vi "BRig_RT_start_v1,10__PortC.vi"() -> ()   [LabVIEW 2014]
uses:
  myRIO_BRig_RT__Case_Exp_stateList.ctl
  myRIO_BRig_RT__Case_NonExp_stateList.ctl
  <vilib>/WebDAVClient/Advanced/SessionHandle.ctl
  <vilib>/Platform/TimedLoop/XDataNode/timing_clust.ctl
  <vilib>/Platform/TimedLoop/XDataNode/nitl_modes.ctl
  <vilib>/Platform/TimedLoop/XDataNode/wakeup.ctl
  <vilib>/myRIO/Common/Instrument Driver Framework/myRIO v1.0/UART/vis/myRIO v1.0 Close UART.vi
  <vilib>/FPGAPlugInAG/myRIO-1900/niLvFpga_Open_myRIO-1900.vi
  <vilib>/rvi/interface/common/dynamic/niFpgaDynamicAddResources.vi
  <vilib>/Utility/error.llb/Error Cluster From Error Code.vi
  <vilib>/rvi/errors/niLvFpgaAdjustHostInterfaceError.vi
  <vilib>/Utility/file.llb/Read From Spreadsheet File (I64).vi
  <vilib>/Utility/file.llb/Write To Spreadsheet File (DBL).vi
  <vilib>/FPGAPlugInAG/Dynamic/niLvFpga_Close_Dynamic.vi
  <vilib>/myRIO/Common/Instrument Driver Framework/Utilities/vis/FPGA Ref Manager.vi
  <vilib>/myRIO/Common/Instrument Driver Framework/myRIO v1.0/myRIO v1.0 Reset FPGA.vi
  <vilib>/myRIO/Common/Instrument Driver Framework/myRIO v1.0/IRQ/vis/myRIO v1.0 IRQ Info FGV.vi
  <vilib>/myRIO/Common/Instrument Driver Framework/myRIO v1.0/IRQ/vis/myRIO v1.0 Timer IRQ Info FGV.vi
  <vilib>/myRIO/Common/Instrument Driver Framework/myRIO v1.0/IRQ/vis/myRIO v1.0 ISR Agent.vi
  <vilib>/rvi/interface/nirviOpenFPGA/nirviOpenFPGA.xnode
  BRig_FPGA_v3,93__PortC__build.lvbitx
  BRig_FPGA_v3,93__PortC.vi
  <vilib>/rvi/interface/nirviReadWriteControl/nirviReadWriteControl.xnode
  <vilib>/Platform/TimedLoop/XDataNode/XDataNode.xnode
  <vilib>/rvi/interface/nirviCloseFPGA/nirviCloseFPGA.xnode
  <vilib>/Platform/TimedLoop/XDataNode/XDNodeRunTimeDep.lvlib
  <vilib>/rvi/interface/Simulation/niFpgaSimulationCallBeginRW.vi
  <vilib>/myRIO/Instrument Drivers/Utilities/Utilities.lvlib
  NiFpgaLv.dll
  <vilib>/WebDAVClient/NI_WebDAV.lvlib
panel:
  out "Solenoid R":bool
  out "Solenoid L":bool
  out "Laser2":bool
  out "Laser1":bool
  out "FreeReward_c_R":u16
  out "FreeReward_c_L":u16
  in  "Laser2_LED":bool
  in  "Laser1_LED":bool
  in  "lick_Rising(F)_or_Falling(T)":bool
  out "T_ExpRun_min":dbl
  out "stop_TimedLoop":bool
  out "BTPR_avg_R":dbl
  out "T2R_avg_R":dbl
  out "BTPR_avg_L":dbl
  out "T2R_avg_L":dbl
  out "BTPR_block":u16
  out "T2R_block":u16
  in  "comm_WebDAV_connect":bool
  in  "I_sendData":bool
  in  "comm_TCP_connect":bool
  out "nRewards_total":u16 caption="# Rewards in Current Block"
  out "BUR_target":u16 caption="Target Trials Per Block"
  in  "input_Threshold_reset":bool
  out "nTrial":u16
  out "allReward_R":bool
  out "allReward_L":bool
  out "Threshold":bool
  out "tLoop":dbl format="%#_2g"
  out "L_Power_l2":dbl
  out "comm_TCP":bool
  in  "get_countPerMS":bool
  out "SolenoidReward":bool
  out "L_Power_l1":dbl caption="LaserPower"
  in  "Recording":bool
  out "FPGA_count2ms":dbl=159.0
  out "error out":errorcluster
  out "cSpout":enum16{"Left", "Right"}(ring) caption="Left or Right Spout"
  out "A4":u32 caption="LickCounter_Right"
  out "A2":u32 caption="LickCounter_Left"
  out "nRewards_Right":u16 caption="# Rewards Total (Right)"
  out "nRewards_Left":u16 caption="# Rewards Total (Left)"
  out "nRewards_cur":u16 caption="# Rewards in Current Block"
  out "TpB_target":u16 caption="Target Trials Per Block"
  out "cState_NonExp":T1 caption="WarmUp State"
  out "iBlock":u16 caption="Current Block"
  out "cState":T2 caption="Experimental State"
  out "iTrial":u16 caption="Current Trial"
  in  "Data Set Prefix":string="Exp1_TM2"
  out "comm_WebDAV":bool
  in  "Host Password":string="sabalab"
  in  "Host UserName":string="Test2"
  in  "STOP_abort":bool caption="Stop LabView\n(Stops myRio and FPGA)"
  in  "STOP_endBlock":bool caption="Stop Experiment\n@ End of Block"
  in  "STOP_endTrial":bool caption="Stop Experiment\n@ End of Trial"
  in  "START":bool caption="Start Experiment"
  # "Experimental Run"
  # "Recording Rig"
  # "FPGA Conversion\n[counts per ms]"
  # "RealTime Cycle\nShould be <5ms"
  # "STOP experiment at"
  # "Exp Run Time"
  # "Reset"
  # "min"
  # "Communication with Host"
  # "Lick Counter"
  # "Give Water?\n(Reward)"
  # "Experimental State"
  # "Left/Right"
  # "Left           Right"
  # "Direction\n(NonSpecific Licking)"
  # "Block Target"
  # "# Blocks"
  # "L          R"
  # "# Trials"
  # "# Rewards"
  # "Bad Trials\nPost Reward"
  # "Trials 2 Reward"
  # "Block"
  # "# Trials"
  # "# Rewards"
  # "Current\nBlock"
  # "WarmUp State"
  # "avg L"
  # "Total"
  # "# Rewards"
  # "# Trials"
  # "avg R"
  # "Laser Power [V]"
  # "Left           Right"
  # "FreeRewards"
  # "Laser1"
  # "Laser2"
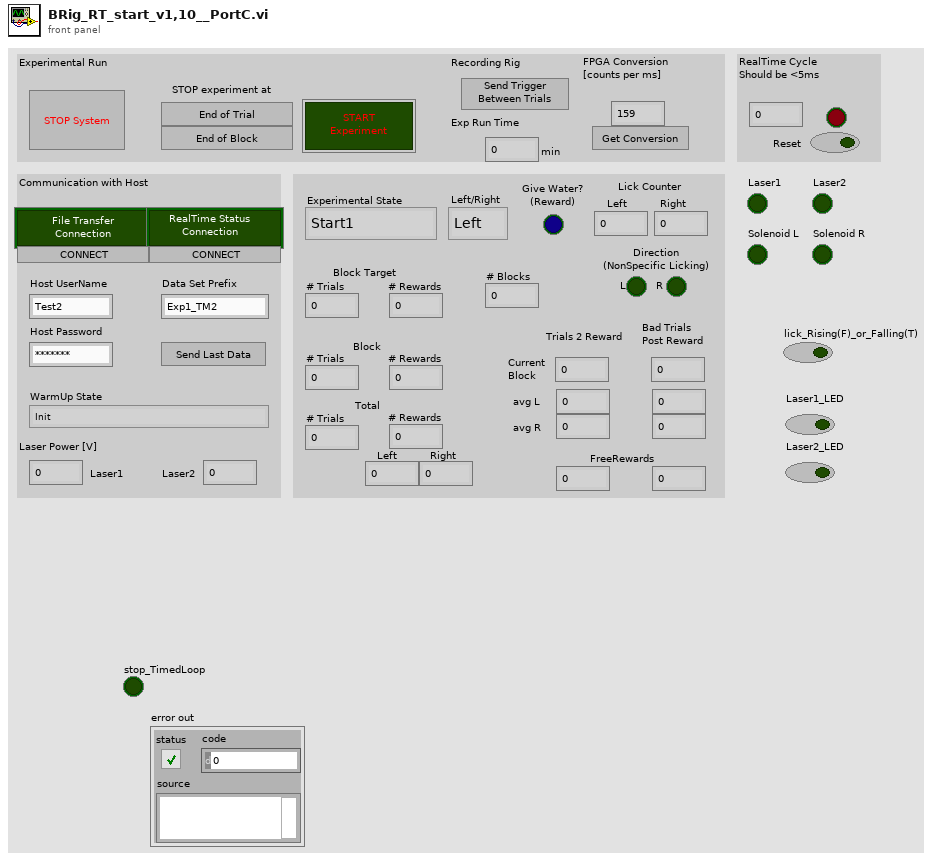
[diagram p1: front panel]
types:
  T1 = typedef "myRIO_BRig_RT__Case_NonExp_stateList.ctl" = enum16{"Init", "UploadSettings_pre", "UploadSettings_Read_dataExp", "UploadSettings_dataExp_1", "UploadSettings_dataExp_2", "UploadSettings_Read_dataLC", "UploadSettings_dataLC_1", "UploadSettings_dataLC_2", "UploadSettings_dataLC_3", "UploadSettings_dataLC_4", "UploadSettings_Read_dataMTrig", "UploadSettings_dataMTrig_1", "UploadSettings_post", "Idle_pre", "IdleEmpty", "IdleEmpty2", "IdleEmpty3", "IdleEmpty4", "Idle", "Idle_2", "Idle_3", "Idle_4", "Idle_5", "Idle_6", "Idle_post", "Cue_pre__pre", "Cue_pre", "Cue", "Cue_LED", "Cue_post", "RewardCalibration_pre", "RewardCalibration", "DispenseWater_pre__pre", "DispenseWater_pre", "DispenseWater", "DispenseWater_post", "TestConnection", "SendData", "Get_FPGA_count_per_ms", "End", "commTCP_connect"}
  T2 = typedef "myRIO_BRig_RT__Case_Exp_stateList.ctl" = enum16{"Start1", "Start2", "Start3", "saveSettings1", "saveSettings2", "saveSettings3", "saveSettings4", "saveSettings_LC_ENL_l1", "saveSettings_LC_ENL_l2", "saveSettings_LC_Cue_l1", "saveSettings_LC_Cue_l2", "saveSettings6_LC_l1_Other", "SaveSettings6_LC_l2_Other", "setSettings_Audio", "setSettings_Laser", "initBlock_pre", "initBlock", "initBlock2", "initBlock_post", "initTrial_pre", "initTrial", "initTrial2", "initTrial3", "initTrial4", "initTrial_LC_ENL1", "initTrial_LC_Cue1", "initTrial_LC_Cue1_2", "initTrial_LC_Sel", "initTrial_post", "ENL1_pre", "ENL1", "ENL1_post", "ENL1Penalty_pre", "ENL1Penalty", "ENL2_pre", "ENL2", "ENL2Penalty_pre", "ENL2Penalty", "Cue1_pre", "Cue1", "Cue1_post", "Cue1Penalty_pre", "Cue1Penalty", "Cue2_pre", "Cue2", "Cue2Penalty_pre", "Cue2Penalty", "Selection_pre", "Selection", "Select_post", "SelectReward_pre", "SelectReward", "SelectRewardPost_pre", "SelectRewardPost", "SelectWrong_pre", "SelectWrong", "SelectWrong_post", "SelectTimeout_pre", "SelectTimeout", "SelectTimeout_post", "endTrial_pre", "endTrial1", "endTrial2", "endTrial3", "endTrial_post", "endBlock_pre", "endBlock", "endBlock_post", "endExp", "commConnect", "commUpload_pre", "commUpload_dataBlock", "commUpload_dataCurrent", "commUpload_dataExp", "commUpload_dataLC", "commUpload_dataTrial", "commUpload_post", "saveData_pre", "saveData_dataBlock", "saveData_dataCurrent", "saveData_dataExp", "saveData_dataLC", "saveData_dataTrial", "saveData_post", "empty_endBlock1", "empty_endBlock2", "empty_endTrial1", "empty_endTrial2", "empty_endTrial3", "empty_endTrial4", "empty_endTrial5", "dummyState", "dummyState_endBlock", "FreeReward_pre", "FreeReward", "FreeRewardPost_pre", "FreeRewardPost"}
  T3 = enum8{"Enabled", "Disabled", "Disabled and Grayed Out"}
  T4 = typedef "NI_WebDAV.lvlib/SessionHandle.ctl" = refnum<k1>
  T5 = typedef "XDNodeRunTimeDep.lvlib/timing_clust.ctl" = cluster{"Expected End [f-1]":u64, "Actual End [f-1]":u64, "Finished Late? [f-1]":bool, "Expected End [i-1]":u64, "Actual End [i-1]":u64, "Finished Late? [i-1]":bool, "Expected Start [i]":u64, "Actual Start [i]":u64, "Expected Start [f]":u64, "Actual Start [f]":u64, "Source Name":string, "Structure Name":string, "Period":i64, "Deadline":i64, "Offset":i64, "Start":i64, "Priority":i32, "Timeout":i32, "Mode":T6, "Wakeup Reason":T7, "Error":errorcluster, "Source Type":string, "Secondary Source Type":string, "Global End Time":u64, "Global Start Time":u64, "Frame Duration":u64, "Iteration Duration":u64, "Assigned CPU":i32, "I/O Scan Engine Mode":u32}
  T6 = typedef "XDNodeRunTimeDep.lvlib/nitl_modes.ctl" = enum32{"No Change", "Process missed periods, maintain original phase", "Discard missed periods, maintain original phase", "Process missed periods, ignore original phase", "Discard missed periods, ignore original phase"}
  T7 = typedef "XDNodeRunTimeDep.lvlib/wakeup.ctl" = enum32{"Normal", "Aborted", "Asynchronous wakeup", "Timing source error", "Timed loop error", "Timeout"}
  T8 = cluster{"read mode":enum16{"polling", "blocking"}, "write mode":enum16{"polling", "blocking"}}
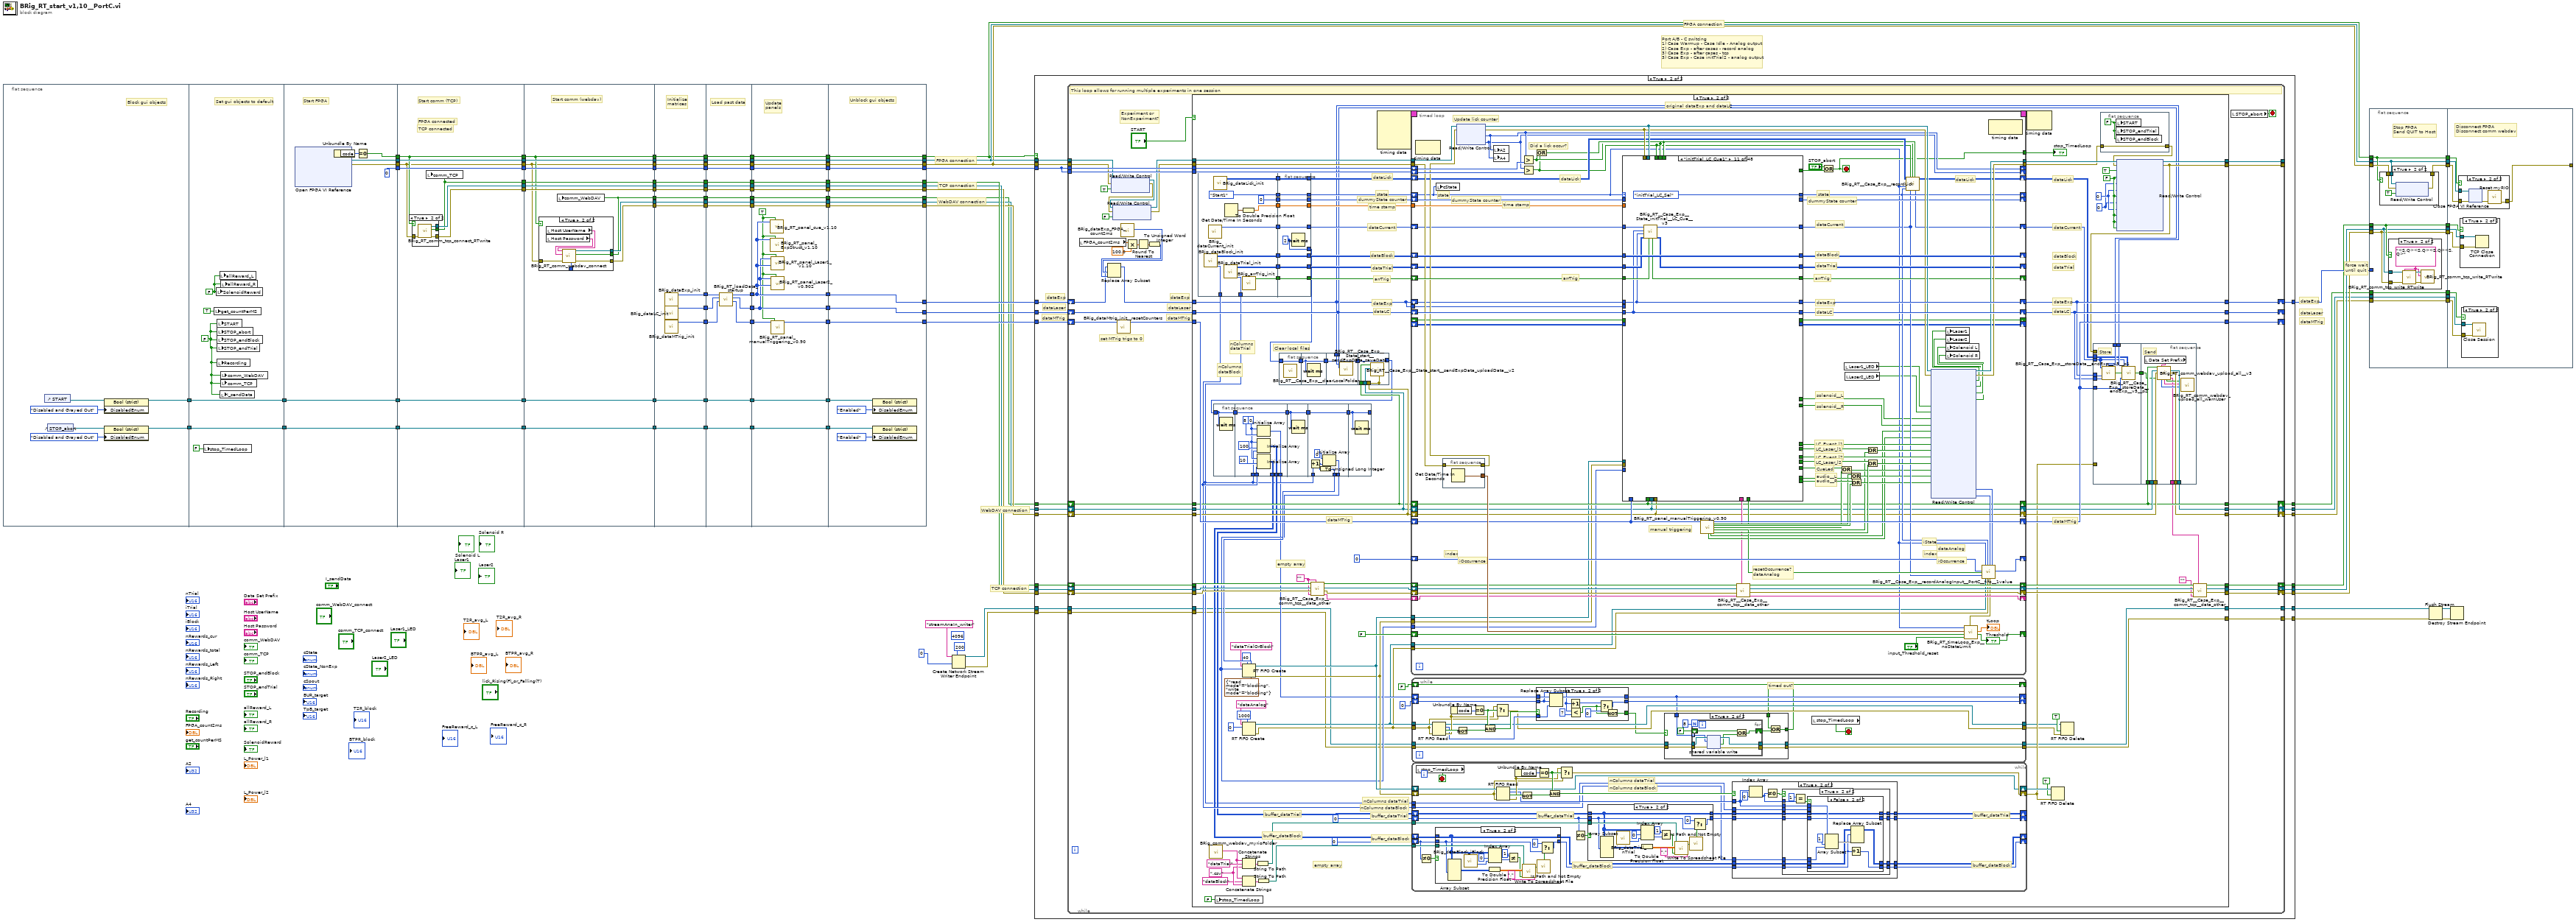
[diagram p0: block diagram]
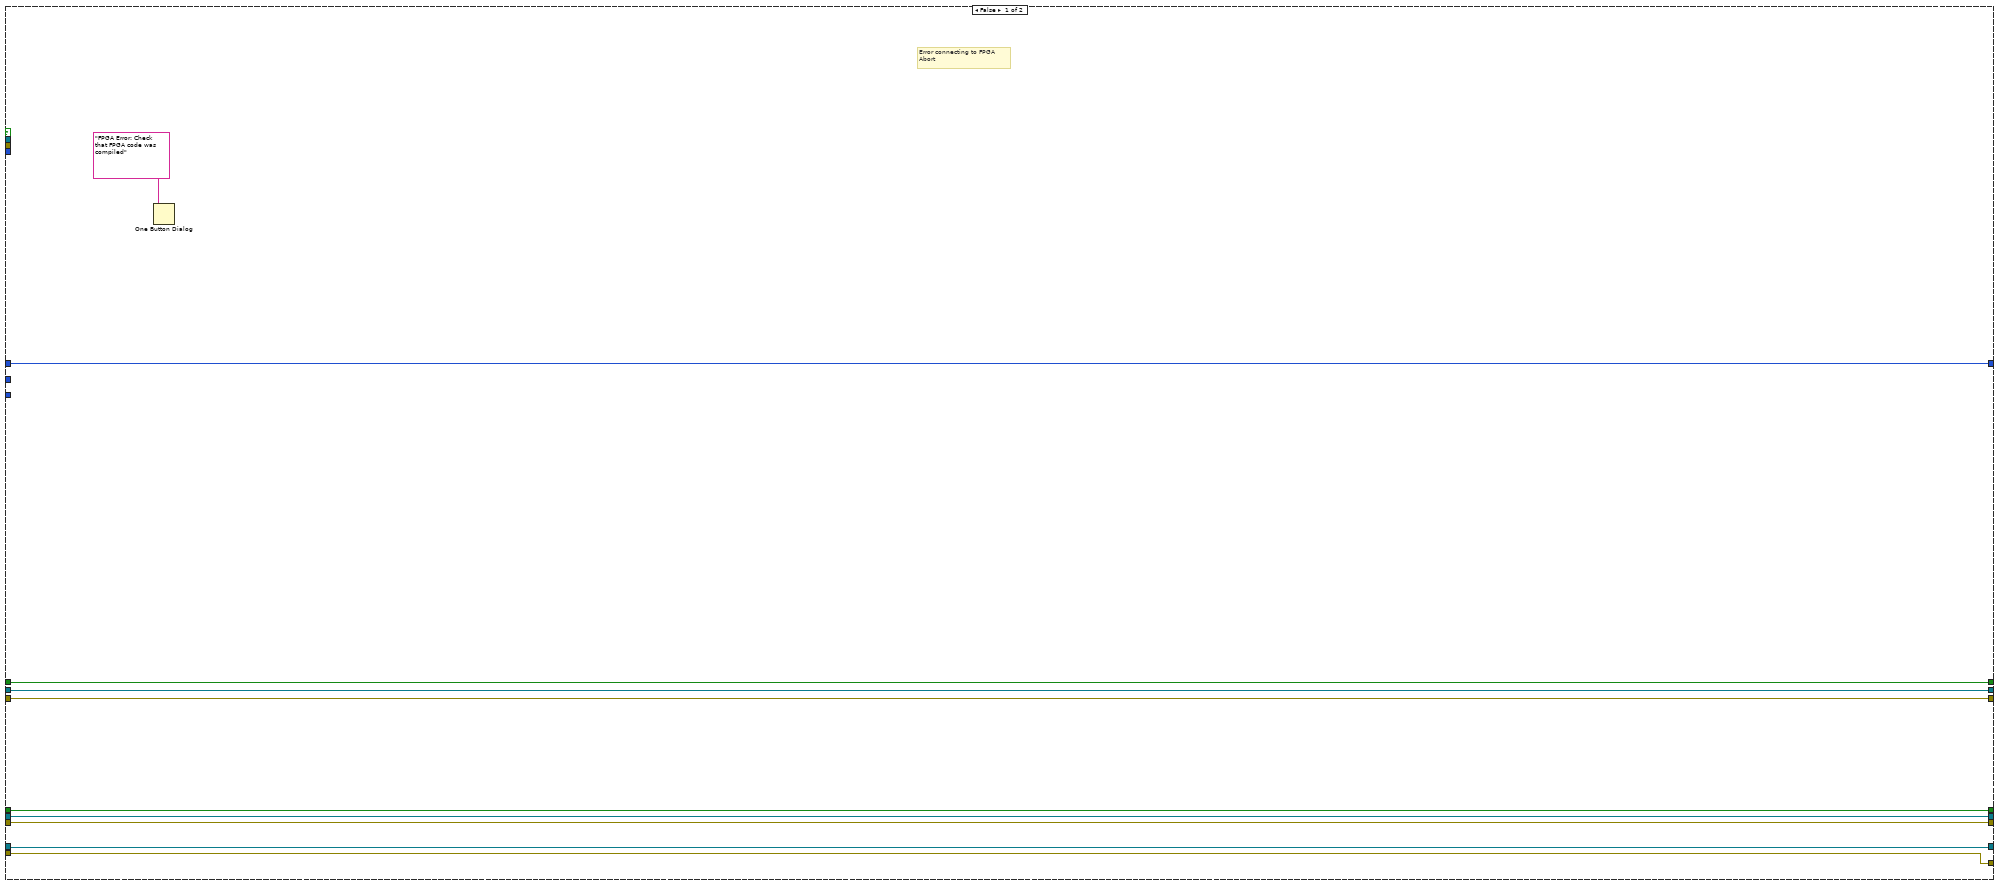
[diagram p2: hidden frame]
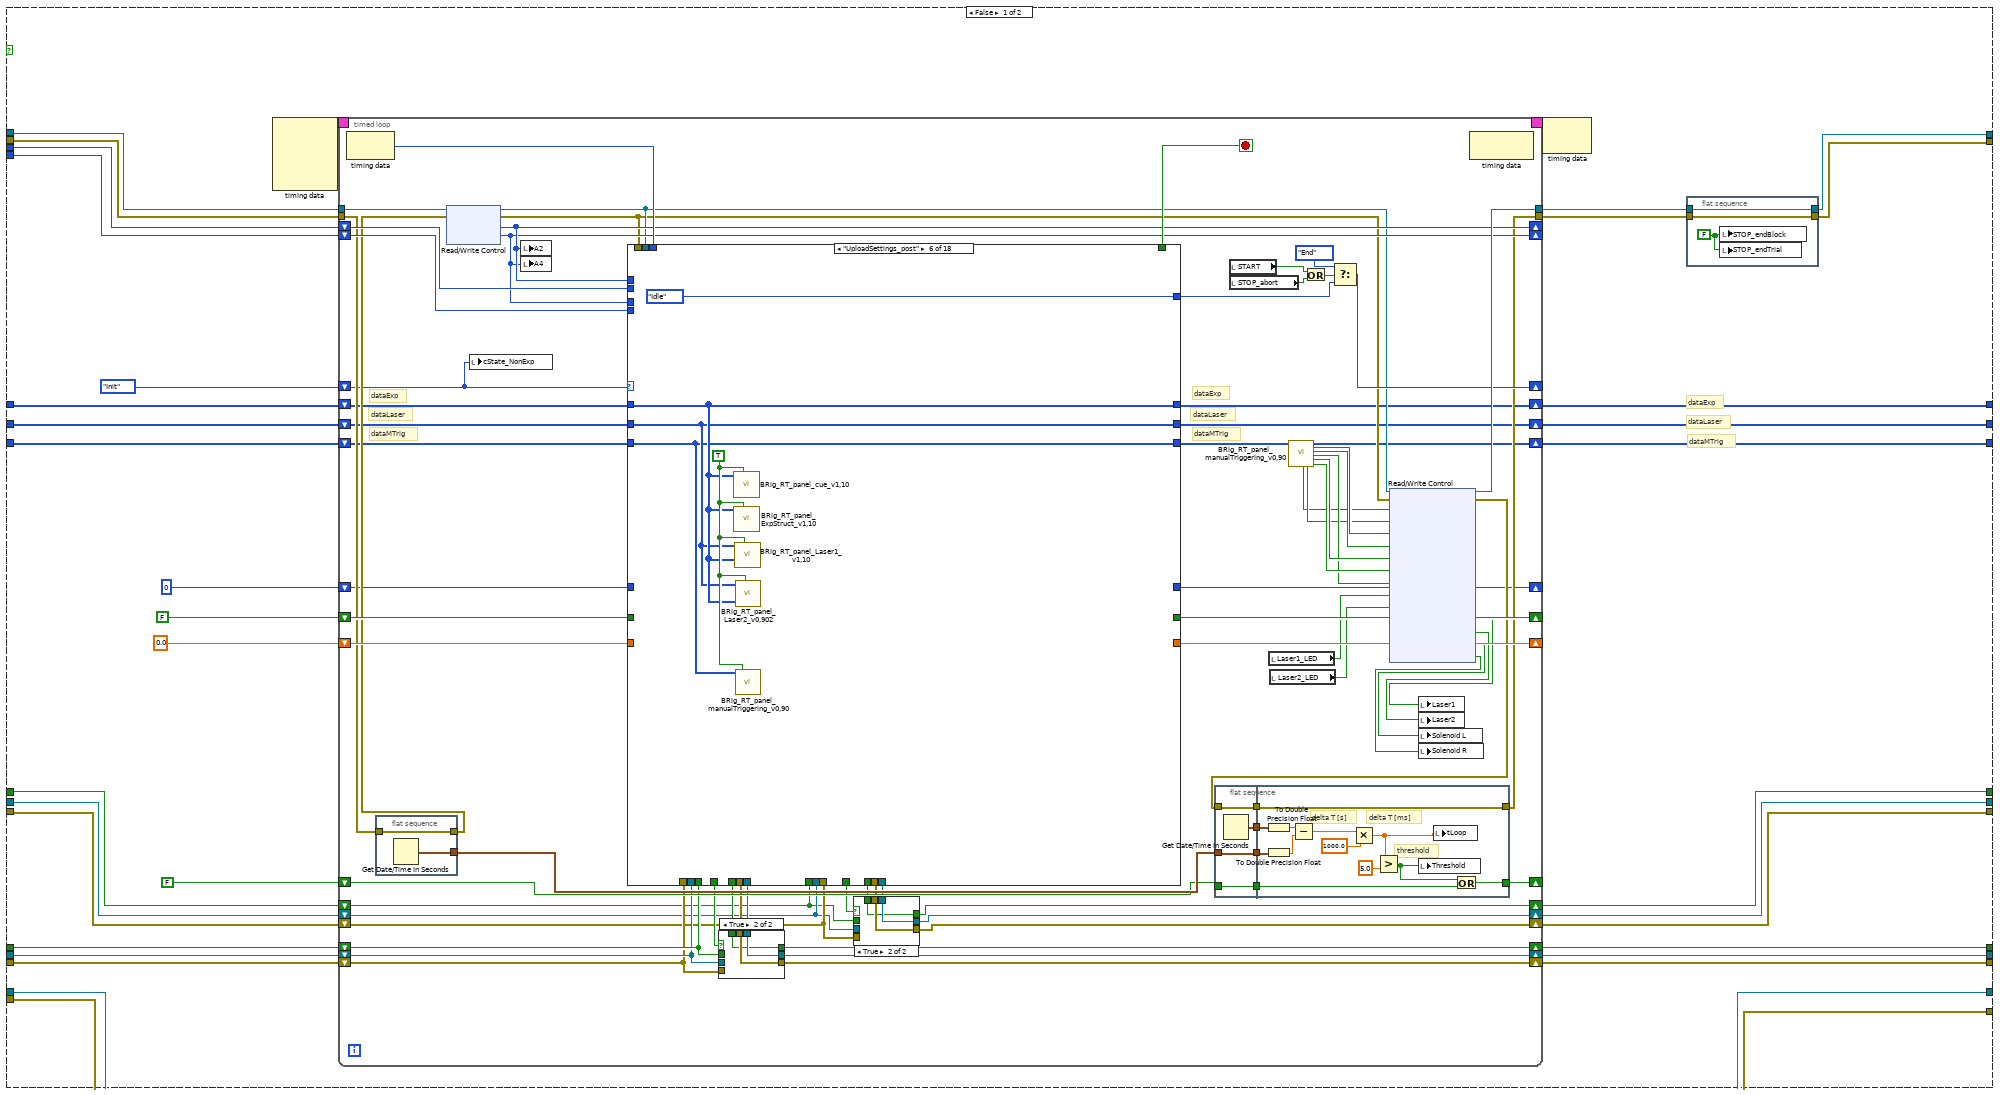
[diagram p3: hidden frame]
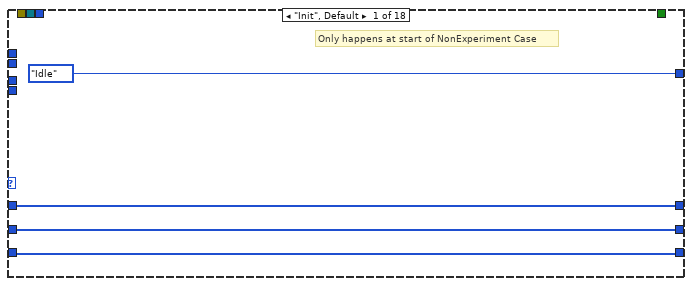
[diagram p6: hidden frame]
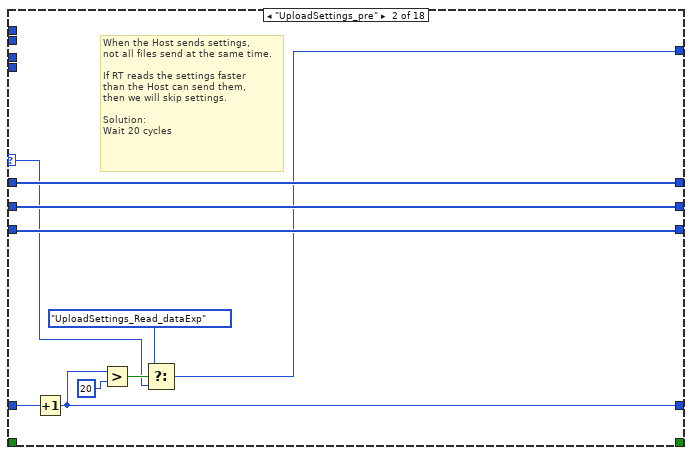
[diagram p7: hidden frame]
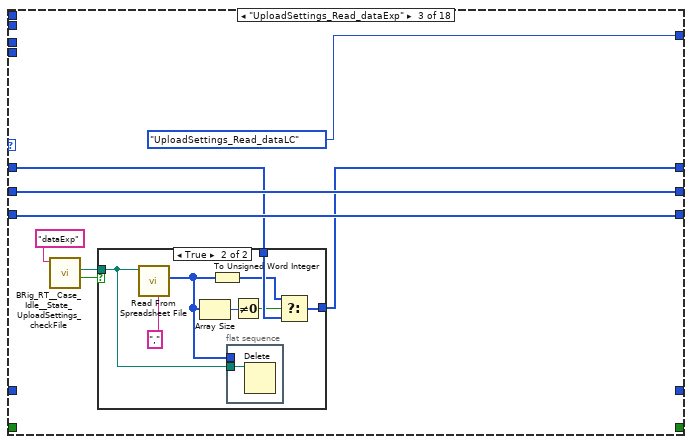
[diagram p8: hidden frame]
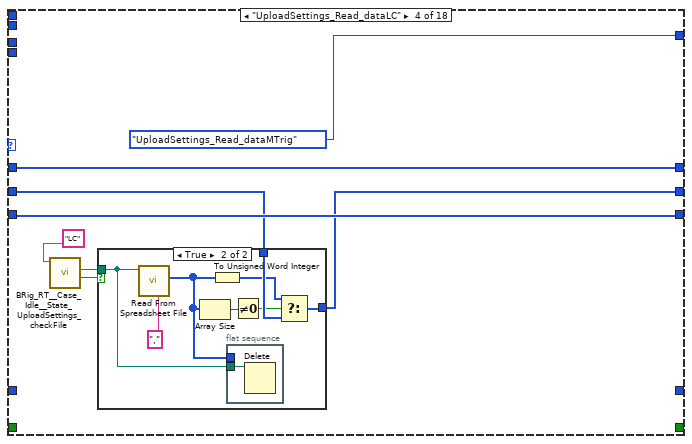
[diagram p10: hidden frame]
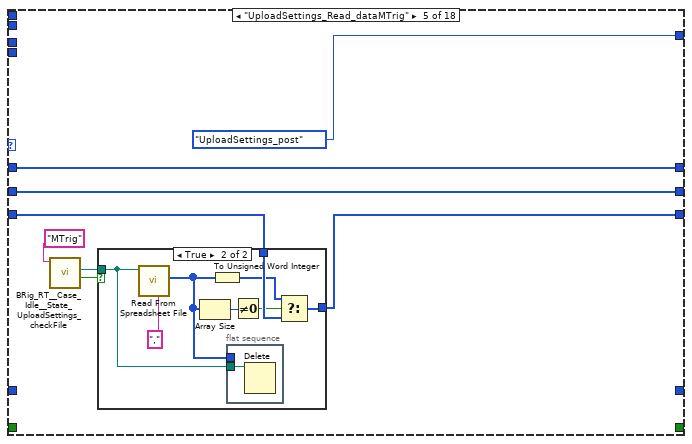
[diagram p12: hidden frame]
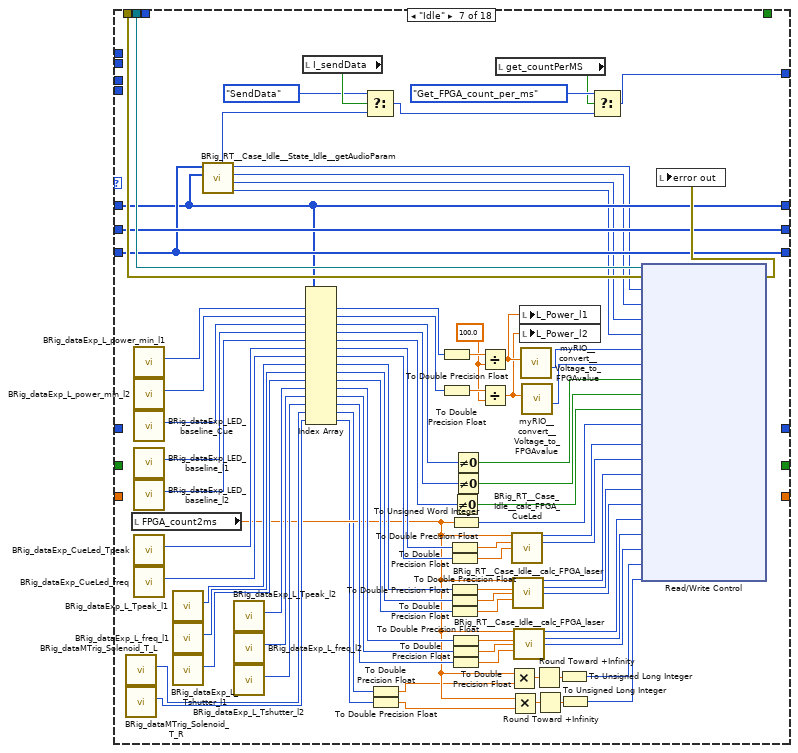
[diagram p14: hidden frame]
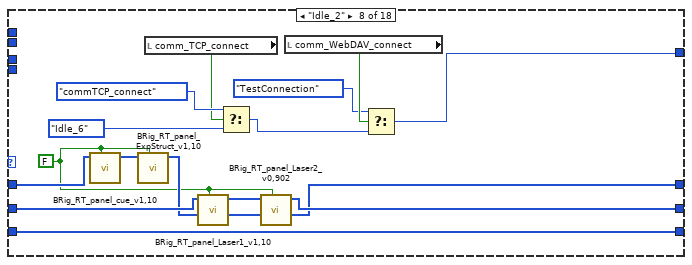
[diagram p15: hidden frame]
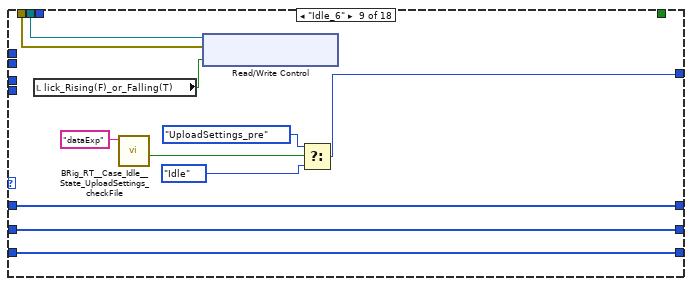
[diagram p16: hidden frame]
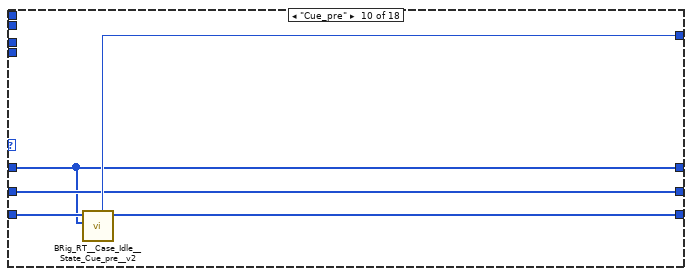
[diagram p17: hidden frame]
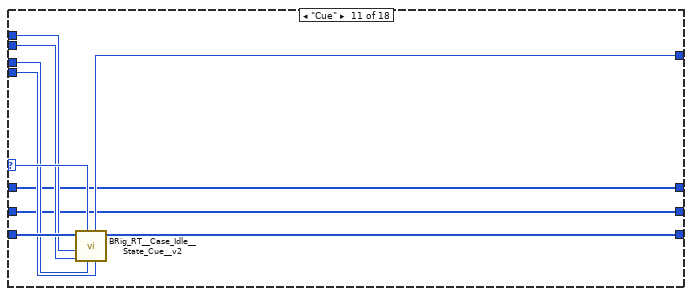
[diagram p18: hidden frame]
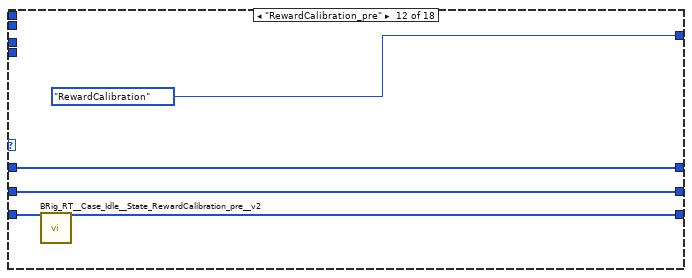
[diagram p19: hidden frame]
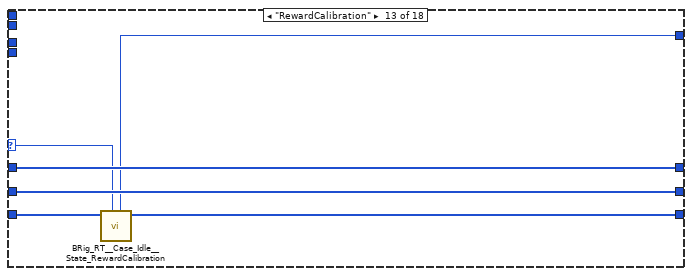
[diagram p20: hidden frame]
diagram:
  (unwired) 4096 ("reader buffer size")
  # "WebDAV connection"
  # "TCP connection"
  # "WebDAV connection"
  # "TCP connection"
  # "FPGA connection"
  # "FPGA connection"
  # "Port A/B - C switcing\n1) Case Warmup - Case Idle - Analog output\n2) Case Exp - after cases - record analog\n3) Case Exp - after cases - tcp\n3) Case Exp - Case initTrial2 - analog output"
  # "force wait\nuntil quit"
  # "dataLaser"
  # "dataExp"
  # "dataMTrig"
  n1 = flat-sequence {
    tunnel: [w116] -> w99
    tunnel: [w115] -> w95
    tunnel: [w125] -> w100
    tunnel: w99 -> [w125]
    tunnel: [w124] -> w96
    tunnel: w95 -> [w124]
    tunnel: [w131] -> w113
    tunnel: [w133] -> w112
    tunnel: [u32 0] -> w111
    tunnel: [w129] -> w110
    tunnel: [w128] -> w101
    tunnel: w100 -> [w128]
    tunnel: [w127] -> w97
    tunnel: w96 -> [w127]
    tunnel: w113 -> [w139]
    tunnel: w112 -> [w142]
    tunnel: w111 -> [w141]
    tunnel: w110 -> [w140]
    tunnel: [w139] -> w109
    tunnel: [w142] -> w108
    tunnel: [w141] -> w107
    tunnel: [w140] -> w106
    tunnel: [w134] -> w105
    tunnel: [w138] -> w104
    tunnel: [w137] -> w103
    tunnel: [w136] -> w102
    tunnel: w101 -> [w136]
    tunnel: [w135] -> w98
    tunnel: w97 -> [w135]
    tunnel: w109 -> [w153]
    tunnel: w108 -> [w161]
    tunnel: w107 -> [w160]
    tunnel: w106 -> [w154]
    tunnel: w105 -> [w159]
    tunnel: w104 -> [w158]
    tunnel: w103 -> [w157]
    tunnel: [w153] -> w66
    tunnel: [w161] -> w65
    tunnel: [w160] -> w64
    tunnel: [w154] -> w63
    tunnel: [w159] -> w62
    tunnel: [w158] -> w61
    tunnel: [w157] -> w60
    tunnel: [w156] -> w59
    tunnel: w102 -> [w156]
    tunnel: [w155] -> w58
    tunnel: w98 -> [w155]
    tunnel: [w152] -> w57
    tunnel: [w150] -> w56
    tunnel: [w151] -> w55
    tunnel: w66 -> [w186]
    tunnel: [w186] -> w54
    tunnel: w65 -> [w185]
    tunnel: [w185] -> w53
    tunnel: w64 -> [w184]
    tunnel: [w184] -> w52
    tunnel: w63 -> [w183]
    tunnel: [w183] -> w51
    tunnel: w62 -> [w182]
    tunnel: [w182] -> w50
    tunnel: w61 -> [w181]
    tunnel: [w181] -> w49
    tunnel: w60 -> [w180]
    tunnel: [w180] -> w48
    tunnel: w59 -> [w179]
    tunnel: [w179] -> w47
    tunnel: w58 -> [w178]
    tunnel: [w178] -> w46
    tunnel: w57 -> [w177]
    tunnel: [w177] -> w45
    tunnel: w56 -> [w176]
    tunnel: [w176] -> w44
    tunnel: w55 -> [w175]
    tunnel: [w175] -> w43
    tunnel: [w174] -> w42
    tunnel: [w173] -> w41
    tunnel: [w172] -> w40
    tunnel: w54 -> [w204]
    tunnel: [w204] -> w39
    tunnel: w53 -> [w203]
    tunnel: [w203] -> w37
    tunnel: w52 -> [w202]
    tunnel: [w202] -> w35
    tunnel: w51 -> [w201]
    tunnel: [w201] -> w33
    tunnel: w50 -> [w200]
    tunnel: [w200] -> w31
    tunnel: w49 -> [w199]
    tunnel: [w199] -> w29
    tunnel: w48 -> [w198]
    tunnel: [w198] -> w27
    tunnel: w47 -> [w197]
    tunnel: [w197] -> w25
    tunnel: w46 -> [w196]
    tunnel: [w196] -> w23
    tunnel: w45 -> [w195]
    tunnel: [w195] -> w21
    tunnel: w44 -> [w194]
    tunnel: [w194] -> w19
    tunnel: w43 -> [w193]
    tunnel: [w193] -> w17
    tunnel: w42 -> [w188]
    tunnel: [w187] -> w15
    tunnel: w41 -> [w190]
    tunnel: [w189] -> w13
    tunnel: w40 -> [w192]
    tunnel: [w191] -> w12
    tunnel: w39 -> [w221]
    tunnel: [w221] -> w38
    tunnel: w37 -> [w220]
    tunnel: [w220] -> w36
    tunnel: w35 -> [w219]
    tunnel: [w219] -> w34
    tunnel: w33 -> [w218]
    tunnel: [w218] -> w32
    tunnel: w31 -> [w217]
    tunnel: [w217] -> w30
    tunnel: w29 -> [w216]
    tunnel: [w216] -> w28
    tunnel: w27 -> [w215]
    tunnel: [w215] -> w26
    tunnel: w25 -> [w214]
    tunnel: [w214] -> w24
    tunnel: w23 -> [w213]
    tunnel: [w213] -> w22
    tunnel: w21 -> [w212]
    tunnel: [w212] -> w20
    tunnel: w19 -> [w211]
    tunnel: [w211] -> w18
    tunnel: w17 -> [w210]
    tunnel: [w210] -> w16
    tunnel: w15 -> [w207]
    tunnel: [w206] -> w14
    tunnel: w13 -> [w208]
    tunnel: w12 -> [w209]
    tunnel: [w209] -> w11
    tunnel: [w208] -> w10
    tunnel: [w228] -> w76
    tunnel: [w229] -> w77
    tunnel: [w230] -> w78
    tunnel: [w235] -> w82
    tunnel: [w236] -> w114
    tunnel: [w237] -> w89
    tunnel: [w238] -> w88
    tunnel: w38 -> [w238]
    tunnel: w36 -> [w237]
    tunnel: w34 -> [w236]
    tunnel: w32 -> [w235]
    tunnel: w30 -> [w230]
    tunnel: w28 -> [w229]
    tunnel: w26 -> [w228]
    tunnel: w24 -> [w232]
    tunnel: w22 -> [w231]
    tunnel: w20 -> [w226]
    tunnel: w18 -> [w227]
    tunnel: w16 -> [w225]
    tunnel: [w227] -> w70
    tunnel: [w226] -> w71
    tunnel: [w225] -> w72
    tunnel: [w222] -> w85
    tunnel: [w223] -> w84
    tunnel: [w224] -> w83
    tunnel: w14 -> [w224]
    tunnel: w11 -> [w222]
    tunnel: w10 -> [w223]
    frame #0 {
      # "Block gui objects"
      n2 = control-ref of="START"() -> (w120:refnum<vi>)
      n3 = control-ref of="STOP_abort"() -> (w117:refnum<vi>)
      n4 = property class="Bool (strict)"(reference=w120, "DisabledEnum"=T3."Disabled and Grayed Out" ("Disabled")) -> (reference out=w116:refnum<vi>)  [unwired: 1 in, 1 out]
      n5 = property class="Bool (strict)"(reference=w117, "DisabledEnum"=T3."Disabled and Grayed Out" ("Disabled")) -> (reference out=w115:refnum<vi>)  [unwired: 1 in, 1 out]
    }
    frame #1 {
      w122 = FALSE ("SolenoidReward")
      w123 = FALSE
      # "Set gui objects to default"
      n6 = local write "stop_TimedLoop"(FALSE ("stop_TimedLoop")) -> ()
      n7 = local write "get_countPerMS"(TRUE ("get_countPerMS")) -> ()
      n8 = local write "SolenoidReward"(w122) -> ()
      n9 = local write "START"(w123) -> ()
      n10 = local write "STOP_abort"(w123) -> ()
      n11 = local write "STOP_endBlock"(w123) -> ()
      n12 = local write "STOP_endTrial"(w123) -> ()
      n13 = local write "Recording"(w123) -> ()
      n14 = local write "allReward_L"(w122) -> ()
      n15 = local write "I_sendData"(w123) -> ()
      n16 = local write "comm_WebDAV"(w123) -> ()
      n17 = local write "comm_TCP"(w123) -> ()
      n18 = local write "allReward_R"(w122) -> ()
    }
    frame #2 {
      # "Start FPGA"
      n19 = xnode "Open FPGA VI Reference"() -> ("FPGA VI Reference Out"=w133:refnum<k20>, "error out"=w131:errorcluster)  [unwired: 2 in]
      n20 = Unbundle By Name(w131) -> ("code"=w130:i32)
      n21 = Equal To 0?(x=w130) -> (x = 0?=w129:bool)
    }
    frame #3 {
      # "TCP connected"
      # "Start comm (TCP)"
      # "FPGA connected"
      n22 = case shown="True" w140 {
        selector: w140 -> [w143 _]
        tunnel: w139 -> [w145 w149]
        tunnel: [refnum<k5> refnum ("output_hTCP") w148] -> w138
        tunnel: [w143 w147] -> w134
        tunnel: [w145 w146] -> w137
        frame False {
        }
        frame True {
          n23 = call "BRig_RT_comm_tcp_connect_RTwrite.vi"("input_error"=w149) -> ("output_error"=w146:errorcluster, "output_connected"=w147:bool, "output_hTCP"=w148:refnum<k5>)  [unwired: 8 in]
        }
      }
      n24 = local write "comm_TCP"(w134) -> ()
    }
    frame #4 {
      # "Start comm (webdav)"
      n25 = case shown="True" w154 {
        selector: w154 -> [w163 _]
        tunnel: [w162 w169] -> w152
        tunnel: [w163 w168] -> w150
        tunnel: w153 -> [w164 w167]
        tunnel: [w164 w166] -> w151
        tunnel: [_ w165] -> _
        frame False {
          w162 = T4 refnum items=["Session NI_WebDAV"] ("output_hSession")
        }
        frame True {
          n26 = local read "Host UserName"() -> (w170:string)
          n27 = local read "Host Password"() -> (w171:string)
          n28 = call "BRig_RT_comm_webdav_connect.vi"("input_error"=w167, "input_password"=w171, "input_username"=w170) -> ("output_error"=w166:errorcluster, "output_Iconnected"=w168:bool, "output_hSession"=w169:T4, "output_code"=w165:u8)  [unwired: 5 in]
        }
      }
      n29 = local write "comm_WebDAV"(w150) -> ()
    }
    frame #5 {
      # "Initialize\nmatrices"
      n30 = call "BRig_dataExp_init.vi"() -> ("output_dataExp"=w172:u16[])  [unwired: 11 in]
      n31 = call "BRig_dataLC_init.vi"() -> ("output_dataLC"=w173:u16[])  [unwired: 11 in]
      n32 = call "BRig_dataMTrig_init.vi"() -> ("output_dataMTrig"=w174:u16[])  [unwired: 5 in]
    }
    frame #6 {
      # "Load past data"
      n33 = call "BRig_RT_loadData_startup.vi"("input_dataMTrig"=w188, "input_dataLC"=w190, "input_dataExp"=w192) -> ("output_dataMTrig"=w187:u16[], "output_dataLC"=w189:u16[], "output_dataExp"=w191:u16[])  [unwired: 6 in]
    }
    frame #7 {
      w205 = TRUE ("input_setValues")
      # "Update\npanels"
      n34 = call "BRig_RT_panel_cue_v1,10.vi"("input_setValues"=w205, "input_dataExp"=w209) -> ()  [unwired: 9 in, 1 out]
      n35 = call "BRig_RT_panel_ExpStruct_v1,10.vi"("input_setValues"=w205, "input_dataExp"=w209) -> ()  [unwired: 9 in, 1 out]
      n36 = call "BRig_RT_panel_Laser1_v1,10.vi"("input_setValues"=w205, "input_dataExp"=w209, "input_dataLC"=w208) -> ()  [unwired: 7 in, 2 out]
      n37 = call "BRig_RT_panel_Laser2_v0,902.vi"("input_setValues"=w205, "input_dataExp"=w209, "input_dataLC"=w208) -> ()  [unwired: 7 in, 2 out]
      n38 = call "BRig_RT_panel_manualTriggering_v0,90.vi"("input_dataMTrig"=w207, "input_setValues"=w205) -> ("output_dataMTrig"=w206:u16[])  [unwired: 10 in, 7 out]
    }
    frame #8 {
      # "Unblock gui objects"
      n39 = property class="Bool (strict)"(reference=w232, "DisabledEnum"=T3."Enabled" ("Disabled")) -> ()  [unwired: 1 in, 2 out]
      n40 = property class="Bool (strict)"(reference=w231, "DisabledEnum"=T3."Enabled" ("Disabled")) -> ()  [unwired: 1 in, 2 out]
    }
  }
  n41 = Create Network Stream Writer Endpoint(7:200 ("reader buffer size"), 9:u16 0 ("element"), 11:"streamAnaIn_writer" ("reader name")) -> (0:w2:errorcluster, 3:w3:refnum<k21>)  [unwired: 4 in]
  n42 = case shown="True" w82 {
    tunnel: w114 -> [_ w271]
    tunnel: w89 -> [_ w270]
    tunnel: w88 -> [_ w269]
    tunnel: [w248 w268] -> w86
    tunnel: w85 -> [w248 w267]
    tunnel: w84 -> [_ w266]
    tunnel: w83 -> [_ w265]
    tunnel: w78 -> [w247 w264]
    tunnel: w77 -> [w246 w263]
    tunnel: w76 -> [w245 w262]
    tunnel: [w247 w261] -> w75
    tunnel: [w246 w260] -> w74
    tunnel: [w245 w259] -> w73
    tunnel: w72 -> [w244 w258]
    tunnel: w71 -> [w243 w257]
    tunnel: w70 -> [w242 w256]
    tunnel: [w244 w255] -> w69
    tunnel: [w243 w254] -> w68
    tunnel: [w242 w253] -> w67
    tunnel: [w241 w252] -> w7
    tunnel: [w240 w251] -> w6
    tunnel: w3 -> [w241 w250]
    tunnel: w2 -> [w240 w249]
    frame False {
      # "Error connecting to FPGA\nAbort"
      n43 = One Button Dialog(message="FPGA Error: Check that FPGA code was compiled") -> ()  [unwired: 1 in, 1 out]
    }
    frame True {
      # "dataExp"
      # "dataLaser"
      # "dataMTrig"
      n44 = while {
        tunnel: w270 -> [w305]
        tunnel: w269 -> [w310]
        tunnel: w271 -> [w313]
        tunnel: w271 -> [w312]
        tunnel: [w303] -> _
        tunnel: [w302] -> _
        shift-right: [w301] -> _
        shift-left: w265 -> [w297]
        shift-right: [w299] -> _
        shift-left: w266 -> [w300]
        shift-right: [w298] -> w268
        shift-left: w267 -> [w277]
        shift-right: [w292] -> w261
        shift-left: w264 -> [w295]
        shift-right: [w291] -> w260
        shift-left: w263 -> [w294]
        shift-right: [w290] -> w259
        shift-left: w262 -> [w293]
        shift-right: [w286] -> w255
        shift-left: w258 -> [w289]
        shift-right: [w285] -> w254
        shift-left: w257 -> [w288]
        shift-right: [w284] -> w253
        shift-left: w256 -> [w287]
        tunnel: [w275] -> w252
        tunnel: [w274] -> w251
        tunnel: w250 -> [w273]
        tunnel: w249 -> [w272]
        stop <- w311 stop-if-true
        # "set MTrig trigs to 0"
        # "dataExp"
        # "dataLaser"
        # "dataMTrig"
        # "Experiment or\nNonExperiment?"
        # "This loop allows for running multiple experiments in one session"
        n45 = local read "FPGA_count2ms"() -> (w281:dbl)
        n46 = xnode "Read/Write Control"("FPGA VI Reference In"=w305, "error in"=w310, "Counts_Reset"=TRUE) -> ("FPGA VI Reference Out"=w307:refnum<k20>, "error out"=w308:errorcluster)
        n47 = xnode "Read/Write Control"("FPGA VI Reference In"=w307, "error in"=w308, "Counts_Reset"=FALSE) -> ("FPGA VI Reference Out"=w304:refnum<k20>, "error out"=w306:errorcluster)
        n48 = call "BRig_dataMtrig_init__resetCounters.vi"("input_dataMTrig"=w297) -> ("output_dataMTrig"=w296:u16[])  [unwired: 10 in]
        n49 = call "BRig_dataExp_FPGA_count2ms.vi"() -> ("output_FPGA_count2ms"=w282:i32)  [unwired: 11 in]
        n50 = Multiply(x=w281, y=100.0) -> (x*y=w279:dbl)
        n51 = Round To Nearest(number=w279) -> (nearest integer value=w278:dbl)
        n52 = To Unsigned Word Integer(number=w278) -> (unsigned 16bit integer=w283:u16)
        n53 = Replace Array Subset(array=w277, new element=w283, index=w282) -> (w276:u16[])
        n54 = case shown="True" "START" {
          tunnel: w313 -> [w347 w914]
          tunnel: w312 -> [w346 w913]
          tunnel: w306 -> [w344 w902]
          tunnel: w304 -> [w345 w903]
          tunnel: [w342 w911] -> w303
          tunnel: [w340 w880] -> w302
          tunnel: w296 -> [w336 w900]
          tunnel: [w335 w886] -> w301
          tunnel: w300 -> [w334 w850]
          tunnel: w276 -> [w333 w801]
          tunnel: [w332 w885] -> w299
          tunnel: [w331 w884] -> w298
          tunnel: w295 -> [w330 w894]
          tunnel: w294 -> [w329 w893]
          tunnel: w293 -> [w328 w892]
          tunnel: [w327 w869] -> w292
          tunnel: [w326 w868] -> w291
          tunnel: [w325 w867] -> w290
          tunnel: w289 -> [w324 w849]
          tunnel: w288 -> [w323 w848]
          tunnel: w287 -> [w322 w847]
          tunnel: [w321 w876] -> w286
          tunnel: [w320 w875] -> w285
          tunnel: [w319 w877] -> w284
          tunnel: w273 -> [w317 w806]
          tunnel: w272 -> [w316 w805]
          tunnel: [w317 w804] -> w275
          tunnel: [w316 w803] -> w274
          frame False {
            # "dataExp"
            # "dataLaser"
            # "dataMTrig"
            n55 = node-c288() -> (w350:T5)  [unwired: 4 in]
            n56 = timed-loop {
              timing: w350 -> [_]
              timing-out: [_] -> w349
              shift-right: [w418] -> _
              shift-left: myRIO_BRig_RT__Case_NonExp_stateList."Init" ("Enum") -> [w387]
              shift-right: [w416] -> _
              shift-left: w347 -> [w417]
              shift-right: [w414] -> _
              shift-left: w346 -> [w415]
              tunnel: [w424] -> w343
              tunnel: [w400] -> w341
              tunnel: w344 -> [w407]
              tunnel: w345 -> [w425]
              shift-right: [w410] -> _
              shift-left: FALSE -> [w411]
              shift-right: [w408] -> _
              shift-left: 0.0 -> [w409]
              shift-right: [w397] -> _
              shift-left: FALSE -> [w398]
              shift-right: [w396] -> w335
              shift-left: w336 -> [w388]
              shift-right: [w382] -> w331
              shift-left: w333 -> [w385]
              shift-right: [w383] -> w332
              shift-left: w334 -> [w384]
              shift-right: [w381] -> w327
              shift-left: w330 -> [w377]
              shift-right: [w380] -> w326
              shift-left: w329 -> [w376]
              shift-right: [w379] -> w325
              shift-left: w328 -> [w375]
              shift-right: [w365] -> w321
              shift-left: w324 -> [w371]
              shift-right: [w366] -> w320
              shift-left: w323 -> [w370]
              shift-right: [w367] -> w319
              shift-left: w322 -> [w369]
              shift-right: [w360] -> _
              shift-left: u16 0 ("y") -> [w361]
              stop <- w427 stop-if-true
              # "dataExp"
              # "dataLaser"
              # "dataExp"
              # "dataLaser"
              # "dataMTrig"
              # "dataMTrig"
              n57 = node-c288() -> (w426:i64)  [unwired: 1 in]
              n58 = flat-sequence {
                tunnel: w407 -> [w456]
                tunnel: [w457] -> w399
                tunnel: [w456] -> w406
                frame #0 {
                  n59 = Get Date/Time In Seconds() -> (seconds since 1Jan1904=w457:timestamp)
                }
              }
              n60 = xnode "Read/Write Control"("FPGA VI Reference In"=w425, "error in"=w406) -> ("FPGA VI Reference Out"=w413:refnum<k20>, "error out"=w412:errorcluster, "A2_LickL"=w416:u32, "A4_LickR"=w414:u32)
              n61 = local write "cState_NonExp"(w387) -> ()
              n62 = local write "A2"(w416) -> ()
              n63 = local write "A4"(w414) -> ()
              n64 = case shown="\"UploadSettings_post\"" w387 {
                selector: w387 -> [_ w464 _ _ _ _ _ _ _ _ w655 _ w663 _ _ w707 w750 w756]
                tunnel: [myRIO_BRig_RT__Case_NonExp_stateList."Idle" ("Enum") w465 myRIO_BRig_RT__Case_NonExp_stateList."UploadSettings_Read_dataLC" ("t") myRIO_BRig_RT__Case_NonExp_stateList."UploadSettings_Read_dataMTrig" ("t") myRIO_BRig_RT__Case_NonExp_stateList."UploadSettings_post" ("t") myRIO_BRig_RT__Case_NonExp_stateList."Idle" ("t") w546 w614 w638 w644 w653 myRIO_BRig_RT__Case_NonExp_stateList."RewardCalibration" ("Enum") w662 myRIO_BRig_RT__Case_NonExp_stateList."Idle" ("Enum") myRIO_BRig_RT__Case_NonExp_stateList."Idle" ("Enum") w706 w750 w757] -> w419
                tunnel: [w460 w471 w479 w497 w511 w526 w558 w630 w636 w645 w654 w657 w664 w678 w690 w716 w748 w765] -> w386
                tunnel: [_ _ _ _ _ _ _ _ _ _ _ _ _ _ _ _ TRUE _] -> w427
                tunnel: w388 -> [w460 w471 w479 w497 w508 w526 w558 w630 w636 w646 w656 w658 w665 w678 w690 w716 w748 w765]
                tunnel: w426 -> [_ _ _ _ _ _ _ _ _ _ _ _ _ _ _ _ _ _]
                tunnel: w417 -> [_ _ _ _ _ _ _ _ _ _ w651 _ _ _ _ _ _ _]
                tunnel: w416 -> [_ _ _ _ _ _ _ _ _ _ w652 _ _ _ _ _ _ _]
                tunnel: w415 -> [_ _ _ _ _ _ _ _ _ _ w649 _ _ _ _ _ _ _]
                tunnel: w414 -> [_ _ _ _ _ _ _ _ _ _ w650 _ _ _ _ _ _ _]
                tunnel: w413 -> [_ _ _ _ _ _ w613 _ w633 _ _ _ _ _ _ w711 _ _]
                tunnel: w412 -> [_ _ _ _ _ _ w612 _ w632 _ _ _ _ _ _ w710 _ _]
                tunnel: w411 -> [_ _ _ _ _ _ _ _ _ _ _ _ _ _ _ w715 _ _]
                tunnel: [_ _ _ _ _ _ _ _ _ _ _ _ _ _ _ TRUE _ _] -> w410
                tunnel: w409 -> [_ _ _ _ _ _ _ _ _ _ _ _ _ _ _ w713 _ _]
                tunnel: [_ _ _ _ _ _ _ _ _ _ _ _ _ _ _ w712 _ _] -> w408
                tunnel: w385 -> [w458 w469 w474 w496 w515 w528 w557 w628 w634 w642 w647 w660 w666 w675 w687 w703 w746 w763]
                tunnel: w384 -> [w459 w470 w478 w490 w512 w527 w559 w627 w635 w643 w648 w659 w667 w676 w688 w704 w747 w764]
                tunnel: [w459 w470 w478 w493 w512 w527 w559 w623 w635 w643 w648 w659 w667 w676 w688 w704 w747 w764] -> w383
                tunnel: [w458 w469 w473 w496 w515 w528 w557 w620 w634 w642 w647 w660 w666 w675 w687 w703 w746 w763] -> w382
                tunnel: [_ _ _ _ _ _ _ _ _ _ _ _ _ _ _ _ _ TRUE] -> w378
                tunnel: w377 -> [_ _ _ _ _ _ _ _ _ _ _ _ _ _ w681 _ _ w762]
                tunnel: w376 -> [_ _ _ _ _ _ _ _ _ _ _ _ _ _ w683 _ _ w758]
                tunnel: w375 -> [_ _ _ _ _ _ _ _ _ _ _ _ _ _ w682 _ _ w761]
                tunnel: [_ _ _ _ _ _ _ _ _ _ _ _ _ _ _ _ _ w760] -> w374
                tunnel: [_ _ _ _ _ _ _ _ _ _ _ _ _ _ _ _ _ w759] -> w373
                tunnel: [_ _ _ _ _ _ _ _ _ _ _ _ _ _ _ _ _ w751] -> w372
                tunnel: w369 -> [_ _ _ _ _ _ _ _ _ _ _ _ _ _ w680 _ _ _]
                tunnel: w370 -> [_ _ _ _ _ _ _ _ _ _ _ _ _ _ w686 _ _ _]
                tunnel: w371 -> [_ _ _ _ _ _ _ _ _ _ _ _ _ w668 w685 _ _ _]
                tunnel: [_ _ _ _ _ _ _ _ _ _ _ _ _ TRUE _ _ _ _] -> w368
                tunnel: [_ _ _ _ _ _ _ _ _ _ _ _ _ w670 _ _ _ _] -> w364
                tunnel: [_ _ _ _ _ _ _ _ _ _ _ _ _ w668 _ _ _ _] -> w363
                tunnel: [_ _ _ _ _ _ _ _ _ _ _ _ _ w669 _ _ _ _] -> w362
                tunnel: w361 -> [_ w463 _ _ _ _ _ _ _ _ _ _ _ _ _ _ _ _]
                tunnel: [_ w462 _ _ _ _ _ _ _ _ _ _ _ _ _ _ _ _] -> w360
                frame "Init", Default {
                  # "Only happens at start of NonExperiment Case"
                }
                frame "UploadSettings_pre" {
                  # "When the Host sends settings,\nnot all files send at the same time.\n\nIf RT reads the settings faster\nthan the Host can send them,\nthen we will skip settings.\n\nSolution:\nWait 20 cycles"
                  n65 = Increment(x=w463) -> (x+1=w462:u16)
                  n66 = Greater?(x=w462, y=u16 20) -> (0:w467:bool)
                  n67 = Select(t=myRIO_BRig_RT__Case_NonExp_stateList."UploadSettings_Read_dataExp", s=w467, f=w464) -> (s? t:f=w465:T1)
                }
                frame "UploadSettings_Read_dataExp" {
                  n68 = call "BRig_RT__Case_Idle__State_UploadSettings_checkFile.vi"("input_dataName"="dataExp") -> ("output_Iexist"=w476:bool, "output_dataPath"=w475:path)  [unwired: 9 in]
                  n69 = case shown="True" w476 {
                    tunnel: w475 -> [_ w482]
                    tunnel: w474 -> [w480 w486]
                    tunnel: [w480 w484] -> w473
                    frame False {
                    }
                    frame True {
                      n70 = call-poly <vilib>:"Read From Spreadsheet File.vi"("delimiter (\\t)"="," ("delimiter (\\t)"), "file path (dialog if empty)"=w482) -> ("first row"=w481:i64[])  [unwired: 5 in, 4 out]
                      n71 = Array Size(array=w481) -> (size(s)=w487:i32)
                      n72 = To Unsigned Word Integer(number=w481) -> (unsigned 16bit integer=w485:u16[])
                      n73 = flat-sequence {
                        tunnel: w482 -> [w489]
                        tunnel: w481 -> [_]
                        frame #0 {
                          n74 = Delete(path (use dialog)=w489) -> ()  [unwired: 4 in, 3 out]
                        }
                      }
                      n75 = Not Equal To 0?(x=w487) -> (x != 0?=w483:bool)
                      n76 = Select(t=w485, s=w483, f=w486) -> (s? t:f=w484:u16[])
                    }
                  }
                }
                frame "UploadSettings_Read_dataLC" {
                  n77 = call "BRig_RT__Case_Idle__State_UploadSettings_checkFile.vi"("input_dataName"="LC") -> ("output_Iexist"=w491:bool, "output_dataPath"=w492:path)  [unwired: 9 in]
                  n78 = case shown="True" w491 {
                    tunnel: w492 -> [_ w500]
                    tunnel: w490 -> [w498 w504]
                    tunnel: [w498 w502] -> w493
                    frame False {
                    }
                    frame True {
                      n79 = call-poly <vilib>:"Read From Spreadsheet File.vi"("delimiter (\\t)"="," ("delimiter (\\t)"), "file path (dialog if empty)"=w500) -> ("first row"=w499:i64[])  [unwired: 5 in, 4 out]
                      n80 = Array Size(array=w499) -> (size(s)=w505:i32)
                      n81 = To Unsigned Word Integer(number=w499) -> (unsigned 16bit integer=w503:u16[])
                      n82 = flat-sequence {
                        tunnel: w500 -> [w507]
                        tunnel: w499 -> [_]
                        frame #0 {
                          n83 = Delete(path (use dialog)=w507) -> ()  [unwired: 4 in, 3 out]
                        }
                      }
                      n84 = Not Equal To 0?(x=w505) -> (x != 0?=w501:bool)
                      n85 = Select(t=w503, s=w501, f=w504) -> (s? t:f=w502:u16[])
                    }
                  }
                }
                frame "UploadSettings_Read_dataMTrig" {
                  n86 = call "BRig_RT__Case_Idle__State_UploadSettings_checkFile.vi"("input_dataName"="MTrig") -> ("output_Iexist"=w509:bool, "output_dataPath"=w510:path)  [unwired: 9 in]
                  n87 = case shown="True" w509 {
                    tunnel: w510 -> [_ w518]
                    tunnel: w508 -> [w516 w522]
                    tunnel: [w516 w520] -> w511
                    frame False {
                    }
                    frame True {
                      n88 = call-poly <vilib>:"Read From Spreadsheet File.vi"("delimiter (\\t)"="," ("delimiter (\\t)"), "file path (dialog if empty)"=w518) -> ("first row"=w517:i64[])  [unwired: 5 in, 4 out]
                      n89 = Array Size(array=w517) -> (size(s)=w523:i32)
                      n90 = To Unsigned Word Integer(number=w517) -> (unsigned 16bit integer=w521:u16[])
                      n91 = flat-sequence {
                        tunnel: w518 -> [w525]
                        tunnel: w517 -> [_]
                        frame #0 {
                          n92 = Delete(path (use dialog)=w525) -> ()  [unwired: 4 in, 3 out]
                        }
                      }
                      n93 = Not Equal To 0?(x=w523) -> (x != 0?=w519:bool)
                      n94 = Select(t=w521, s=w519, f=w522) -> (s? t:f=w520:u16[])
                    }
                  }
                }
                frame "UploadSettings_post" {
                  w529 = TRUE ("input_setValues")
                  n95 = call "BRig_RT_panel_cue_v1,10.vi"("input_setValues"=w529, "input_dataExp"=w528) -> ()  [unwired: 9 in, 1 out]
                  n96 = call "BRig_RT_panel_ExpStruct_v1,10.vi"("input_setValues"=w529, "input_dataExp"=w528) -> ()  [unwired: 9 in, 1 out]
                  n97 = call "BRig_RT_panel_Laser1_v1,10.vi"("input_setValues"=w529, "input_dataExp"=w528, "input_dataLC"=w527) -> ()  [unwired: 7 in, 2 out]
                  n98 = call "BRig_RT_panel_Laser2_v0,902.vi"("input_setValues"=w529, "input_dataExp"=w528, "input_dataLC"=w527) -> ()  [unwired: 7 in, 2 out]
                  n99 = call "BRig_RT_panel_manualTriggering_v0,90.vi"("input_dataMTrig"=w526, "input_setValues"=w529) -> ()  [unwired: 10 in, 8 out]
                }
                frame "Idle" {
                  w603 = 100.0 ("y")
                  n100 = call "BRig_dataMTrig_Solenoid_T_L.vi"() -> ("output_Solenoid_T_L"=w541:i32)  [unwired: 11 in]
                  n101 = call "BRig_dataMTrig_Solenoid_T_R.vi"() -> ("output_Solenoid_T_R"=w540:i32)  [unwired: 11 in]
                  n102 = local read "FPGA_count2ms"() -> (w539:dbl)
                  n103 = call "BRig_dataExp_L_power_min_l1.vi"() -> ("output_L_power_min_l1"=w608:i32)  [unwired: 11 in]
                  n104 = call "BRig_dataExp_L_power_min_l2.vi"() -> ("output_L_power_min_l2"=w607:i32)  [unwired: 11 in]
                  n105 = call "BRig_dataExp_LED_baseline_Cue.vi"() -> ("output_LED_baseline_Cue"=w601:i32)  [unwired: 11 in]
                  n106 = call "BRig_dataExp_LED_baseline_l1.vi"() -> ("output_LED_baseline_l1"=w600:i32)  [unwired: 11 in]
                  n107 = call "BRig_dataExp_LED_baseline_l2.vi"() -> ("output_LED_baseline_l2"=w599:i32)  [unwired: 11 in]
                  n108 = call "BRig_dataExp_CueLed_Tpeak.vi"() -> ("output_CueLed_Tpeak"=w591:i32)  [unwired: 11 in]
                  n109 = call "BRig_dataExp_CueLed_freq.vi"() -> ("output_CueLed_Freq"=w590:i32)  [unwired: 11 in]
                  n110 = call "BRig_dataExp_L_Tpeak_l1.vi"() -> ("output_L_Tpeak_l1"=w583:i32)  [unwired: 11 in]
                  n111 = call "BRig_dataExp_L_freq_l1.vi"() -> ("output_L_freq_l1"=w582:i32)  [unwired: 11 in]
                  n112 = call "BRig_dataExp_L_Tshutter_l1.vi"() -> ("output_L_Tshutter_l1"=w581:i32)  [unwired: 11 in]
                  n113 = call "BRig_RT__Case_Idle__State_Idle__getAudioParam.vi"("input_dataExp"=w557, "input_dataMTrig"=w558) -> ("output_Audio_freq_R"=w553:u8, "output_Audio_amp_R"=w554:u16, "output_Audio_freq_L"=w555:u8, "output_Audio_amp_L"=w556:u16, "output_state"=w552:T1)  [unwired: 5 in]
                  n114 = call "BRig_dataExp_L_Tpeak_l2.vi"() -> ("output_L_Tpeak_l2"=w565:i32)  [unwired: 11 in]
                  n115 = call "BRig_dataExp_L_freq_l2.vi"() -> ("output_L_freq_l2"=w564:i32)  [unwired: 11 in]
                  n116 = call "BRig_dataExp_L_Tshutter_l2.vi"() -> ("output_L_Tshutter_l2"=w563:i32)  [unwired: 11 in]
                  n117 = local read "I_sendData"() -> (w551:bool)
                  n118 = Index Array(array=w557, index #1=w608, index #2=w607, index #3=w601, index #4=w600, index #5=w599, index #6=w591, index #7=w590, index #8=w583, index #9=w582, index #10=w581, index #11=w565, index #12=w564, index #13=w563, index #14=w541, index #15=w540) -> (element #1=w606:u16, element #2=w602:u16, element #3=w598:u16, element #4=w597:u16, element #5=w596:u16, element #6=w587:u16, element #7=w586:u16, element #8=w580:u16, element #9=w579:u16, element #10=w578:u16, element #11=w568:u16, element #12=w567:u16, element #13=w566:u16, element #14=w538:u16, element #15=w537:u16)
                  n119 = Select(t=myRIO_BRig_RT__Case_NonExp_stateList."SendData" ("Enum"), s=w551, f=w552) -> (s? t:f=w548:T1)
                  n120 = To Double Precision Float(number=w538) -> (double precision float=w536:dbl)
                  n121 = To Double Precision Float(number=w537) -> (double precision float=w535:dbl)
                  n122 = To Double Precision Float(number=w606) -> (double precision float=w605:dbl)
                  n123 = To Double Precision Float(number=w602) -> (double precision float=w604:dbl)
                  n124 = To Double Precision Float(number=w587) -> (double precision float=w589:dbl)
                  n125 = To Double Precision Float(number=w586) -> (double precision float=w588:dbl)
                  n126 = To Double Precision Float(number=w580) -> (double precision float=w577:dbl)
                  n127 = To Double Precision Float(number=w579) -> (double precision float=w576:dbl)
                  n128 = To Double Precision Float(number=w578) -> (double precision float=w575:dbl)
                  n129 = To Unsigned Word Integer(number=w539) -> (unsigned 16bit integer=w592:u16)
                  n130 = To Double Precision Float(number=w568) -> (double precision float=w569:dbl)
                  n131 = To Double Precision Float(number=w567) -> (double precision float=w570:dbl)
                  n132 = To Double Precision Float(number=w566) -> (double precision float=w571:dbl)
                  n133 = Not Equal To 0?(x=w596) -> (x != 0?=w593:bool)
                  n134 = Not Equal To 0?(x=w598) -> (x != 0?=w595:bool)
                  n135 = Not Equal To 0?(x=w597) -> (x != 0?=w594:bool)
                  n136 = Divide(x=w605, y=w603) -> (x/y=w532:dbl)
                  n137 = Divide(x=w604, y=w603) -> (x/y=w531:dbl)
                  n138 = local read "get_countPerMS"() -> (w547:bool)
                  n139 = Multiply(x=w539, y=w536) -> (x*y=w545:dbl)
                  n140 = Multiply(x=w539, y=w535) -> (x*y=w543:dbl)
                  n141 = call "BRig_RT__Case_Idle__calc_FPGA_CueLed.vi"("input_FPGA_ms2count"=w539, "input_Tpeak"=w589, "input_Freq"=w588) -> ("output_laser_Npeak"=w585:u32, "output_laser_Nvalley"=w584:u32)  [unwired: 11 in]
                  n142 = call "BRig_RT__Case_Idle__calc_FPGA_laser.vi"("input_FPGA_ms2count"=w539, "input_Tpeak"=w577, "input_Freq"=w576, "input_Tshutter"=w575) -> ("output_laser_Npeak"=w574:u32, "output_laser_Nvalley"=w573:u32, "output_laser_Nshutter"=w572:u32)  [unwired: 9 in]
                  n143 = call "BRig_RT__Case_Idle__calc_FPGA_laser.vi"("input_FPGA_ms2count"=w539, "input_Tpeak"=w569, "input_Freq"=w570, "input_Tshutter"=w571) -> ("output_laser_Npeak"=w562:u32, "output_laser_Nvalley"=w561:u32, "output_laser_Nshutter"=w560:u32)  [unwired: 9 in]
                  n144 = local write "L_Power_l1"(w532) -> ()
                  n145 = local write "L_Power_l2"(w531) -> ()
                  n146 = call "myRIO__convert__Voltage_to_FPGAvalue.vi"("input_voltage"=w532) -> ("output_PortC"=w609:i16)  [unwired: 9 in, 1 out]
                  n147 = call "myRIO__convert__Voltage_to_FPGAvalue.vi"("input_voltage"=w531) -> ("output_PortC"=w610:i16)  [unwired: 9 in, 1 out]
                  n148 = Round Toward +Infinity(x=w545) -> (ceil(x): smallest int >= x=w544:dbl)
                  n149 = Round Toward +Infinity(x=w543) -> (ceil(x): smallest int >= x=w542:dbl)
                  n150 = To Unsigned Long Integer(number=w544) -> (unsigned 32bit integer=w534:u32)
                  n151 = To Unsigned Long Integer(number=w542) -> (unsigned 32bit integer=w533:u32)
                  n152 = Select(t=myRIO_BRig_RT__Case_NonExp_stateList."Get_FPGA_count_per_ms" ("Enum"), s=w547, f=w548) -> (s? t:f=w546:T1)
                  n153 = xnode "Read/Write Control"("FPGA VI Reference In"=w613, "error in"=w612, "audioAmp_L"=w556, "audioFreq_L_kHz"=w555, "audioAmp_R"=w554, "audioFreq_R_kHz"=w553, "AnaOut_0"=w609, "AnaOut_1"=w610, "CueLed_Baseline"=w595, "L1Led_Baseline"=w594, "L2Led_Baseline"=w593, "k1__counter_per_ms"=w592, "CueLed_nPeak"=w585, "CueLed_nValley"=w584, "LC_nPeak_l1"=w574, "LC_nValley_l1"=w573, "LC_nShutter_l1"=w572, "LC_nPeak_l2"=w562, "LC_nValley_l2"=w561, "LC_nShutter_l2"=w560, "Solenoid_nTotal_L"=w534, "Solenoid_nTotal_R"=w533) -> ("error out"=w611:errorcluster)  [unwired: 1 out]
                  n154 = local write "error out"(w611) -> ()
                }
                frame "Idle_2" {
                  w619 = FALSE
                  n155 = call "BRig_RT_panel_cue_v1,10.vi"("input_setValues"=w619, "input_dataExp"=w628) -> ("output_dataExp"=w629:u16[])  [unwired: 9 in]
                  n156 = call "BRig_RT_panel_ExpStruct_v1,10.vi"("input_setValues"=w619, "input_dataExp"=w629) -> ("output_dataExp"=w622:u16[])  [unwired: 9 in]
                  n157 = local read "comm_TCP_connect"() -> (w618:bool)
                  n158 = call "BRig_RT_panel_Laser1_v1,10.vi"("input_setValues"=w619, "input_dataExp"=w622, "input_dataLC"=w627) -> ("output_dataExp"=w621:u16[], "output_dataLC"=w624:u16[])  [unwired: 7 in]
                  n159 = Select(t=myRIO_BRig_RT__Case_NonExp_stateList."commTCP_connect" ("Enum"), s=w618, f=myRIO_BRig_RT__Case_NonExp_stateList."Idle_6" ("Enum")) -> (s? t:f=w616:T1)
                  n160 = call "BRig_RT_panel_Laser2_v0,902.vi"("input_setValues"=w619, "input_dataExp"=w621, "input_dataLC"=w624) -> ("output_dataExp"=w620:u16[], "output_dataLC"=w623:u16[])  [unwired: 7 in]
                  n161 = local read "comm_WebDAV_connect"() -> (w617:bool)
                  n162 = Select(t=myRIO_BRig_RT__Case_NonExp_stateList."TestConnection" ("Enum"), s=w617, f=w616) -> (s? t:f=w614:T1)
                }
                frame "Idle_6" {
                  n163 = local read "lick_Rising(F)_or_Falling(T)"() -> (w631:bool)
                  n164 = call "BRig_RT__Case_Idle__State_UploadSettings_checkFile.vi"("input_dataName"="dataExp") -> ("output_Iexist"=w640:bool)  [unwired: 9 in, 1 out]
                  n165 = xnode "Read/Write Control"("FPGA VI Reference In"=w633, "error in"=w632, "Rising(F)_or_Falling(T)"=w631) -> ()  [unwired: 2 out]
                  n166 = Select(t=myRIO_BRig_RT__Case_NonExp_stateList."UploadSettings_pre" ("Enum"), s=w640, f=myRIO_BRig_RT__Case_NonExp_stateList."Idle") -> (s? t:f=w638:T1)
                }
                frame "Cue_pre" {
                  n167 = call "BRig_RT__Case_Idle__State_Cue_pre__v2.vi"("input_dataExp"=w642, "input_dataMTrig"=w646) -> ("output_dataMTrig"=w645:u16[], "output_state"=w644:T1)  [unwired: 8 in]
                }
                frame "Cue" {
                  n168 = call "BRig_RT__Case_Idle__State_Cue__v2.vi"("input_cLick_R_prev"=w649, "input_cLick_R"=w650, "input_state"=w655, "input_cLick_L_prev"=w651, "input_cLick_L"=w652, "input_dataMTrig"=w656) -> ("output_dataMTrig"=w654:u16[], "output_state"=w653:T1)  [unwired: 4 in]
                }
                frame "RewardCalibration_pre" {
                  n169 = call "BRig_RT__Case_Idle__State_RewardCalibration_pre__v2.vi"("input_dataMTrig"=w658) -> ("output_dataMTrig"=w657:u16[])  [unwired: 26 in]
                }
                frame "RewardCalibration" {
                  n170 = call "BRig_RT__Case_Idle__State_RewardCalibration.vi"("input_state"=w663, "input_dataMTrig"=w665) -> ("output_dataMtrig"=w664:u16[], "output_state"=w662:T1)  [unwired: 8 in]
                }
                frame "TestConnection" {
                  n171 = local read "Host Password"() -> (w671:string)
                  n172 = local read "Host UserName"() -> (w672:string)
                  n173 = call "BRig_RT_comm_webdav_connect.vi"("input_password"=w671, "input_username"=w672) -> ("output_Iconnected"=w670:bool, "output_hSession"=w669:T4)  [unwired: 6 in, 2 out]
                  n174 = local write "comm_WebDAV_connect"(FALSE ("comm_WebDAV_connect")) -> ()
                  n175 = local write "comm_WebDAV"(w670) -> ()
                }
                frame "SendData" {
                  n176 = And(x=w681, y=w680) -> (x .and. y?=w679:bool)
                  n177 = case shown="True" w679 {
                    tunnel: w680 -> [_ w698]
                    tunnel: w686 -> [_ w697]
                    tunnel: w685 -> [_ w696]
                    tunnel: w683 -> [_ w694]
                    tunnel: w682 -> [_ w693]
                    frame False {
                      n178 = One Button Dialog(message="Unable to send data:\n Missing one or more\n connections") -> ()  [unwired: 1 in, 1 out]
                    }
                    frame True {
                      n179 = local read "Data Set Prefix"() -> (w699:string)
                      n180 = call "BRig_RT_comm_webdav_upload_all__v3.vi"("input_I_connected_webdav"=w698, "input_fileName_prefix"=w699, "input_hSession"=w697, "input_error"=w696, "input_True"=TRUE) -> ("output_nFilenames"=w700:i32, "output_arrFilenames"=w701:string[], "output_uploaded"=w702:bool[], "output_strCmd"=w695:string)  [unwired: 5 in, 2 out]
                      n181 = call "BRig_RT_comm_tcp_write_RTwrite.vi"("input_error"=w693, "input_packet"=w695, "input_hTCP"=w694) -> ()  [unwired: 5 in, 4 out]
                      n182 = call "BRig_RT_comm_webdav_upload_all_warnUser.vi"("input_n"=w700, "input_arrFilenames"=w701, "input_arrUploaded"=w702) -> ()  [unwired: 9 in]
                    }
                  }
                  n183 = local write "I_sendData"(FALSE ("I_sendData")) -> ()
                }
                frame "Get_FPGA_count_per_ms" {
                  # "Used to automatically determine how many FPGA cycles in 1 ms"
                  n184 = case shown="True" w715 {
                    selector: w715 -> [w717 _]
                    tunnel: w713 -> [_ w730]
                    tunnel: [w721 w730] -> w712
                    tunnel: w711 -> [w720 w728]
                    tunnel: w710 -> [w719 w727]
                    tunnel: [w718 w725] -> w705
                    tunnel: [w717 w724] -> w709
                    frame False {
                      n185 = Get Date/Time In Seconds() -> (seconds since 1Jan1904=w722:timestamp)
                      n186 = To Double Precision Float(number=w722) -> (double precision float=w721:dbl)
                      n187 = xnode "Read/Write Control"("FPGA VI Reference In"=w720, "error in"=w719, "timeTrial_trig"=TRUE ("timeTrial")) -> ("error out"=w718:errorcluster)  [unwired: 1 out]
                      n188 = local write "get_countPerMS"(w717) -> ()
                    }
                    frame True {
                      w726 = 1.0
                      n189 = Get Date/Time In Seconds() -> (seconds since 1Jan1904=w731:timestamp)
                      n190 = To Double Precision Float(number=w731) -> (double precision float=w732:dbl)
                      n191 = Subtract(x=w732, y=w730) -> (x-y=w729:dbl)
                      n192 = Less Or Equal?(x=w726, y=w729) -> (x <= y?=w724:bool)
                      n193 = case shown="True" w724 {
                        tunnel: w728 -> [_ w745]
                        tunnel: w727 -> [w733 w744]
                        tunnel: w726 -> [_ w735]
                        tunnel: [w733 w734] -> w725
                        frame False {
                        }
                        frame True {
                          n194 = xnode "Read/Write Control"("FPGA VI Reference In"=w745, "error in"=w744) -> ("FPGA VI Reference Out"=w742:refnum<k20>, "error out"=w741:errorcluster, "timeTrial_count"=w736:u32)
                          n195 = Multiply(x=w735, y=1000.0) -> (x*y=w739:dbl)
                          n196 = To Double Precision Float(number=w736) -> (double precision float=w738:dbl)
                          n197 = Divide(x=w738, y=w739) -> (x/y=w740:dbl)
                          n198 = local write "FPGA_count2ms"(w740) -> ()
                          n199 = xnode "Read/Write Control"("FPGA VI Reference In"=w742, "error in"=w741, "timeTrial_trig"=FALSE ("timeTrial")) -> ("error out"=w734:errorcluster)  [unwired: 1 out]
                        }
                      }
                    }
                  }
                  n200 = Select(t=myRIO_BRig_RT__Case_NonExp_stateList."Idle" ("Enum"), s=w709, f=w707) -> (s? t:f=w706:T1)
                  n201 = local write "error out"(w705) -> ()
                }
                frame "End" {
                }
                frame "commTCP_connect" {
                  n202 = local read "comm_TCP_connect"() -> (w755:bool)
                  n203 = case shown="True" w762 {
                    tunnel: w761 -> [w772 w781]
                    tunnel: [w771 w777] -> w759
                    tunnel: [w770 w774] -> w751
                    tunnel: [w769 w775] -> w760
                    tunnel: w758 -> [_ w782]
                    frame False {
                      n204 = call "BRig_RT_comm_tcp_connect_RTwrite.vi"("input_error"=w772) -> ("output_error"=w769:errorcluster, "output_connected"=w770:bool, "output_hTCP"=w771:refnum<k5>)  [unwired: 8 in]
                    }
                    frame True {
                      n205 = call "BRig_RT_comm_tcp_write_RTwrite.vi"("input_error"=w781, "input_packet"="<test>", "input_hTCP"=w782) -> ("output_error"=w776:errorcluster, "output_I_NotDisconnected"=w773:bool, "output_I_write"=w779:bool, "output_hTCP"=w778:refnum<k5>)  [unwired: 5 in]
                      n206 = case shown="False" w779 {
                        selector: w779 -> [_ w793]
                        tunnel: w778 -> [w788 w795]
                        tunnel: [w783 w795] -> w777
                        tunnel: w776 -> [w787 w794]
                        tunnel: [w785 w794] -> w775
                        tunnel: [w784 w793] -> w774
                        tunnel: w773 -> [w789 _]
                        frame False {
                          n207 = case shown="True" w789 {
                            tunnel: w788 -> [_ w792]
                            tunnel: w787 -> [w790 w791]
                            tunnel: [w790 w791] -> w786
                            frame False {
                            }
                            frame True {
                              n208 = TCP Close Connection(connection ID=w792, error in (no error)=w791) -> ()  [unwired: 1 in, 2 out]
                            }
                          }
                          n209 = call "BRig_RT_comm_tcp_connect_RTwrite.vi"("input_error"=w786) -> ("output_error"=w785:errorcluster, "output_connected"=w784:bool, "output_hTCP"=w783:refnum<k5>)  [unwired: 8 in]
                        }
                        frame True {
                        }
                      }
                    }
                  }
                  n210 = Not(x=w755) -> (.not. x?=w754:bool)
                  n211 = Or(x=w754, y=w751) -> (x .or. y?=w753:bool)
                  n212 = case shown="True" w753 {
                    tunnel: [w766 myRIO_BRig_RT__Case_NonExp_stateList."Idle" ("Enum")] -> w757
                    tunnel: w756 -> [w766 _]
                    frame False {
                    }
                    frame True {
                      n213 = local write "comm_TCP_connect"(FALSE) -> ()
                    }
                  }
                  n214 = local write "comm_TCP"(w751) -> ()
                }
              }
              n215 = case shown="True" w378 {
                tunnel: [w436 w437] -> w381
                tunnel: [w435 w438] -> w380
                tunnel: [w434 w439] -> w379
                tunnel: w377 -> [w436 _]
                tunnel: w376 -> [w435 _]
                tunnel: w375 -> [w434 _]
                tunnel: w374 -> [_ w439]
                tunnel: w373 -> [_ w438]
                tunnel: w372 -> [_ w437]
                frame False {
                }
                frame True {
                }
              }
              n216 = case shown="True" w368 {
                tunnel: [w430 w431] -> w367
                tunnel: [w429 w432] -> w366
                tunnel: [w428 w433] -> w365
                tunnel: w369 -> [w430 _]
                tunnel: w370 -> [w429 _]
                tunnel: w371 -> [w428 _]
                tunnel: w363 -> [_ w433]
                tunnel: w362 -> [_ w432]
                tunnel: w364 -> [_ w431]
                frame False {
                }
                frame True {
                }
              }
              n217 = flat-sequence {
                tunnel: w401 -> [w443]
                tunnel: w399 -> [w441]
                tunnel: [w443] -> w405
                tunnel: [w442] -> w404
                tunnel: [w441] -> w403
                tunnel: [w440] -> w402
                tunnel: w398 -> [w440]
                tunnel: [w455] -> w400
                tunnel: w405 -> [w455]
                tunnel: w404 -> [w454]
                tunnel: w403 -> [w452]
                tunnel: w402 -> [w447]
                tunnel: [w446] -> w397
                frame #0 {
                  n218 = Get Date/Time In Seconds() -> (seconds since 1Jan1904=w442:timestamp)
                }
                frame #1 {
                  # "threshold"
                  # "delta T [ms]"
                  # "delta T [s]"
                  n219 = To Double Precision Float(number=w454) -> (double precision float=w453:dbl)
                  n220 = To Double Precision Float(number=w452) -> (double precision float=w451:dbl)
                  n221 = Subtract(x=w453, y=w451) -> (x-y=w450:dbl)
                  n222 = Multiply(x=w450, y=1000.0) -> (x*y=w445:dbl)
                  n223 = Greater?(x=w445, y=5.0) -> (0:w444:bool)
                  n224 = local write "Threshold"(w444) -> ()
                  n225 = local write "tLoop"(w445) -> ()
                  n226 = Or(x=w444, y=w447) -> (x .or. y?=w446:bool)
                }
              }
              n227 = local read "START"() -> (w422:bool)
              n228 = local read "STOP_abort"() -> (w421:bool)
              n229 = local read "Laser1_LED"() -> (w359:bool)
              n230 = local read "Laser2_LED"() -> (w358:bool)
              n231 = call "BRig_RT_panel_manualTriggering_v0,90.vi"("input_dataMTrig"=w386) -> ("output_Solenoid_R"=w389:bool, "output_Solenoid_L"=w390:bool, "output_dataMTrig"=w396:u16[], "output_Audio_L"=w391:bool, "output_Audio_R"=w392:bool, "output_CueLed"=w393:bool, "output_Laser_l1"=w394:bool, "output_Laser_l2"=w395:bool)  [unwired: 11 in]
              n232 = Or(x=w422, y=w421) -> (x .or. y?=w420:bool)
              n233 = Select(t=myRIO_BRig_RT__Case_NonExp_stateList."End" ("Enum"), s=w420, f=w419) -> (s? t:f=w418:T1)
              n234 = xnode "Read/Write Control"("FPGA VI Reference In"=w413, "error in"=w412, "A1_SR"=w389, "A3_SL"=w390, "audioTrigger_L"=w391, "audioTrigger_R"=w392, "LC_Laser_l1"=w394, "LC_Laser_l2"=w395, "CueLed_Event"=w393, "L1Led_ON"=w359, "L2Led_ON"=w358) -> ("FPGA VI Reference Out"=w424:refnum<k20>, "error out"=w401:errorcluster, "fpga_laser1"=w354:bool, "fpga_laser2"=w355:bool, "fpga_solenoid_L"=w356:bool, "fpga_solenoid_R"=w357:bool)
              n235 = local write "Laser1"(w354) -> ()
              n236 = local write "Laser2"(w355) -> ()
              n237 = local write "Solenoid L"(w356) -> ()
              n238 = local write "Solenoid R"(w357) -> ()
              n239 = node-c288() -> ()  [unwired: 1 in, 1 out]
            }
            n240 = node-c288(w349) -> ()  [unwired: 1 out]
            n241 = flat-sequence {
              tunnel: w343 -> [w353]
              tunnel: [w353] -> w342
              tunnel: w341 -> [w352]
              tunnel: [w352] -> w340
              frame #0 {
                w351 = FALSE
                n242 = local write "STOP_endBlock"(w351) -> ()
                n243 = local write "STOP_endTrial"(w351) -> ()
              }
            }
          }
          frame True {
            w857 = ".csv" ("string")
            w887 = ""
            w896 = u8 0
            w897 = u16 0 ("AudioLeft_phase_inc")
            w898 = FALSE
            # "Clear local files"
            # "empty array"
            # "empty array"
            # "buffer_dataBlock"
            # "buffer_dataTrial"
            # "nColumns dataBlock"
            # "nColumns dataTrial"
            # "buffer_dataBlock"
            # "buffer_dataTrial"
            # "nColumns\ndataBlock"
            # "nColumns\ndataTrial"
            # "original dataExp and dataLC"
            # "dataLick"
            # "dataTrial"
            # "dataBlock"
            # "dataCurrent"
            # "arrTrig"
            # "time stamp"
            # "dummyState counter"
            # "dataTrial"
            # "dataLick"
            # "dataLC"
            # "dataLC"
            # "dataBlock"
            # "dataMTrig"
            # "dataMTrig"
            # "dataExp"
            # "dataExp"
            # "dataCurrent"
            # "state"
            n244 = flat-sequence {
              tunnel: [w994] -> w825
              tunnel: [w993] -> w830
              tunnel: [w1002] -> w844
              tunnel: [w1001] -> w843
              tunnel: [myRIO_BRig_RT__Case_Exp_stateList."Start1" ("Enum")] -> w842
              tunnel: [w999] -> w841
              tunnel: [u16 0] -> w840
              tunnel: [w997] -> w839
              tunnel: [w996] -> w838
              tunnel: [w995] -> w837
              tunnel: [w1004] -> w853
              tunnel: [w1005] -> w854
              tunnel: [w1006] -> w904
              tunnel: [w1007] -> w906
              tunnel: [w1008] -> w907
              tunnel: [w1009] -> w908
              tunnel: [w1010] -> w909
              tunnel: [w1011] -> w910
              tunnel: w844 -> [w1011]
              tunnel: w843 -> [w1010]
              tunnel: w842 -> [w1009]
              tunnel: w841 -> [w1008]
              tunnel: w840 -> [w1007]
              tunnel: w839 -> [w1006]
              tunnel: w838 -> [w1005]
              tunnel: w837 -> [w1004]
              tunnel: [w1003] -> w835
              frame #0 {
                n245 = call "BRig_dataBlock_init.vi"() -> ("output_nCol"=w993:i32, "output_dataBlock"=w995:u16[][])  [unwired: 10 in]
                n246 = call "BRig_dataCurrent_init.vi"() -> ("output_dataCurrent"=w1002:u16[])  [unwired: 11 in]
                n247 = call "BRig_dataLick_init.vi"() -> ("output_dataLick"=w1001:u16[][])  [unwired: 11 in]
                n248 = call "BRig_dataTrial_init.vi"() -> ("output_nCol"=w994:i32, "output_dataTrial"=w996:u16[][])  [unwired: 10 in]
                n249 = Get Date/Time In Seconds() -> (seconds since 1Jan1904=w992:timestamp)
                n250 = To Double Precision Float(number=w992) -> (double precision float=w999:dbl)
                n251 = call "BRig_arrTrig_init.vi"() -> ("output_arrTrig"=w997:bool[])  [unwired: 11 in]
              }
              frame #1 {
                w1003 = u32 2 ("milliseconds to wait")
                n252 = Wait (ms)(milliseconds to wait=w1003) -> ()  [unwired: 1 out]
              }
            }
            n253 = call "BRig_comm_webdav_myrioFolder.vi"() -> ("output_myrioFolder"=w858:string)  [unwired: 11 in]
            n254 = flat-sequence {
              tunnel: w832 -> [w973]
              tunnel: [w973] -> w831
              tunnel: w831 -> [w982]
              tunnel: [w980] -> w813
              tunnel: [w979] -> w829
              tunnel: [w976] -> w828
              tunnel: w830 -> [w975]
              tunnel: w825 -> [w974]
              tunnel: [w982] -> w827
              tunnel: w827 -> [w984]
              tunnel: [w984] -> w826
              tunnel: w826 -> [w990]
              tunnel: w825 -> [w989]
              tunnel: [w987] -> w820
              tunnel: [w985] -> w823
              tunnel: [w990] -> w824
              tunnel: [w991] -> _
              tunnel: w824 -> [w991]
              frame #0 {
                n255 = Wait (ms)(milliseconds to wait=w973) -> ()  [unwired: 1 out]
              }
              frame #1 {
                w977 = u16 0 ("element")
                n256 = Initialize Array(w977, 8 ("dimension size")) -> (w980:u16[])
                n257 = Initialize Array(w977, 100 ("dimension size"), w974) -> (w979:u16[][])
                n258 = Initialize Array(w977, 10 ("dimension size"), w975) -> (w976:u16[][])
              }
              frame #2 {
                n259 = Wait (ms)(milliseconds to wait=w984) -> ()  [unwired: 1 out]
              }
              frame #3 {
                n260 = Increment(x=w989) -> (x+1=w986:i32)
                n261 = To Unsigned Long Integer(number=w986) -> (unsigned 32bit integer=w985:u32)
                n262 = Initialize Array(u16 0 ("element"), w986) -> (w987:u16[])
              }
              frame #4 {
                n263 = Wait (ms)(milliseconds to wait=w991) -> ()  [unwired: 1 out]
              }
            }
            n264 = local write "stop_TimedLoop"(FALSE ("stop_TimedLoop")) -> ()
            n265 = RT FIFO Create(0:"dataTrialOrBlock" ("name (unnamed)"), 1:w820, 4:u32 40 ("size (10)"), 6:w823, 7:T8 {"read mode"=enum."blocking", "write mode"=enum."blocking"} ("r/w modes (polling,polling)")) -> (8:w822:refnum<k33>, 11:w821:errorcluster)  [unwired: 3 in, 1 out]
            n266 = RT FIFO Create(0:"dataAnalog" ("name (unnamed)"), 1:u16 0 ("element"), 4:u32 1000 ("size (10)")) -> (8:w808:refnum<k33>, 11:w807:errorcluster)  [unwired: 5 in, 1 out]
            n267 = Concatenate Strings(w858, "dataTrial" ("input_filename"), w857) -> (w859:string)
            n268 = Concatenate Strings(w858, "dataBlock" ("input_filename"), w857) -> (w860:string)
            n269 = String To Path(string=w859) -> (path=w863:path)
            n270 = String To Path(string=w860) -> (path=w855:path)
            n271 = flat-sequence {
              tunnel: [w1012] -> w836
              tunnel: w835 -> [w1012]
              tunnel: w836 -> [w1013]
              tunnel: [w1013] -> w833
              tunnel: w850 -> [w1016]
              tunnel: w801 -> [w1015]
              tunnel: [w1014] -> w834
              tunnel: w833 -> [w1014]
              tunnel: [w1020] -> _
              tunnel: w849 -> [w1020]
              tunnel: w848 -> [w1019]
              tunnel: w847 -> [w1018]
              tunnel: [w1017] -> w832
              tunnel: w834 -> [w1017]
              frame #0 {
                n272 = call "BRig_RT__Case_Exp__clearLocalFolder.vi"() -> ()  [unwired: 12 in]
              }
              frame #1 {
                n273 = Wait (ms)(milliseconds to wait=w1013) -> ()  [unwired: 1 out]
              }
              frame #2 {
                n274 = call "BRig_RT__Case_Exp__State_start__sendExpData_saveData.vi"("input_dataLC"=w1016, "input_dataExp"=w1015) -> ()  [unwired: 10 in]
              }
              frame #3 {
                n275 = call "BRig_RT__Case_Exp__State_start__sendExpData_uploadData__v2.vi"("input_error"=w1020, "input_hSession"=w1019, "input_connected"=w1018) -> ()  [unwired: 8 in, 1 out]
              }
            }
            n276 = call "BRig_RT__Case_Exp__comm_tcp__data_other.vi"("input_strState"=w887, "input_strAccum"=w887, "input_error"=w892, "input_hTCP"=w893, "input_I_connected_TCP"=w894) -> ("output_strAccum"=w888:string, "output_error"=w889:errorcluster, "output_hTCP"=w890:refnum<k5>, "output_I_connect_TCP"=w891:bool)  [unwired: 3 in]
            n277 = node-c288() -> (w916:T5)  [unwired: 4 in]
            n278 = timed-loop {
              timing: w916 -> [_]
              timing-out: [_] -> w915
              shift-right: [w1218] -> _
              shift-left: w908 -> [w1173]
              tunnel: w903 -> [w1262]
              tunnel: w902 -> [w1242]
              shift-right: [w1206] -> _
              shift-left: w914 -> [w1261]
              shift-right: [w1205] -> _
              shift-left: w913 -> [w1260]
              tunnel: [w1253] -> w895
              tunnel: [w1254] -> w912
              shift-right: [w1216] -> w883
              shift-left: w910 -> [w1190]
              shift-right: [w1259] -> w884
              shift-left: w801 -> [w1192]
              shift-right: [w1236] -> w886
              shift-left: w900 -> [w1193]
              shift-right: [w1257] -> _
              shift-left: w853 -> [w1258]
              shift-right: [w1255] -> w885
              shift-left: w850 -> [w1256]
              shift-right: [w1212] -> w882
              shift-left: w909 -> [w1219]
              shift-right: [w1252] -> _
              shift-left: w854 -> [w1191]
              tunnel: w907 -> [w1251]
              shift-right: [w1225] -> _
              shift-left: u16 0 -> [w1224]
              shift-right: [w1245] -> _
              shift-left: w906 -> [w1246]
              shift-right: [w1243] -> _
              shift-left: w904 -> [w1244]
              shift-right: [w1237] -> _
              shift-left: FALSE -> [w1239]
              shift-right: [w1181] -> w874
              shift-left: w891 -> [w1200]
              shift-right: [w1180] -> w873
              shift-left: w890 -> [w1199]
              shift-right: [w1178] -> w872
              shift-left: w889 -> [w1198]
              shift-right: [w1179] -> _
              shift-left: w888 -> [w1197]
              shift-right: [w1187] -> w879
              shift-left: w849 -> [w1187]
              shift-right: [w1189] -> w877
              shift-left: w847 -> [w1189]
              shift-right: [w1188] -> w878
              shift-left: w848 -> [w1188]
              shift-right: [w1186] -> _
              shift-left: _ -> [w1184]
              shift-right: [w1185] -> _
              shift-left: _ -> [w1183]
              tunnel: [w1182] -> w866
              tunnel: w822 -> [w1176]
              tunnel: w821 -> [w1175]
              tunnel: w820 -> [w1174]
              tunnel: w808 -> [w1172]
              tunnel: w807 -> [w1171]
              tunnel: w801 -> [w1170]
              stop <- w1182 stop-if-true
              # "iOccurrence"
              # "index"
              # "resetOccurrence?\ndataAnalog"
              # "dataLick"
              # "dataLick"
              # "dummyState counter"
              # "dummyState counter"
              # "iOccurrence"
              # "arrTrig"
              # "arrTrig"
              # "CueLed"
              # "LC_Laser_l2"
              # "LC_Event_l2"
              # "LC_Laser_l1"
              # "LC_Event_l1"
              # "iState"
              # "dataAnalog"
              # "index"
              # "manual triggering"
              # "dataTrial"
              # "dataBlock"
              # "dataExp"
              # "dataCurrent"
              # "time stamp"
              # "audio__L\naudio__R"
              # "dataLC"
              # "solenoid__R"
              # "solenoid__L"
              # "Did a lick occur?"
              # "Update lick counter"
              # "state"
              # "state"
              n279 = node-c288() -> ()  [unwired: 1 in, 1 out]
              n280 = local write "cState"(w1173) -> ()
              n281 = flat-sequence {
                tunnel: w1242 -> [w1263]
                tunnel: [w1264] -> w1240
                tunnel: [w1263] -> w1241
                frame #0 {
                  n282 = Get Date/Time In Seconds() -> (seconds since 1Jan1904=w1264:timestamp)
                }
              }
              n283 = xnode "Read/Write Control"("FPGA VI Reference In"=w1262, "error in"=w1241) -> ("FPGA VI Reference Out"=w1248:refnum<k20>, "error out"=w1247:errorcluster, "A2_LickL"=w1206:u32, "A4_LickR"=w1205:u32)
              n284 = local write "A2"(w1206) -> ()
              n285 = local write "A4"(w1205) -> ()
              n286 = Greater?(x=w1206, y=w1261) -> (0:w1214:bool)
              n287 = Greater?(x=w1205, y=w1260) -> (0:w1213:bool)
              n288 = Or(x=w1214, y=w1213) -> (x .or. y?=w1215:bool)
              n289 = case shown="\"initTrial_LC_Cue1\"" w1173 {
                selector: w1173 -> [_ _ _ _ _ _ _ _ _ _ _ _ _ _ w1477 w1493 _ w1522 _ _ w1569 w1596 _ w1622 _ w1666 _ w1706 _ w1726 _ w1764 _ w1806 _ _ _ _ w1925 _ w1949 w1980 w2001 w2026 _ w2083 w2093 _]
                tunnel: [myRIO_BRig_RT__Case_Exp_stateList."Start2" ("Enum") myRIO_BRig_RT__Case_Exp_stateList."Start3" ("Enum") myRIO_BRig_RT__Case_Exp_stateList."saveSettings1" ("Enum") myRIO_BRig_RT__Case_Exp_stateList."initBlock" ("Enum") myRIO_BRig_RT__Case_Exp_stateList."initTrial_LC_ENL1" ("Enum") myRIO_BRig_RT__Case_Exp_stateList."initTrial" ("Enum") myRIO_BRig_RT__Case_Exp_stateList."initTrial2" ("Enum") myRIO_BRig_RT__Case_Exp_stateList."setSettings_Laser" ("Enum") myRIO_BRig_RT__Case_Exp_stateList."ENL1_pre" ("Enum") myRIO_BRig_RT__Case_Exp_stateList."initTrial_LC_Cue1" ("Enum") myRIO_BRig_RT__Case_Exp_stateList."initTrial_LC_Sel" ("Enum") myRIO_BRig_RT__Case_Exp_stateList."initTrial4" ("Enum") w1455 w1466 w1475 w1491 myRIO_BRig_RT__Case_Exp_stateList."ENL1Penalty" ("Enum") w1520 w1535 w1547 w1568 w1595 myRIO_BRig_RT__Case_Exp_stateList."Cue1Penalty" ("Enum") w1623 w1639 w1661 myRIO_BRig_RT__Case_Exp_stateList."SelectReward" ("Enum") w1705 myRIO_BRig_RT__Case_Exp_stateList."SelectRewardPost" ("Enum") w1725 myRIO_BRig_RT__Case_Exp_stateList."SelectWrong" ("Enum") w1763 myRIO_BRig_RT__Case_Exp_stateList."SelectTimeout" ("Enum") w1805 myRIO_BRig_RT__Case_Exp_stateList."saveData_dataTrial" ("Enum") w1840 w1875 w1914 w1925 myRIO_BRig_RT__Case_Exp_stateList."initBlock" ("Enum") w1947 w1981 w2000 w2025 myRIO_BRig_RT__Case_Exp_stateList."FreeReward" ("Enum") w2081 w2091 myRIO_BRig_RT__Case_Exp_stateList."FreeRewardPost" ("Enum")] -> w1218
                tunnel: w1215 -> [_ _ _ _ _ _ _ _ _ _ _ _ w1456 w1467 w1476 w1492 _ _ w1536 w1548 w1570 w1597 _ _ _ _ _ _ _ _ _ _ _ _ _ _ _ _ _ _ _ _ _ _ _ _ _ _]
                tunnel: w1214 -> [_ _ _ _ _ _ _ _ _ _ _ _ _ _ _ _ _ _ _ _ _ _ _ _ w1631 w1662 _ _ _ _ _ _ _ _ _ _ _ _ _ _ _ _ _ _ _ _ _ _]
                tunnel: w1213 -> [_ _ _ _ _ _ _ _ _ _ _ _ _ _ _ _ _ _ _ _ _ _ _ _ w1630 w1663 _ _ _ _ _ _ _ _ _ _ _ _ _ _ _ _ _ _ _ _ _ _]
                tunnel: w1190 -> [w1274 w1280 w1295 w1299 w1320 w1357 w1360 w1375 w1402 w1417 w1427 w1444 w1453 w1464 w1484 w1500 w1511 w1519 w1537 w1549 w1571 w1598 w1615 w1621 w1642 w1659 w1691 w1702 w1714 w1724 w1748 w1762 w1786 w1804 w1819 w1846 w1884 w1904 w1924 w1931 w1950 w1983 w1999 w2016 w2055 w2079 w2090 w2101]
                tunnel: w1192 -> [w1265 w1279 w1285 w1297 w1308 w1356 w1370 w1376 w1413 w1416 w1426 w1436 w1460 w1471 w1487 w1503 w1510 w1527 w1534 w1546 w1574 w1601 w1608 w1629 w1638 w1658 w1693 w1704 w1712 w1731 w1744 w1769 w1781 w1811 w1829 w1838 w1882 w1889 w1923 w1928 w1952 w1985 w2011 w2031 w2036 w2084 w2094 w2100]
                tunnel: [w1274 w1280 w1295 w1299 w1320 w1355 w1359 w1378 w1402 w1420 w1434 w1443 w1457 w1468 w1483 w1499 w1512 w1518 w1531 w1543 w1554 w1581 w1614 w1620 w1637 w1660 w1684 w1707 w1713 w1722 w1741 w1760 w1779 w1803 w1821 w1846 w1884 w1904 w1924 w1931 w1950 w1983 w1999 w2016 w2061 w2080 w2089 w2099] -> w1217
                tunnel: [w1265 w1279 w1284 w1297 w1308 w1356 w1370 w1376 w1413 w1416 w1426 w1436 w1460 w1471 w1487 w1503 w1510 w1527 w1534 w1546 w1574 w1601 w1608 w1629 w1638 w1658 w1693 w1704 w1712 w1731 w1744 w1769 w1781 w1811 w1829 w1835 w1882 w1888 w1923 w1928 w1952 w1985 w2011 w2031 w2037 w2084 w2094 w2100] -> w1259
                tunnel: [_ _ _ _ _ _ _ _ _ _ _ _ _ _ _ _ _ _ _ _ _ _ _ _ _ _ _ w1696 _ _ _ _ _ _ _ _ _ _ _ _ _ _ _ _ _ w2073 _ _] -> w1202
                tunnel: [_ _ _ _ _ _ _ _ _ _ _ _ _ _ _ _ _ _ _ _ _ _ _ _ _ _ _ w1695 _ _ _ _ _ _ _ _ _ _ _ _ _ _ _ _ _ w2074 _ _] -> w1201
                tunnel: w1258 -> [w1273 w1277 w1293 w1301 w1333 w1352 w1364 w1392 w1414 w1422 w1433 w1441 w1459 w1470 w1486 w1502 w1507 w1525 w1539 w1551 w1573 w1600 w1613 w1626 w1648 w1670 w1690 w1709 w1718 w1729 w1746 w1767 w1785 w1810 w1815 w1847 w1873 w1906 w1921 w1930 w1932 w1986 w2009 w2029 w2064 w2086 w2096 w2108]
                tunnel: [w1273 w1277 w1293 w1301 w1333 w1351 w1363 w1392 w1414 w1422 w1433 w1441 w1459 w1470 w1486 w1502 w1507 w1525 w1539 w1551 w1573 w1600 w1613 w1626 w1648 w1670 w1689 w1709 w1718 w1729 w1745 w1767 w1783 w1810 w1815 w1847 w1873 w1906 w1921 w1930 w1932 w1986 w2009 w2029 w2064 w2086 w2096 w2108] -> w1257
                tunnel: w1256 -> [w1266 w1278 w1294 w1300 w1328 w1358 w1374 w1393 w1415 w1421 w1428 w1442 w1458 w1469 w1485 w1501 w1508 w1526 w1538 w1550 w1572 w1599 w1612 w1628 w1647 w1671 w1692 w1708 w1721 w1730 w1750 w1768 w1792 w1809 w1828 w1837 w1885 w1908 w1922 w1927 w1951 w1984 w2010 w2030 w2065 w2087 w2097 w2109]
                tunnel: [w1266 w1278 w1294 w1300 w1328 w1358 w1374 w1393 w1415 w1421 w1428 w1442 w1458 w1469 w1485 w1501 w1508 w1526 w1538 w1550 w1572 w1599 w1612 w1628 w1647 w1671 w1692 w1708 w1721 w1730 w1750 w1768 w1792 w1809 w1828 w1836 w1885 w1908 w1922 w1927 w1951 w1984 w2010 w2030 w2065 w2087 w2097 w2109] -> w1255
                tunnel: [_ _ _ _ _ _ _ _ _ _ _ _ _ _ _ _ _ _ _ _ _ _ _ _ _ _ _ _ _ _ _ _ _ _ _ _ _ _ TRUE _ _ _ _ _ _ _ _ _] -> w1220
                tunnel: [_ _ _ _ _ _ _ _ _ _ _ _ _ _ _ _ _ _ _ _ w1556 w1583 _ _ _ _ _ _ _ _ _ _ _ _ _ _ _ _ _ _ _ _ _ _ _ _ _ _] -> w1250
                tunnel: [_ _ _ _ _ _ _ _ _ _ _ _ _ _ _ _ _ _ _ _ w1555 w1582 _ _ _ _ _ _ _ _ _ _ _ _ _ _ _ _ _ _ _ _ _ _ _ _ _ _] -> w1249
                tunnel: w1191 -> [w1271 w1276 w1291 w1298 w1332 w1350 w1369 w1394 w1406 w1423 w1432 w1440 w1452 w1463 w1474 w1490 w1504 w1524 w1533 w1545 w1559 w1586 w1610 w1625 w1646 w1650 w1681 w1703 w1719 w1728 w1743 w1766 w1784 w1808 w1827 w1845 w1883 w1905 w1919 w1929 w1936 w1963 w2008 w2028 w2059 w2085 w2095 w2107]
                tunnel: [w1271 w1276 w1291 w1298 w1332 w1349 w1362 w1377 w1400 w1419 w1431 w1439 w1451 w1462 w1473 w1489 w1504 w1524 w1532 w1544 w1558 w1585 w1610 w1625 w1646 w1649 w1680 w1703 w1719 w1728 w1740 w1766 w1778 w1808 w1826 w1845 w1883 w1905 w1919 w1929 w1936 w1963 w2008 w2028 w2059 w2085 w2095 w2107] -> w1252
                tunnel: w1251 -> [_ _ _ _ _ _ _ _ _ _ _ _ _ _ _ _ _ _ _ _ _ _ _ _ _ _ _ _ _ _ _ _ _ _ w1820 _ _ _ _ _ _ _ _ _ _ _ _ _]
                tunnel: w1248 -> [w1270 _ _ _ w1329 w1344 w1373 w1398 w1411 _ _ w1447 _ _ _ _ _ _ _ _ w1560 w1587 _ _ w1644 w1669 w1679 _ _ _ _ _ w1790 _ w1823 _ _ _ w1917 _ _ _ _ _ w2043 _ _ _]
                tunnel: w1247 -> [w1269 _ _ _ w1330 w1343 w1361 w1397 w1410 _ _ w1446 _ _ _ _ _ _ _ _ w1561 w1588 _ _ w1645 w1668 w1678 _ _ _ _ _ w1789 _ w1822 _ _ _ w1916 _ _ _ _ _ w2042 _ _ _]
                tunnel: [_ _ _ _ _ _ _ _ _ _ _ _ _ _ w1482 w1498 _ _ _ _ w1566 w1593 _ _ w1636 w1656 _ _ _ _ _ _ _ _ _ _ _ _ _ _ _ _ _ _ _ _ _ _] -> w1226
                tunnel: [_ _ _ _ _ _ _ _ _ _ _ _ _ _ w1481 w1497 _ _ _ _ w1565 w1592 _ _ w1635 w1655 _ _ _ _ _ _ _ _ _ _ _ _ _ _ _ _ _ _ _ _ _ _] -> w1207
                tunnel: [_ _ _ _ _ _ _ _ TRUE ("Recording") _ _ _ _ _ _ _ _ _ _ _ _ _ _ _ _ _ _ _ _ _ _ _ _ _ _ _ _ _ _ _ _ _ _ _ _ _ _ _] -> w1223
                tunnel: w1246 -> [_ _ _ _ _ _ _ _ _ _ _ _ _ _ _ _ _ _ _ _ _ _ _ _ _ _ _ _ _ _ _ _ _ _ _ _ _ _ _ _ w1948 w1979 w2006 w2013 _ _ _ _]
                tunnel: [_ _ _ _ _ _ _ _ _ _ _ _ _ _ _ _ _ _ _ _ _ _ _ _ _ _ _ _ _ _ _ _ _ _ _ _ _ _ _ _ w1946 w1978 w2004 w2014 _ _ _ _] -> w1245
                tunnel: w1244 -> [_ _ _ _ w1302 _ _ _ w1407 w1424 w1430 w1438 w1454 w1465 w1478 w1494 w1505 w1523 w1530 w1542 w1567 w1594 w1609 w1624 w1632 w1657 _ _ _ _ _ _ _ _ _ _ _ _ _ _ _ _ _ _ _ _ _ _]
                tunnel: [_ _ _ _ w1302 _ _ w1379 w1407 w1418 w1429 w1437 w1454 w1465 w1478 w1494 w1505 w1523 w1529 w1541 w1567 w1594 w1609 w1624 w1632 w1657 _ _ _ _ _ _ _ _ _ _ _ _ _ _ _ _ _ _ _ _ _ _] -> w1243
                tunnel: [_ _ _ _ _ _ _ _ _ _ _ _ _ _ w1480 w1496 _ _ _ _ w1564 w1591 _ _ w1634 w1654 _ _ _ _ _ _ _ _ _ _ _ _ _ _ _ _ _ _ _ _ _ _] -> w1230
                tunnel: [_ _ _ _ _ _ _ _ _ _ _ _ _ _ w1479 w1495 _ _ _ _ w1563 w1590 _ _ w1633 w1653 _ _ _ _ _ _ _ _ _ _ _ _ _ _ _ _ _ _ _ _ _ _] -> w1231
                tunnel: [_ _ _ _ _ _ _ _ _ _ _ _ _ _ _ _ _ _ _ _ w1557 w1584 _ _ _ _ _ _ _ _ _ _ _ _ _ _ _ _ _ _ _ _ _ _ _ _ _ _] -> w1233
                tunnel: [_ _ "<S,S>" ("string") _ _ _ _ _ w1401 _ _ _ _ _ _ _ _ _ _ _ _ _ _ _ _ _ w1682 _ _ _ w1739 _ w1777 _ w1818 _ _ w1900 _ _ _ _ _ _ _ _ _ _] -> w1196
                tunnel: w1193 -> [_ _ _ _ _ _ _ _ _ _ _ _ _ _ _ _ _ _ _ _ _ _ _ _ _ _ _ _ _ _ _ _ _ _ _ _ _ _ _ _ _ _ _ _ w2050 _ _ _]
                tunnel: w1189 -> [_ _ _ _ _ _ _ _ _ _ _ _ _ _ _ _ _ _ _ _ _ _ _ _ _ _ _ _ _ _ _ _ _ _ _ _ _ w1899 _ _ _ _ _ _ _ _ _ _]
                tunnel: w1188 -> [_ _ _ _ _ _ _ _ _ _ _ _ _ _ _ _ _ _ _ _ _ _ _ _ _ _ _ _ _ _ _ _ _ _ _ _ _ _ _ _ _ _ _ _ _ _ _ _]
                tunnel: w1187 -> [_ _ _ _ _ _ _ _ _ _ _ _ _ _ _ _ _ _ _ _ _ _ _ _ _ _ _ _ _ _ _ _ _ _ _ _ _ _ _ _ _ _ _ _ _ _ _ _]
                tunnel: [_ _ _ _ _ _ _ _ _ _ _ _ _ _ _ _ _ _ _ _ _ _ _ _ _ _ _ _ _ _ _ _ _ _ _ w1839 _ _ _ _ _ _ _ _ _ _ _ _] -> w1186
                tunnel: [_ _ _ _ _ _ _ _ _ _ _ _ _ _ _ _ _ _ _ _ _ _ _ _ _ _ _ _ _ _ _ _ _ _ _ w1844 _ _ _ _ _ _ _ _ _ _ _ _] -> w1185
                tunnel: w1184 -> [_ _ _ _ _ _ _ _ _ _ _ _ _ _ _ _ _ _ _ _ _ _ _ _ _ _ _ _ _ _ _ _ _ _ _ w1843 _ _ _ _ _ _ _ _ _ _ _ _]
                tunnel: w1183 -> [_ _ _ _ _ _ _ _ _ _ _ _ _ _ _ _ _ _ _ _ _ _ _ _ _ _ _ _ _ _ _ _ _ _ _ w1834 _ _ _ _ _ _ _ _ _ _ _ _]
                tunnel: w1176 -> [_ _ _ _ _ _ _ _ _ _ _ _ _ _ _ _ _ _ _ _ _ _ _ _ _ _ _ _ _ _ _ _ _ _ _ _ _ _ _ _ w1943 w1966 _ _ _ _ _ _]
                tunnel: w1175 -> [_ _ _ _ _ _ _ _ _ _ _ _ _ _ _ _ _ _ _ _ _ _ _ _ _ _ _ _ _ _ _ _ _ _ _ _ _ _ _ _ w1942 w1965 _ _ _ _ _ _]
                tunnel: w1174 -> [_ _ _ _ _ _ _ _ _ _ _ _ _ _ _ _ _ _ _ _ _ _ _ _ _ _ _ _ _ _ _ _ _ _ _ _ _ _ _ _ w1940 w1964 _ _ _ _ _ _]
                tunnel: w1170 -> [_ _ _ _ _ _ _ _ _ _ _ _ _ _ _ _ _ _ _ _ w1553 w1580 _ _ _ _ _ _ _ _ _ _ _ _ _ _ _ w1894 _ _ _ _ _ _ _ _ _ _]
                frame "Start1", Default {
                  w1268 = FALSE ("SelectionState")
                  n290 = xnode "Read/Write Control"("FPGA VI Reference In"=w1270, "error in"=w1269, "SelectionState"=w1268, "LR_reward_Laser_l1"=w1268, "LR_wrong_Laser_l1"=w1268, "LR_reward_Event_l1"=w1268, "LR_wrong_Event_l1"=w1268, "Left(F)_or_Right(T)"=w1268, "SelectionState"=w1268, "LR_reward_Laser_l2"=w1268, "LR_wrong_laser_l2"=w1268, "LR_reward_Event_l2"=w1268, "LR_wrong_Event_l2"=w1268, "LC_Event_l1"=w1268, "LC_Laser_l1"=w1268, "LC_Laser_l2"=w1268, "LC_Event_l2"=w1268, "CueLed_Event"=w1268) -> ("error out"=w1267:errorcluster)  [unwired: 1 out]
                  n291 = local write "error out"(w1267) -> ()
                }
                frame "Start2" {
                }
                frame "Start3" {
                  w1281 = u16 0 ("new element/subarray")
                  w1286 = 0.0 ("BTPR_avg_L")
                  w1289 = FALSE ("SolenoidReward")
                  w1287 = u16 0 ("BTPR_block")
                  w1290 = u16 0 ("nRewards_cur")
                  # "Goal:\nPrepare dataCurrent"
                  n292 = call "BRig_dataExp_FreeReward_c_L.vi"() -> ("output_FreeReward_c_L"=w1283:i32)  [unwired: 11 in]
                  n293 = call "BRig_dataExp_FreeReward_c_R.vi"() -> ("output_FreeReward_c_R"=w1282:i32)  [unwired: 11 in]
                  n294 = local write "nRewards_cur"(w1290) -> ()
                  n295 = local write "nRewards_total"(w1290) -> ()
                  n296 = local write "nRewards_Left"(w1290) -> ()
                  n297 = local write "nRewards_Right"(w1290) -> ()
                  n298 = local write "BUR_target"(w1290) -> ()
                  n299 = local write "TpB_target"(w1290) -> ()
                  n300 = local write "iBlock"(w1290) -> ()
                  n301 = local write "iTrial"(w1290) -> ()
                  n302 = local write "nTrial"(w1290) -> ()
                  n303 = local write "SolenoidReward"(w1289) -> ()
                  n304 = local write "allReward_L"(w1289) -> ()
                  n305 = local write "allReward_R"(w1289) -> ()
                  n306 = Replace Array Subset(array=w1285, new element #1=w1281, index #1=w1283, new element #2=w1281, index #2=w1282) -> (w1284:u16[])
                  n307 = local write "FreeReward_c_L"(w1281) -> ()
                  n308 = local write "FreeReward_c_R"(w1281) -> ()
                  n309 = local write "BTPR_block"(w1287) -> ()
                  n310 = local write "T2R_block"(w1287) -> ()
                  n311 = local write "BTPR_avg_L"(w1286) -> ()
                  n312 = local write "BTPR_avg_R"(w1286) -> ()
                  n313 = local write "T2R_avg_L"(w1286) -> ()
                  n314 = local write "T2R_avg_R"(w1286) -> ()
                }
                frame "saveSettings1" {
                }
                frame "setSettings_Laser" {
                  n315 = call "BRig_dataExp_LED_baseline_Cue.vi"() -> ("output_LED_baseline_Cue"=w1317:i32)  [unwired: 11 in]
                  n316 = call "BRig_dataExp_LED_baseline_l1.vi"() -> ("output_LED_baseline_l1"=w1318:i32)  [unwired: 11 in]
                  n317 = call "BRig_dataExp_LED_baseline_l2.vi"() -> ("output_LED_baseline_l2"=w1316:i32)  [unwired: 11 in]
                  n318 = call "BRig_dataExp_I_anySelect.vi"() -> ("output_I_anySelect"=w1310:i32)  [unwired: 11 in]
                  n319 = call "BRig_dataExp_I_trialUntilReward.vi"() -> ("output_I_trialUntilReward"=w1309:i32)  [unwired: 11 in]
                  n320 = local read "FPGA_count2ms"() -> (w1327:dbl)
                  n321 = call "BRig_RT__Case_Exp__State_setLaserSettings.vi"("input_FPGA_count2ms"=w1327, "input_dataExp"=w1308, "input_dataLC"=w1328) -> ("output_LR_nTotal_l1"=w1326:u32, "output_LR_nTotal_l2"=w1325:u32, "output_LR_reward_nDelay_l1"=w1324:u32, "output_LR_wrong_nDelay_l1"=w1323:u32, "output_LR_reward_nDelay_l2"=w1322:u32, "output_LR_wrong_nDelay_l2"=w1321:u32)  [unwired: 11 in]
                  n322 = Index Array(array=w1308, index #1=w1317, index #2=w1318, index #3=w1316, index #4=w1310, index #5=w1309) -> (element #1=w1315:u16, element #2=w1314:u16, element #3=w1313:u16, element #4=w1312:u16, element #5=w1311:u16)
                  n323 = Not Equal To 0?(x=w1314) -> (x != 0?=w1306:bool)
                  n324 = Not Equal To 0?(x=w1312) -> (x != 0?=w1304:bool)
                  n325 = Not Equal To 0?(x=w1315) -> (x != 0?=w1307:bool)
                  n326 = Not Equal To 0?(x=w1313) -> (x != 0?=w1305:bool)
                  n327 = Not Equal To 0?(x=w1311) -> (x != 0?=w1303:bool)
                  n328 = xnode "Read/Write Control"("FPGA VI Reference In"=w1329, "error in"=w1330, "LR_reward_nTotal_l1"=w1326, "LR_wrong_nTotal_l1"=w1326, "LR_reward_nTotal_l2"=w1325, "LR_wrong_nTotal_l2"=w1325, "LR_reward_nDelay_l1"=w1324, "LR_wrong_nDelay_l1"=w1323, "LR_reward_nDelay_l2"=w1322, "LR_wrong_nDelay_l2"=w1321, "CueLed_Baseline"=w1307, "L1Led_Baseline"=w1306, "L2Led_Baseline"=w1305, "I_allReward"=w1304, "ignoreWrong"=w1303) -> ("error out"=→"error out":errorcluster)  [unwired: 1 out]
                }
                frame "initBlock" {
                  w1334 = u16 0 ("BTPR_block")
                  n329 = local write "nRewards_cur"(u16 0 ("nRewards_cur")) -> ()
                  n330 = local write "BTPR_block"(w1334) -> ()
                  n331 = local write "T2R_block"(w1334) -> ()
                  n332 = call "BRig_RT__Case_Exp__State_initBlock.vi"("input_dataCurrent"=w1357, "input_dataExp"=w1356, "input_dataBlock"=w1352, "input_dataTrial"=w1350) -> ("output_iSpout"=w1341:u16, "output_speaker_amp_R"=w1345:u16, "output_iBlock"=w1340:u16, "output_speaker_freq_R"=w1346:u8, "output_BUR_target"=w1339:u16, "output_speaker_amp_L"=w1347:u16, "output_TpB_target"=w1354:u16, "output_speaker_freq_L"=w1348:u8, "output_dataCurrent"=w1355:u16[], "output_dataBlock"=w1351:u16[][], "output_dataTrial"=w1349:u16[][])  [unwired: 5 in]
                  n333 = Type Cast(type=enum16{"Left", "Right"}."Left", x=w1341) -> (*(type *) &x=w1336:enum16{"Left", "Right"})
                  n334 = Not Equal To 0?(x=w1341) -> (x != 0?=w1335:bool)
                  n335 = local write "cSpout"(w1336) -> ()
                  n336 = local write "iBlock"(w1340) -> ()
                  n337 = local write "BUR_target"(w1339) -> ()
                  n338 = local write "TpB_target"(w1354) -> ()
                  n339 = xnode "Read/Write Control"("FPGA VI Reference In"=w1344, "error in"=w1343, "Left(F)_or_Right(T)"=w1335, "audioFreq_L_kHz"=w1348, "audioAmp_L"=w1347, "audioFreq_R_kHz"=w1346, "audioAmp_R"=w1345) -> ("error out"=w1342:errorcluster)  [unwired: 1 out]
                  n340 = local write "error out"(w1342) -> ()
                }
                frame "initTrial" {
                  n341 = xnode "Read/Write Control"("FPGA VI Reference In"=w1373, "error in"=w1361, "SelectionState"=FALSE) -> ("error out"=w1372:errorcluster)  [unwired: 1 out]
                  n342 = call "BRig_RT__Case_Exp__State_initTrial__v3.vi"("input_dataCurrent"=w1360, "input_dataBlock"=w1364, "input_dataTrial"=w1369, "input_dataExp"=w1370) -> ("output_iTrial"=w1367:u16, "output_nTrial"=w1365:u16, "output_SolenoidReward"=w1368:bool, "output_dataCurrent"=w1359:u16[], "output_dataBlock"=w1363:u16[][], "output_dataTrial"=w1362:u16[][])  [unwired: 6 in]
                  n343 = local write "iTrial"(w1367) -> ()
                  n344 = local write "nTrial"(w1365) -> ()
                  n345 = local write "SolenoidReward"(w1368) -> ()
                  n346 = local write "error out"(w1372) -> ()
                }
                frame "initTrial2" {
                  n347 = call "BRig_RT__Case_Exp__State_initTrial2__v3.vi"("input_dataCurrent"=w1375, "input_dataTrial"=w1394, "input_dataExp"=w1376, "input_dataBlock"=w1392, "input_dataLC"=w1393) -> ("output_L_Wrong_Laser_l2"=w1384:bool, "output_L_Wrong_Event_l2"=w1385:bool, "output_L_Power_l1"=w1383:dbl, "output_L_Reward_Laser_l2"=w1386:bool, "output_L_Power_l2"=w1382:dbl, "output_L_Reward_Event_l2"=w1387:bool, "output_dataCurrent"=w1378:u16[], "output_dataTrial"=w1377:u16[][], "output_L_Reward_Event_l1"=w1391:bool, "output_L_Reward_Laser_l1"=w1390:bool, "output_L_Wrong_Event_l1"=w1389:bool, "output_L_Wrong_Laser_l1"=w1388:bool)  [unwired: 3 in]
                  n348 = local write "L_Power_l1"(w1383) -> ()
                  n349 = call "myRIO__convert__Voltage_to_FPGAvalue.vi"("input_voltage"=w1383) -> ("output_PortC"=w1380:i16)  [unwired: 9 in, 1 out]
                  n350 = local write "L_Power_l2"(w1382) -> ()
                  n351 = call "myRIO__convert__Voltage_to_FPGAvalue.vi"("input_voltage"=w1382) -> ("output_PortC"=w1381:i16)  [unwired: 9 in, 1 out]
                  n352 = xnode "Read/Write Control"("FPGA VI Reference In"=w1398, "error in"=w1397, "AnaOut_0"=w1380, "AnaOut_1"=w1381, "LR_reward_Event_l1"=w1391, "LR_reward_Laser_l1"=w1390, "LR_wrong_Event_l1"=w1389, "LR_wrong_Laser_l1"=w1388, "LR_reward_Event_l2"=w1387, "LR_reward_Laser_l2"=w1386, "LR_wrong_Event_l2"=w1385, "LR_wrong_laser_l2"=w1384) -> ("error out"=w1395:errorcluster)  [unwired: 1 out]
                  n353 = local write "error out"(w1395) -> ()
                  n354 = call "BRig_arrTrig_init.vi"() -> ("output_arrTrig"=w1379:bool[])  [unwired: 11 in]
                }
                frame "initTrial4" {
                  # "resetOccurrence?\ndataAnalog"
                  n355 = local read "FPGA_count2ms"() -> (w1403:dbl)
                  n356 = local read "lick_Rising(F)_or_Falling(T)"() -> (w1399:bool)
                  n357 = local read "Recording"() -> (w1405:bool)
                  n358 = call "BRig_RT_comm_tcp_write_RTwrite__RunState_Trial_start.vi"("input_dataCurrent"=w1402) -> ("output_strCmd"=w1401:string)  [unwired: 10 in]
                  n359 = call "BRig_RT__Case_Exp__State_initTrial4.vi"("input_Recording"=w1405, "input_FPGA_count2ms"=w1403, "input_dataTrial"=w1406) -> ("output_Solenoid_nTotal"=w1404:u32, "output_dataTrial"=w1400:u16[][])  [unwired: 7 in]
                  n360 = xnode "Read/Write Control"("FPGA VI Reference In"=w1411, "error in"=w1410, "Solenoid_nTotal_L"=w1404, "Solenoid_nTotal_R"=w1404, "A6_Act"=w1405, "Rising(F)_or_Falling(T)"=w1399) -> ("error out"=w1409:errorcluster)  [unwired: 1 out]
                  n361 = local write "error out"(w1409) -> ()
                }
                frame "initTrial_LC_ENL1" {
                  n362 = call "BRig_RT__Case_Exp__State_initTrial__LC_ENL__v3.vi"("input_arrTrig"=w1424, "input_dataTrial"=w1423, "input_dataExp"=w1416, "input_dataLC"=w1421, "input_dataCurrent"=w1417) -> ("output_dataTrial"=w1419:u16[][], "output_dataCurrent"=w1420:u16[], "output_arrTrig"=w1418:bool[])  [unwired: 4 in]
                }
                frame "initTrial_LC_Cue1" {
                  n363 = call "BRig_RT__Case_Exp__State_initTrial__LC_Cue__v3.vi"("input_arrTrig"=w1430, "input_dataTrial"=w1432, "input_dataExp"=w1426, "input_dataLC"=w1428, "input_dataCurrent"=w1427) -> ("output_dataTrial"=w1431:u16[][], "output_dataCurrent"=w1434:u16[], "output_arrTrig"=w1429:bool[])  [unwired: 4 in]
                }
                frame "initTrial_LC_Sel" {
                  n364 = call "BRig_RT__Case_Exp__State_initTrial__LC_Select.vi"("input_arrTrig"=w1438, "input_dataTrial"=w1440, "input_dataExp"=w1436, "input_dataLC"=w1442, "input_dataCurrent"=w1444) -> ("output_dataTrial"=w1439:u16[][], "output_dataCurrent"=w1443:u16[], "output_arrTrig"=w1437:bool[])  [unwired: 4 in]
                  n365 = xnode "Read/Write Control"("FPGA VI Reference In"=w1447, "error in"=w1446, "A6_Act"=FALSE) -> ("error out"=w1448:errorcluster)  [unwired: 1 out]
                  n366 = local write "error out"(w1448) -> ()
                }
                frame "ENL1_pre" {
                  n367 = call "BRig_RT__Case_Exp__State_ENLPre__v3.vi"("input_ENL2"=FALSE, "input_I_lick"=w1456, "input_dataTrial"=w1452, "input_dataCurrent"=w1453) -> ("output_dataTrial"=w1451:u16[][], "output_dataCurrent"=w1457:u16[], "output_state"=w1455:T2)  [unwired: 5 in]
                }
                frame "ENL2_pre" {
                  n368 = call "BRig_RT__Case_Exp__State_ENLPre__v3.vi"("input_ENL2"=TRUE, "input_I_lick"=w1467, "input_dataTrial"=w1463, "input_dataCurrent"=w1464) -> ("output_dataTrial"=w1462:u16[][], "output_dataCurrent"=w1468:u16[], "output_state"=w1466:T2)  [unwired: 5 in]
                }
                frame "ENL1" {
                  n369 = call "BRig_RT__Case_Exp__State_ENL__v3.vi"("input_dataCurrent"=w1484, "input_dataTrial"=w1474, "input_ENL2"=FALSE, "input_arrTrig"=w1478, "input_state"=w1477, "I_lick"=w1476) -> ("output_l2_laserOn"=w1479:bool, "output_l2_laserEvent"=w1480:bool, "output_l1_laserOn"=w1481:bool, "output_state"=w1475:T2, "output_l1_laserEvent"=w1482:bool, "output_dataCurrent"=w1483:u16[], "output_dataTrial"=w1473:u16[][])  [unwired: 7 in]
                }
                frame "ENL2" {
                  n370 = call "BRig_RT__Case_Exp__State_ENL__v3.vi"("input_dataCurrent"=w1500, "input_dataTrial"=w1490, "input_ENL2"=TRUE, "input_arrTrig"=w1494, "input_state"=w1493, "I_lick"=w1492) -> ("output_l2_laserOn"=w1495:bool, "output_l2_laserEvent"=w1496:bool, "output_l1_laserOn"=w1497:bool, "output_state"=w1491:T2, "output_l1_laserEvent"=w1498:bool, "output_dataCurrent"=w1499:u16[], "output_dataTrial"=w1489:u16[][])  [unwired: 7 in]
                }
                frame "ENL1Penalty_pre" {
                  n371 = call "BRig_dataCurrent_c_generic.vi"() -> ("output_count_generic"=w1516:i32)  [unwired: 11 in]
                  n372 = call "BRig_dataCurrent_T_generic.vi"() -> ("output_T_generic"=w1514:i32)  [unwired: 11 in]
                  n373 = call "BRig_dataExp_T_ENLPenalty.vi"() -> ("output_ENL_penalty"=w1509:i32)  [unwired: 11 in]
                  n374 = Index Array(array=w1510, index=w1509) -> (element=w1513:u16)
                  n375 = Replace Array Subset(array=w1511, new element #1=u16 0 ("new element/subarray"), index #1=w1516, new element #2=w1513, index #2=w1514) -> (w1512:u16[])
                }
                frame "ENL1Penalty" {
                  n376 = call "BRig_RT__Case_Exp__generic__incrementCountTilThreshold.vi"("input_dataCurrent"=w1519) -> ("output_dataCurrent"=w1518:u16[], "output_underThreshold"=w1517:bool)  [unwired: 9 in]
                  n377 = Select(t=w1522, s=w1517, f=myRIO_BRig_RT__Case_Exp_stateList."ENL1_pre" ("Enum")) -> (s? t:f=w1520:T2)
                }
                frame "Cue1_pre" {
                  n378 = call "BRig_RT__Case_Exp__State_CuePre__v3.vi"("input_dataCurrent"=w1537, "input_dataTrial"=w1533, "input_Cue2"=FALSE ("input_ENL2"), "input_I_lick"=w1536, "input_dataExp"=w1534, "input_arrTrig"=w1530) -> ("output_state"=w1535:T2, "output_arrTrig"=w1529:bool[], "output_dataCurrent"=w1531:u16[], "output_dataTrial"=w1532:u16[][])  [unwired: 10 in]
                }
                frame "Cue2_pre" {
                  n379 = call "BRig_RT__Case_Exp__State_CuePre__v3.vi"("input_dataCurrent"=w1549, "input_dataTrial"=w1545, "input_Cue2"=TRUE ("input_ENL2"), "input_I_lick"=w1548, "input_dataExp"=w1546, "input_arrTrig"=w1542) -> ("output_state"=w1547:T2, "output_arrTrig"=w1541:bool[], "output_dataCurrent"=w1543:u16[], "output_dataTrial"=w1544:u16[][])  [unwired: 10 in]
                }
                frame "Cue1" {
                  n380 = call "BRig_RT__Case_Exp__State_Cue__v3.vi"("input_dataCurrent"=w1571, "input_dataTrial"=w1559, "input_dataExp"=w1553, "input_Cue2"=FALSE, "input_arrTrig"=w1567, "input_state"=w1569, "I_lick"=w1570) -> ("output_l2_laserOn"=w1563:bool, "output_l2_laserEvent"=w1564:bool, "output_SelectionState"=w1562:bool, "output_l1_laserOn"=w1565:bool, "output_state"=w1568:T2, "output_l1_laserEvent"=w1566:bool, "output_dataCurrent"=w1554:u16[], "output_dataTrial"=w1558:u16[][], "output_CueLed"=w1557:bool, "output_Audio_L"=w1556:bool, "output_Audio_R"=w1555:bool)  [unwired: 2 in]
                  n381 = case shown="True" w1562 {
                    selector: w1562 -> [_ w1577]
                    tunnel: w1561 -> [_ w1576]
                    tunnel: w1560 -> [_ w1575]
                    frame False {
                    }
                    frame True {
                      n382 = xnode "Read/Write Control"("FPGA VI Reference In"=w1575, "error in"=w1576, "SelectionState"=w1577) -> ("error out"=w1578:errorcluster)  [unwired: 1 out]
                      n383 = local write "error out"(w1578) -> ()
                    }
                  }
                }
                frame "Cue2" {
                  n384 = call "BRig_RT__Case_Exp__State_Cue__v3.vi"("input_dataCurrent"=w1598, "input_dataTrial"=w1586, "input_dataExp"=w1580, "input_Cue2"=TRUE, "input_arrTrig"=w1594, "input_state"=w1596, "I_lick"=w1597) -> ("output_l2_laserOn"=w1590:bool, "output_l2_laserEvent"=w1591:bool, "output_SelectionState"=w1589:bool, "output_l1_laserOn"=w1592:bool, "output_state"=w1595:T2, "output_l1_laserEvent"=w1593:bool, "output_dataCurrent"=w1581:u16[], "output_dataTrial"=w1585:u16[][], "output_CueLed"=w1584:bool, "output_Audio_L"=w1583:bool, "output_Audio_R"=w1582:bool)  [unwired: 2 in]
                  n385 = case shown="True" w1589 {
                    selector: w1589 -> [_ w1604]
                    tunnel: w1588 -> [_ w1603]
                    tunnel: w1587 -> [_ w1602]
                    frame False {
                    }
                    frame True {
                      n386 = xnode "Read/Write Control"("FPGA VI Reference In"=w1602, "error in"=w1603, "SelectionState"=w1604) -> ("error out"=w1605:errorcluster)  [unwired: 1 out]
                      n387 = local write "error out"(w1605) -> ()
                    }
                  }
                }
                frame "Cue1Penalty_pre" {
                  n388 = call "BRig_dataCurrent_c_generic.vi"() -> ("output_count_generic"=w1618:i32)  [unwired: 11 in]
                  n389 = call "BRig_dataCurrent_T_generic.vi"() -> ("output_T_generic"=w1616:i32)  [unwired: 11 in]
                  n390 = call "BRig_dataExp_T_CuePenalty.vi"() -> ("output_T_CuePenalty"=w1607:i32)  [unwired: 11 in]
                  n391 = Index Array(array=w1608, index=w1607) -> (element=w1606:u16)
                  n392 = Replace Array Subset(array=w1615, new element #1=u16 0 ("new element/subarray"), index #1=w1618, new element #2=w1606, index #2=w1616) -> (w1614:u16[])
                }
                frame "Cue1Penalty" {
                  n393 = call "BRig_RT__Case_Exp__generic__incrementCountTilThreshold.vi"("input_dataCurrent"=w1621) -> ("output_dataCurrent"=w1620:u16[], "output_underThreshold"=w1619:bool)  [unwired: 9 in]
                  n394 = Select(t=w1622, s=w1619, f=myRIO_BRig_RT__Case_Exp_stateList."ENL1_pre" ("Enum")) -> (s? t:f=w1623:T2)
                }
                frame "Selection_pre" {
                  n395 = xnode "Read/Write Control"("FPGA VI Reference In"=w1644, "error in"=w1645) -> ("error out"=w1643:errorcluster, "SelectReward"=w1640:bool, "SelectWrong"=w1641:bool)  [unwired: 1 out]
                  n396 = call "BRig_RT__Case_Exp__State_SelectPre.vi"("input_dataCurrent"=w1642, "input_SelectWrong"=w1641, "input_SelectReward"=w1640, "input_dataExp"=w1638, "input_LickL"=w1631, "input_LickR"=w1630, "input_arrTrig"=w1632) -> ("output_state"=w1639:T2, "output_dataCurrent"=w1637:u16[], "output_l1_laserEvent"=w1636:bool, "output_l1_laserOn"=w1635:bool, "output_l2_laserOn"=w1633:bool, "output_l2_laserEvent"=w1634:bool)  [unwired: 3 in]
                  n397 = local write "error out"(w1643) -> ()
                }
                frame "Selection" {
                  n398 = xnode "Read/Write Control"("FPGA VI Reference In"=w1669, "error in"=w1668) -> ("error out"=w1667:errorcluster, "SelectReward"=w1664:bool, "SelectWrong"=w1665:bool)  [unwired: 1 out]
                  n399 = call "BRig_RT__Case_Exp__State_Selection.vi"("input_state"=w1666, "input_dataCurrent"=w1659, "input_dataTrial"=w1650, "input_dataExp"=w1658, "input_arrTrig"=w1657, "input_FPGA_SelectWrong"=w1665, "input_FPGA_SelectReward"=w1664, "input_LickR"=w1663, "input_LickL"=w1662) -> ("output_LC_Laser_l2"=w1653:bool, "output_LC_Event_l2"=w1654:bool, "output_LC_Laser_l1"=w1655:bool, "output_LC_Event_l1"=w1656:bool, "output_state"=w1661:T2, "output_dataCurrent"=w1660:u16[], "output_dataTrial"=w1649:u16[][], "output_anySelect_L"=w1651:bool, "output_anySelect_R"=w1652:bool)  [unwired: 2 in]
                  n400 = local write "allReward_L"(w1651) -> ()
                  n401 = local write "allReward_R"(w1652) -> ()
                  n402 = local write "error out"(w1667) -> ()
                }
                frame "SelectReward_pre" {
                  n403 = call "BRig_RT__Case_Exp__State_RewardPre.vi"("input_dataCurrent"=w1691, "input_dataBlock"=w1690, "input_dataTrial"=w1681) -> ("output_T_Reward"=w1677:u16, "output_c_nReward_total_R"=w1686:u16, "output_c_nReward_total_L"=w1687:u16, "output_dataCurrent"=w1684:u16[], "output_dataBlock"=w1689:u16[][], "output_c_nReward_total"=w1685:u16, "output_nReward"=w1688:u16, "output_dataTrial"=w1680:u16[][])  [unwired: 5 in]
                  n404 = local read "FPGA_count2ms"() -> (w1676:dbl)
                  n405 = local write "nRewards_Right"(w1686) -> ()
                  n406 = local write "nRewards_Left"(w1687) -> ()
                  n407 = local write "nRewards_cur"(w1688) -> ()
                  n408 = local write "nRewards_total"(w1685) -> ()
                  n409 = To Double Precision Float(number=w1677) -> (double precision float=w1675:dbl)
                  n410 = Multiply(x=w1676, y=w1675) -> (x*y=w1673:dbl)
                  n411 = Round Toward +Infinity(x=w1673) -> (ceil(x): smallest int >= x=w1674:dbl)
                  n412 = call "BRig_RT_comm_tcp_write_RTwrite__RunState_Trial_selResult.vi"("input_dataTrial"=w1680, "iReward_or_iError"=TRUE, "input_dataCurrent"=w1684) -> ("output_strCmd"=w1682:string)  [unwired: 8 in]
                  n413 = To Unsigned Long Integer(number=w1674) -> (unsigned 32bit integer=w1672:u32)
                  n414 = xnode "Read/Write Control"("FPGA VI Reference In"=w1679, "error in"=w1678, "Solenoid_nTotal_L"=w1672, "Solenoid_nTotal_R"=w1672) -> ()  [unwired: 2 out]
                }
                frame "SelectReward" {
                  n415 = call "BRig_dataCurrent_c_generic.vi"() -> ("output_count_generic"=w1701:i32)  [unwired: 11 in]
                  n416 = call "BRig_RT__Case_Exp__State_Reward.vi"("input_dataCurrent"=w1702, "input_state"=w1706, "input_dataExp"=w1704) -> ("output_state"=w1705:T2, "output_dataCurrent"=w1707:u16[], "output__L"=w1699:bool, "output__R"=w1698:bool)  [unwired: 9 in]
                  n417 = Index Array(array=w1702, index=w1701) -> (element=w1700:u16)
                  n418 = Equal To 0?(x=w1700) -> (x = 0?=w1697:bool)
                  n419 = And(x=w1699, y=w1697) -> (x .and. y?=w1696:bool)
                  n420 = And(x=w1698, y=w1697) -> (x .and. y?=w1695:bool)
                }
                frame "SelectRewardPost_pre" {
                  n421 = call "BRig_dataExp_T_RewardPost.vi"() -> ("output_T_RewardPost"=w1711:i32)  [unwired: 11 in]
                  n422 = call "BRig_dataCurrent_c_generic.vi"() -> ("output_count_generic"=w1717:i32)  [unwired: 11 in]
                  n423 = call "BRig_dataCurrent_T_generic.vi"() -> ("output_T_generic"=w1716:i32)  [unwired: 11 in]
                  n424 = Index Array(array=w1712, index=w1711) -> (element=w1710:u16)
                  n425 = Replace Array Subset(array=w1714, new element #1=u16 0 ("new element/subarray"), index #1=w1717, new element #2=w1710, index #2=w1716) -> (w1713:u16[])
                }
                frame "SelectRewardPost" {
                  n426 = call "BRig_RT__Case_Exp__generic__incrementCountTilThreshold.vi"("input_dataCurrent"=w1724) -> ("output_dataCurrent"=w1722:u16[], "output_underThreshold"=w1723:bool)  [unwired: 9 in]
                  n427 = Select(t=w1726, s=w1723, f=myRIO_BRig_RT__Case_Exp_stateList."endTrial1" ("Enum")) -> (s? t:f=w1725:T2)
                }
                frame "SelectWrong_pre" {
                  n428 = call "BRig_RT__Case_Exp__State_WrongOrTimeout_Pre__v3.vi"("input_dataCurrent"=w1748, "input_WorTO"=FALSE, "input_dataBlock"=w1746, "input_dataTrial"=w1743, "input_dataExp"=w1744) -> ("output_BTPR"=w1737:bool, "output_T2R"=w1738:bool, "output_T2R_or_BTPR"=w1736:u16, "output_dataCurrent"=w1741:u16[], "output_dataBlock"=w1745:u16[][], "output_dataTrial"=w1740:u16[][], "output_BTPRavg"=w1732:dbl, "output_T2Ravg"=w1733:dbl, "output_R(F)_or_L(T)"=w1734:bool, "output_haveNewAvg"=w1735:bool)  [unwired: 1 in]
                  n429 = case shown="True" w1735 {
                    tunnel: w1734 -> [_ w1753]
                    tunnel: w1733 -> [_ w1752]
                    tunnel: w1732 -> [_ w1751]
                    frame False {
                    }
                    frame True {
                      n430 = case shown="False" w1753 {
                        tunnel: w1752 -> [w1754 w1757]
                        tunnel: w1751 -> [w1755 w1756]
                        frame False {
                          n431 = local write "BTPR_avg_R"(w1755) -> ()
                          n432 = local write "T2R_avg_R"(w1754) -> ()
                        }
                        frame True {
                          n433 = local write "BTPR_avg_L"(w1756) -> ()
                          n434 = local write "T2R_avg_L"(w1757) -> ()
                        }
                      }
                    }
                  }
                  n435 = case shown="True" w1738 {
                    tunnel: w1736 -> [_ w1758]
                    frame False {
                    }
                    frame True {
                      n436 = local write "T2R_block"(w1758) -> ()
                    }
                  }
                  n437 = case shown="True" w1737 {
                    tunnel: w1736 -> [_ w1759]
                    frame False {
                    }
                    frame True {
                      n438 = local write "BTPR_block"(w1759) -> ()
                    }
                  }
                  n439 = call "BRig_RT_comm_tcp_write_RTwrite__RunState_Trial_selResult.vi"("input_dataTrial"=w1740, "iReward_or_iError"=FALSE, "input_dataCurrent"=w1741) -> ("output_strCmd"=w1739:string)  [unwired: 8 in]
                }
                frame "SelectWrong" {
                  n440 = call "BRig_RT__Case_Exp__generic__incrementCountTilThreshold.vi"("input_dataCurrent"=w1762) -> ("output_dataCurrent"=w1760:u16[], "output_underThreshold"=w1761:bool)  [unwired: 9 in]
                  n441 = Select(t=w1764, s=w1761, f=myRIO_BRig_RT__Case_Exp_stateList."endTrial1" ("Enum")) -> (s? t:f=w1763:T2)
                }
                frame "SelectTimeout_pre" {
                  n442 = call "BRig_RT__Case_Exp__State_WrongOrTimeout_Pre__v3.vi"("input_dataCurrent"=w1786, "input_WorTO"=TRUE, "input_dataBlock"=w1785, "input_dataTrial"=w1784, "input_dataExp"=w1781) -> ("output_BTPR"=w1775:bool, "output_T2R"=w1776:bool, "output_T2R_or_BTPR"=w1774:u16, "output_dataCurrent"=w1779:u16[], "output_dataBlock"=w1783:u16[][], "output_dataTrial"=w1778:u16[][], "output_BTPRavg"=w1770:dbl, "output_T2Ravg"=w1771:dbl, "output_R(F)_or_L(T)"=w1772:bool, "output_haveNewAvg"=w1773:bool)  [unwired: 1 in]
                  n443 = xnode "Read/Write Control"("FPGA VI Reference In"=w1790, "error in"=w1789, "SelectionState"=FALSE) -> ("error out"=w1787:errorcluster)  [unwired: 1 out]
                  n444 = case shown="True" w1773 {
                    tunnel: w1772 -> [_ w1795]
                    tunnel: w1771 -> [_ w1794]
                    tunnel: w1770 -> [_ w1793]
                    frame False {
                    }
                    frame True {
                      n445 = case shown="False" w1795 {
                        tunnel: w1794 -> [w1796 w1799]
                        tunnel: w1793 -> [w1797 w1798]
                        frame False {
                          n446 = local write "BTPR_avg_R"(w1797) -> ()
                          n447 = local write "T2R_avg_R"(w1796) -> ()
                        }
                        frame True {
                          n448 = local write "BTPR_avg_L"(w1798) -> ()
                          n449 = local write "T2R_avg_L"(w1799) -> ()
                        }
                      }
                    }
                  }
                  n450 = local write "error out"(w1787) -> ()
                  n451 = call "BRig_RT_comm_tcp_write_RTwrite__RunState_Trial_selResult.vi"("input_dataTrial"=w1778, "iReward_or_iError"=FALSE, "input_dataCurrent"=w1779) -> ("output_strCmd"=w1777:string)  [unwired: 8 in]
                  n452 = case shown="True" w1775 {
                    tunnel: w1774 -> [_ w1801]
                    frame False {
                    }
                    frame True {
                      n453 = local write "BTPR_block"(w1801) -> ()
                    }
                  }
                  n454 = case shown="True" w1776 {
                    tunnel: w1774 -> [_ w1800]
                    frame False {
                    }
                    frame True {
                      n455 = local write "T2R_block"(w1800) -> ()
                    }
                  }
                }
                frame "SelectTimeout" {
                  n456 = call "BRig_RT__Case_Exp__generic__incrementCountTilThreshold.vi"("input_dataCurrent"=w1804) -> ("output_dataCurrent"=w1803:u16[], "output_underThreshold"=w1802:bool)  [unwired: 9 in]
                  n457 = Select(t=w1806, s=w1802, f=myRIO_BRig_RT__Case_Exp_stateList."endTrial1" ("Enum")) -> (s? t:f=w1805:T2)
                }
                frame "endTrial1" {
                  n458 = call "BRig_RT_comm_tcp_write_RTwrite__RunState_Trial_end.vi"("input_dataCurrent"=w1819) -> ("output_strCmd"=w1818:string)  [unwired: 10 in]
                  n459 = call "BRig_RT__Case_Exp__State_endTrial__v2.vi"("input_dataBlock"=w1815, "input_timeStamp_start"=w1820, "input_dataTrial"=w1827, "input_dataCurrent"=w1819) -> ("output_BTPRavg"=w1812:dbl, "output_T2Ravg"=w1813:dbl, "output_dataTrial"=w1826:u16[][], "output_dataCurrent"=w1821:u16[], "output_R(F)_or_L(T)"=w1814:bool, "output_runTime"=→"T_ExpRun_min":dbl)  [unwired: 2 in]
                  n460 = xnode "Read/Write Control"("FPGA VI Reference In"=w1823, "error in"=w1822, "SelectionState"=FALSE) -> ("error out"=w1824:errorcluster)  [unwired: 1 out]
                  n461 = case shown="False" w1814 {
                    tunnel: w1813 -> [w1830 w1833]
                    tunnel: w1812 -> [w1831 w1832]
                    frame False {
                      n462 = local write "BTPR_avg_R"(w1831) -> ()
                      n463 = local write "T2R_avg_R"(w1830) -> ()
                    }
                    frame True {
                      n464 = local write "BTPR_avg_L"(w1832) -> ()
                      n465 = local write "T2R_avg_L"(w1833) -> ()
                    }
                  }
                  n466 = local write "error out"(w1824) -> ()
                }
                frame "endTrial2" {
                  n467 = case shown="True" w1843 {
                    tunnel: [w1851 _] -> w1844
                    tunnel: [w1850 w1853] -> w1839
                    tunnel: w1838 -> [w1848 w1861]
                    tunnel: w1837 -> [w1849 w1859]
                    tunnel: [w1849 w1858] -> w1836
                    tunnel: [w1848 w1860] -> w1835
                    tunnel: w1834 -> [_ w1852]
                    frame False {
                      # "Receive commands"
                      n468 = call "BRig_RT__Case_Exp__UploadClosedLoop__v3.vi"() -> ("all rows"=w1851:i64[][], "output_haveCmd"=w1850:bool)  [unwired: 10 in]
                    }
                    frame True {
                      # "Parse commands and update"
                      n469 = Array Size(array=w1852) -> (size(s)=w1857:i32[])
                      n470 = Index Array(array=w1857, index=0) -> (element=w1855:i32)
                      n471 = Not Equal To 0?(x=w1855) -> (x != 0?=w1854:bool)
                      n472 = case shown="False" w1854 {
                        selector: w1854 -> [w1865 w1867]
                        tunnel: w1861 -> [w1863 w1871]
                        tunnel: [w1863 w1870] -> w1860
                        tunnel: w1859 -> [w1862 w1869]
                        tunnel: [w1862 w1868] -> w1858
                        tunnel: [w1865 w1867] -> w1853
                        tunnel: w1852 -> [_ w1866]
                        frame False {
                          w1864 = TRUE ("input_setValues")
                          # "Update"
                          n473 = call "BRig_RT_panel_cue_v0,90.vi"("input_setValues"=w1864, "input_dataExp"=w1863) -> ()  [unwired: 9 in, 1 out]
                          n474 = call "BRig_RT_panel_ExpStruct_v0,96.vi"("input_setValues"=w1864, "input_dataExp"=w1863) -> ()  [unwired: 9 in, 1 out]
                          n475 = call "BRig_RT_panel_Laser1_v0,90.vi"("input_setValues"=w1864, "input_dataExp"=w1863, "input_dataLC"=w1862) -> ()  [unwired: 7 in, 2 out]
                          n476 = call "BRig_RT_panel_Laser2_v0,90.vi"("input_setValues"=w1864, "input_dataExp"=w1863, "input_dataLC"=w1862) -> ()  [unwired: 7 in, 2 out]
                        }
                        frame True {
                          # "Parse"
                          n477 = call "BRig_RT__Case_Exp__UploadClosedLoop__updateSettings.vi"("input_newSettings"=w1866, "input_dataLC"=w1869, "input_dataExp"=w1871) -> ("output_dataLC"=w1868:u16[], "output_dataExp"=w1870:u16[])  [unwired: 7 in]
                        }
                      }
                    }
                  }
                  n478 = Select(t=myRIO_BRig_RT__Case_Exp_stateList."endTrial2", s=w1839, f=myRIO_BRig_RT__Case_Exp_stateList."endTrial3" ("Enum")) -> (s? t:f=w1840:T2)
                }
                frame "endTrial3" {
                  n479 = call "BRig_RT__Case_Exp__endTrial_checkFreeReward.vi"("input_dataBlock"=w1873, "input_dataExp"=w1882, "input_dataTrial"=w1883, "input_dataCurrent"=w1884) -> ("output_state"=w1874:T2, "output_endBlock"=w1872:bool)  [unwired: 6 in]
                  n480 = local read "STOP_endTrial"() -> (w1881:bool)
                  n481 = local read "STOP_abort"() -> (w1880:bool)
                  n482 = local read "START"() -> (w1878:bool)
                  n483 = Not(x=w1878) -> (.not. x?=w1879:bool)
                  n484 = Compound Arithmetic op=OR(w1881, w1879, w1880, w1872) -> (w1877:bool)
                  n485 = Select(t=myRIO_BRig_RT__Case_Exp_stateList."saveData_dataBlock" ("Enum"), s=w1877, f=w1874) -> (s? t:f=w1875:T2)
                }
                frame "endBlock" {
                  # "Get latest\nlaserSwitch"
                  n486 = call "BRig_dataExp_Loop_c_ExpStruct.vi"() -> ("output_Loop_c_ExpStruct"=w1893:i32)  [unwired: 11 in]
                  n487 = call "BRig_dataExp_LaserSwitch.vi"() -> ("output_LaserSwitch"=w1887:i32)  [unwired: 11 in]
                  n488 = local read "START"() -> (w1913:bool)
                  n489 = local read "STOP_endBlock"() -> (w1909:bool)
                  n490 = local read "STOP_endTrial"() -> (w1911:bool)
                  n491 = local read "STOP_abort"() -> (w1910:bool)
                  n492 = Replace Array Subset(array=w1894, new element=u16 2 ("new element/subarray"), index=w1893) -> (w1891:u16[])
                  n493 = call "BRig_RT_panel_ExpStruct_v0,96.vi"("input_setValues"=FALSE, "input_dataExp"=w1891) -> ("output_dataExp"=w1890:u16[])  [unwired: 9 in]
                  n494 = Index Array(array=w1890, index=w1887) -> (element=w1886:u16)
                  n495 = Not(x=w1913) -> (.not. x?=w1912:bool)
                  n496 = Select(t=myRIO_BRig_RT__Case_Exp_stateList."commUpload_dataTrial" ("Enum"), s=w1899, f=myRIO_BRig_RT__Case_Exp_stateList."initBlock" ("Enum")) -> (s? t:f=w1896:T2)
                  n497 = Replace Array Subset(array=w1889, new element=w1886, index=w1887) -> (w1888:u16[])
                  n498 = Compound Arithmetic op=OR(w1912, w1909, w1911, w1910) -> (w1903:bool)
                  n499 = Select(t=myRIO_BRig_RT__Case_Exp_stateList."endExp" ("Enum"), s=w1903, f=w1896) -> (s? t:f=w1914:T2)
                  n500 = Select(t="<S,E>" ("string"), s=w1903, f="") -> (s? t:f=w1900:string)
                }
                frame "endExp" {
                  n501 = xnode "Read/Write Control"("FPGA VI Reference In"=w1917, "error in"=w1916, "A6_Act"=FALSE) -> ("error out"=w1918:errorcluster)  [unwired: 1 out]
                  n502 = local write "error out"(w1918) -> ()
                }
                frame "commUpload_dataTrial" {
                }
                frame "saveData_dataBlock" {
                  n503 = Increment(x=w1948) -> (x+1=w1946:u16)
                  n504 = Replace Array Subset(array=w1940, new element=u16 2 ("new element/subarray"), index=0) -> (w1934:u16[])
                  n505 = Index Array(array=w1932, index (row)=0) -> (element=w1935:u16[])  [unwired: 1 in]
                  n506 = for {
                    tunnel: w1935 -> [w1958] mode=indexing
                    shift-right: [w1957] -> w1933
                    shift-left: w1934 -> [w1961]
                    i -> [w1960]
                    n507 = Increment(x=w1960) -> (x+1=w1959:i32)
                    n508 = Replace Array Subset(array=w1961, new element=w1958, index=w1959) -> (w1957:u16[])
                  }
                  n509 = RT FIFO Write(0:w1943, 1:w1933, 3:w1942) -> (11:w1945:errorcluster)  [unwired: 2 in, 3 out]
                  n510 = Unbundle By Name(w1945) -> ("code"=w1944:i32)
                  n511 = Greater?(x=w1946, y=u16 3) -> (0:w1954:bool)
                  n512 = Equal To 0?(x=w1944) -> (x = 0?=w1941:bool)
                  n513 = Or(x=w1954, y=w1941) -> (x .or. y?=w1953:bool)
                  n514 = Select(t=myRIO_BRig_RT__Case_Exp_stateList."endBlock" ("Enum"), s=w1953, f=w1949) -> (s? t:f=w1947:T2)
                }
                frame "saveData_dataTrial" {
                  n515 = Increment(x=w1979) -> (x+1=w1978:u16)
                  n516 = Replace Array Subset(array=w1964, new element=u16 1 ("new element/subarray"), index=0) -> (w1968:u16[])
                  n517 = Index Array(array=w1963, index (row)=0) -> (element=w1969:u16[])  [unwired: 1 in]
                  n518 = for {
                    tunnel: w1969 -> [w1988] mode=indexing
                    shift-right: [w1987] -> w1967
                    shift-left: w1968 -> [w1991]
                    i -> [w1990]
                    n519 = Increment(x=w1990) -> (x+1=w1989:i32)
                    n520 = Replace Array Subset(array=w1991, new element=w1988, index=w1989) -> (w1987:u16[])
                  }
                  n521 = RT FIFO Write(0:w1966, 1:w1967, 3:w1965) -> (11:w1974:errorcluster)  [unwired: 2 in, 3 out]
                  n522 = Unbundle By Name(w1974) -> ("code"=w1973:i32)
                  n523 = Equal To 0?(x=w1973) -> (x = 0?=w1962:bool)
                  n524 = Greater?(x=w1978, y=u16 3) -> (0:w1976:bool)
                  n525 = Or(x=w1976, y=w1962) -> (x .or. y?=w1975:bool)
                  n526 = Select(t=myRIO_BRig_RT__Case_Exp_stateList."endTrial2" ("Enum"), s=w1975, f=w1980) -> (s? t:f=w1981:T2)
                }
                frame "dummyState" {
                  n527 = call "BRig_dataCurrent_iTrial.vi"() -> ("output_iTrial"=w1998:i32)  [unwired: 11 in]
                  n528 = Index Array(array=w1999, index=w1998) -> (element=w1997:u16)
                  n529 = Equal?(x=w1997, y=u16 1) -> (x = y?=w1995:bool)
                  n530 = Equal To 0?(x=w2006) -> (x = 0?=w2007:bool)
                  n531 = Select(t=u16 13, s=w1995, f=u16 15) -> (s? t:f=w1992:u16)
                  n532 = Select(t=w1992, s=w2007, f=w2006) -> (s? t:f=w2005:u16)
                  n533 = Decrement(x=w2005) -> (x-1=w2004:u16)
                  n534 = Equal To 0?(x=w2004) -> (x = 0?=w2003:bool)
                  n535 = Select(t=myRIO_BRig_RT__Case_Exp_stateList."initTrial" ("Enum"), s=w2003, f=w2001) -> (s? t:f=w2000:T2)
                }
                frame "dummyState_endBlock" {
                  n536 = call "BRig_dataCurrent_iTrial.vi"() -> ("output_iTrial"=w2022:i32)  [unwired: 11 in]
                  n537 = Index Array(array=w2016, index=w2022) -> (element=w2012:u16)
                  n538 = Equal?(x=w2012, y=u16 1) -> (x = y?=w2020:bool)
                  n539 = Equal To 0?(x=w2013) -> (x = 0?=w2024:bool)
                  n540 = Select(t=u16 1, s=w2020, f=u16 3) -> (s? t:f=w2017:u16)
                  n541 = Select(t=w2017, s=w2024, f=w2013) -> (s? t:f=w2023:u16)
                  n542 = Decrement(x=w2023) -> (x-1=w2014:u16)
                  n543 = Equal To 0?(x=w2014) -> (x = 0?=w2015:bool)
                  n544 = Select(t=myRIO_BRig_RT__Case_Exp_stateList."initBlock" ("Enum"), s=w2015, f=w2026) -> (s? t:f=w2025:T2)
                }
                frame "FreeReward_pre" {
                  w2056 = u16 0 ("new element/subarray")
                  # "Duration = MTrig duration"
                  # "Duration = Reward Time"
                  n545 = call "BRig_dataCurrent_FreeReward_c.vi"() -> ("output_FreeReward_c"=w2057:i32)  [unwired: 11 in]
                  n546 = call "BRig_dataCurrent_iSpout.vi"() -> ("output_iSpout"=w2054:i32)  [unwired: 11 in]
                  n547 = call "BRig_dataTrial_T_Reward.vi"() -> ("output_T_Reward"=w2058:i32)  [unwired: 11 in]
                  n548 = call "BRig_dataCurrent_c_generic.vi"() -> ("output_count_generic"=w2063:i32)  [unwired: 11 in]
                  n549 = call "BRig_dataCurrent_T_generic.vi"() -> ("output_T_generic"=w2062:i32)  [unwired: 11 in]
                  n550 = Index Array(array=w2055, index=w2054) -> (element=w2053:u16)
                  n551 = call "BRig_dataMTrig_Solenoid_T_L.vi"() -> ("output_Solenoid_T_L"=w2052:i32)  [unwired: 11 in]
                  n552 = call "BRig_dataMTrig_Solenoid_T_R.vi"() -> ("output_Solenoid_T_R"=w2051:i32)  [unwired: 11 in]
                  n553 = Equal To 0?(x=w2053) -> (x = 0?=w2033:bool)
                  n554 = local read "FPGA_count2ms"() -> (w2045:dbl)
                  n555 = Select(t=w2052, s=w2033, f=w2051) -> (s? t:f=w2049:i32)
                  n556 = Index Array(array=w2059, index (row)=0 ("disabled index (row)"), index (col)=w2058) -> ()  [unwired: 1 out]
                  n557 = Index Array(array=w2050, index=w2049) -> (element=w2044:u16)
                  n558 = Replace Array Subset(array=w2055, new element #1=w2056, index #1=w2057, new element #2=w2056, index #2=w2063, new element #3=w2044, index #3=w2062) -> (w2061:u16[])
                  n559 = To Double Precision Float(number=w2044) -> (double precision float=w2048:dbl)
                  n560 = call "BRig_dataExp_FreeReward_c_L.vi"() -> ("output_FreeReward_c_L"=w2038:i32)  [unwired: 11 in]
                  n561 = call "BRig_dataExp_FreeReward_c_R.vi"() -> ("output_FreeReward_c_R"=w2039:i32)  [unwired: 11 in]
                  n562 = Multiply(x=w2045, y=w2048) -> (x*y=w2046:dbl)
                  n563 = Select(t=w2038, s=w2033, f=w2039) -> (s? t:f=w2035:i32)
                  n564 = Round Toward +Infinity(x=w2046) -> (ceil(x): smallest int >= x=w2047:dbl)
                  n565 = Index Array(array=w2036, index=w2035) -> (element=w2034:u16)
                  n566 = To Unsigned Long Integer(number=w2047) -> (unsigned 32bit integer=w2041:u32)
                  n567 = xnode "Read/Write Control"("FPGA VI Reference In"=w2043, "error in"=w2042, "Solenoid_nTotal_L"=w2041, "Solenoid_nTotal_R"=w2041) -> ()  [unwired: 2 out]
                  n568 = Increment(x=w2034) -> (x+1=w2032:u16)
                  n569 = case shown="False" w2033 {
                    tunnel: w2032 -> [w2066 w2067]
                    frame True {
                      n570 = local write "FreeReward_c_L"(w2066) -> ()
                    }
                    frame False {
                      n571 = local write "FreeReward_c_R"(w2067) -> ()
                    }
                  }
                  n572 = Replace Array Subset(array=w2036, new element=w2032, index=w2035) -> (w2037:u16[])
                }
                frame "FreeReward" {
                  n573 = call "BRig_dataCurrent_iSpout.vi"() -> ("output_iSpout"=w2078:i32)  [unwired: 11 in]
                  n574 = call "BRig_dataCurrent_c_generic.vi"() -> ("output_count_generic"=w2072:i32)  [unwired: 11 in]
                  n575 = Index Array(array=w2079, index #1=w2078, index #2=w2072) -> (element #1=w2077:u16, element #2=w2071:u16)
                  n576 = Equal To 0?(x=w2077) -> (x = 0?=w2075:bool)
                  n577 = Equal To 0?(x=w2071) -> (x = 0?=w2070:bool)
                  n578 = Not(x=w2075) -> (.not. x?=w2076:bool)
                  n579 = call "BRig_RT__Case_Exp__generic__incrementCountTilThreshold.vi"("input_dataCurrent"=w2079) -> ("output_dataCurrent"=w2080:u16[], "output_underThreshold"=w2069:bool)  [unwired: 9 in]
                  n580 = Select(t=w2083, s=w2069, f=myRIO_BRig_RT__Case_Exp_stateList."FreeRewardPost_pre" ("Enum")) -> (s? t:f=w2081:T2)
                  n581 = And(x=w2069, y=w2070) -> (x .and. y?=w2068:bool)
                  n582 = And(x=w2068, y=w2075) -> (x .and. y?=w2073:bool)
                  n583 = And(x=w2068, y=w2076) -> (x .and. y?=w2074:bool)
                }
                frame "FreeRewardPost" {
                  n584 = call "BRig_RT__Case_Exp__generic__incrementCountTilThreshold.vi"("input_dataCurrent"=w2090) -> ("output_dataCurrent"=w2089:u16[], "output_underThreshold"=w2088:bool)  [unwired: 9 in]
                  n585 = Select(t=w2093, s=w2088, f=myRIO_BRig_RT__Case_Exp_stateList."initTrial" ("Enum")) -> (s? t:f=w2091:T2)
                }
                frame "FreeRewardPost_pre" {
                  n586 = call "BRig_dataExp_T_RewardPost.vi"() -> ("output_T_RewardPost"=w2103:i32)  [unwired: 11 in]
                  n587 = call "BRig_dataCurrent_c_generic.vi"() -> ("output_count_generic"=w2106:i32)  [unwired: 11 in]
                  n588 = call "BRig_dataCurrent_T_generic.vi"() -> ("output_T_generic"=w2105:i32)  [unwired: 11 in]
                  n589 = Index Array(array=w2100, index=w2103) -> (element=w2102:u16)
                  n590 = Replace Array Subset(array=w2101, new element #1=u16 0 ("new element/subarray"), index #1=w2106, new element #2=w2102, index #2=w2105) -> (w2099:u16[])
                }
              }
              n591 = call "BRig_RT_panel_manualTriggering_v0,90.vi"("input_dataMTrig"=w1193) -> ("output_Solenoid_R"=w1204:bool, "output_Solenoid_L"=w1203:bool, "output_dataMTrig"=w1236:u16[], "output_Audio_L"=w1235:bool, "output_Audio_R"=w1234:bool, "output_CueLed"=w1232:bool, "output_Laser_l1"=w1208:bool, "output_Laser_l2"=w1228:bool)  [unwired: 11 in]
              n592 = call "BRig_RT__Case_Exp__comm_tcp__data_other.vi"("input_strState"=w1196, "input_strAccum"=w1197, "input_error"=w1198, "input_hTCP"=w1199, "input_I_connected_TCP"=w1200) -> ("output_strAccum"=w1179:string, "output_error"=w1178:errorcluster, "output_hTCP"=w1180:refnum<k5>, "output_I_connect_TCP"=w1181:bool)  [unwired: 3 in]
              n593 = Or(x="STOP_abort", y=w1220) -> (x .or. y?=w1182:bool)
              n594 = Or(x=w1233, y=w1232) -> (x .or. y?=w1211:bool)
              n595 = local read "Laser1_LED"() -> (w1169:bool)
              n596 = local read "Laser2_LED"() -> (w1168:bool)
              n597 = Or(x=w1235, y=w1250) -> (x .or. y?=w1210:bool)
              n598 = Or(x=w1249, y=w1234) -> (x .or. y?=w1209:bool)
              n599 = Or(x=w1207, y=w1208) -> (x .or. y?=w1227:bool)
              n600 = Or(x=w1231, y=w1228) -> (x .or. y?=w1229:bool)
              n601 = call "BRig_RT__Case_Exp__recordLick.vi"("input_dataLick"=w1219, "input_lick__R"=w1213, "input_lick__L"=w1214, "input_lick"=w1215, "intput_state__trialStart"=w1173, "intput_state__trialEnd"=w1218, "input_dataCurrent"=w1217) -> ("output_dataLick"=w1212:u16[][], "output_dataCurrent"=w1216:u16[])  [unwired: 7 in]
              n602 = xnode "Read/Write Control"("FPGA VI Reference In"=w1248, "error in"=w1247, "L1Led_ON"=w1169, "L2Led_ON"=w1168, "Solenoid_trig_L"=w1202, "Solenoid_trig_R"=w1201, "A3_SL"=w1203, "A1_SR"=w1204, "LC_Event_l1"=w1226, "LC_Laser_l1"=w1227, "LC_Event_l2"=w1230, "LC_Laser_l2"=w1229, "CueLed_Event"=w1211, "audioTrigger_L"=w1210, "audioTrigger_R"=w1209) -> ("FPGA VI Reference Out"=w1254:refnum<k20>, "error out"=w1253:errorcluster, "fpga_laser1"=w1167:bool, "fpga_laser2"=w1166:bool, "fpga_solenoid_L"=w1165:bool, "fpga_solenoid_R"=w1164:bool, "AnaIn_0"=w1194:i16, "AnaIn_1"=w1195:i16)
              n603 = local write "Laser1"(w1167) -> ()
              n604 = local write "Laser2"(w1166) -> ()
              n605 = local write "Solenoid L"(w1165) -> ()
              n606 = local write "Solenoid R"(w1164) -> ()
              n607 = call "BRig_RT__Case_Exp__recordAnalogInput__PortC__fifo__1value.vi"("input_iOccurence"=w1224, "resetOccurrence"=w1223, "input_dataCurrent"=w1217, "input_iState_start"=w1173, "rt fifo"=w1172, "input_iState_end"=w1218, "input_fifo_error"=w1171, "input_AI1"=w1195, "input_AI0"=w1194) -> ("output_fifo_error"=w1177:errorcluster, "output_iOccurrence"=w1225:u16)  [unwired: 8 in, 1 out]
              n608 = call "BRig_RT_timeLoop_Exp__noStateLimit.vi"("input_error"=w1177, "input_Threshold_reset"="input_Threshold_reset", "input_Threshold"=w1239, "input_timestamp"=w1240, "input_state"=w1173) -> ("output_Threshold"=w1237:bool, "output_duration"=→"tLoop":dbl)  [unwired: 4 in, 1 out]
              "Threshold" <- w1237
              n609 = node-c288() -> ()  [unwired: 1 in, 1 out]
            }
            "stop_TimedLoop" <- w866
            n610 = while {
              tunnel: w808 -> [w934]
              tunnel: w807 -> [w933]
              shift-right: [w928] -> _
              shift-left: 0 ("element") -> [w929]
              shift-right: [w924] -> _
              shift-left: w813 -> [w930]
              tunnel: [w927] -> w810
              tunnel: [w926] -> w809
              tunnel: w806 -> [w923]
              tunnel: w805 -> [w922]
              tunnel: [w921] -> w804
              tunnel: [w920] -> w803
              shift-right: [w918] -> _
              shift-left: FALSE -> [w919]
              stop <- w917 stop-if-true
              # "timed out?"
              n611 = RT FIFO Read(0:w934, 3:w933) -> (8:w927:refnum<k33>, 9:w931:u16, 10:w938:bool, 11:w935:errorcluster)  [unwired: 2 in, 1 out]
              n612 = Unbundle By Name(w935) -> ("code"=w939:i32)
              n613 = Not(x=w938) -> (.not. x?=w937:bool)
              n614 = Equal To 0?(x=w939) -> (x = 0?=w936:bool)
              n615 = And(x=w936, y=w937) -> (x .and. y?=w932:bool)
              n616 = Select(t=w935, s=w936, f=w933) -> (s? t:f=w926:errorcluster)
              n617 = case shown="True" w932 {
                tunnel: w931 -> [_ w970]
                tunnel: w930 -> [w962 w972]
                tunnel: w929 -> [w961 w969]
                tunnel: [w962 w971] -> w924
                tunnel: [w961 w965] -> w928
                tunnel: [_ w963] -> w925
                frame False {
                }
                frame True {
                  n618 = Replace Array Subset(array=w972, new element=w970, index=w969) -> (w971:u16[])
                  n619 = Increment(x=w969) -> (x+1=w967:i32)
                  n620 = Less?(x=w969, y=7 ("dimension size")) -> (x < y?=w964:bool)
                  n621 = Select(t=w967, s=w964, f=0) -> (s? t:f=w965:i32)
                  n622 = Not(x=w964) -> (.not. x?=w963:bool)
                }
              }
              n623 = case shown="True" w925 {
                tunnel: w924 -> [_ w951]
                tunnel: w923 -> [w942 w950]
                tunnel: w922 -> [w941 w949]
                tunnel: [w942 w947] -> w921
                tunnel: [w941 w946] -> w920
                tunnel: w919 -> [w940 w944]
                tunnel: [w940 w943] -> w918
                frame False {
                }
                frame True {
                  n624 = for {
                    N: 8 -> [_]
                    tunnel: w951 -> [w958] mode=indexing
                    tunnel: w950 -> [w960]
                    tunnel: w949 -> [w959]
                    shift-right: [w953] -> w945
                    shift-left: FALSE -> [w957]
                    tunnel: [w956] -> w947
                    tunnel: [w955] -> w946
                    n625 = shared-variable-write(w960, w959, w958) -> (w956:refnum<k21>, w955:errorcluster, w954:bool)  [unwired: 1 in]
                    n626 = Or(x=w957, y=w954) -> (x .or. y?=w953:bool)
                  }
                  n627 = Or(x=w944, y=w945) -> (x .or. y?=w943:bool)
                }
              }
              n628 = local read "stop_TimedLoop"() -> (w917:bool)
            }
            n629 = while {
              shift-right: [w1032] -> _
              shift-left: 0 -> [w1021]
              tunnel: w863 -> [w1039]
              tunnel: w855 -> [w1041]
              shift-right: [w1028] -> _
              shift-left: 0 -> [w1023]
              shift-right: [w1033] -> _
              shift-left: w829 -> [w1040]
              shift-right: [w1029] -> _
              shift-left: w828 -> [w1042]
              shift-right: [w1036] -> w852
              shift-left: w822 -> [w1049]
              shift-right: [w1037] -> w845
              shift-left: w821 -> [w1043]
              tunnel: w825 -> [w1026]
              tunnel: w830 -> [w1025]
              stop <- w1050 stop-if-true
              # "nColumns dataBlock"
              # "nColumns dataTrial"
              # "buffer_dataTrial"
              # "buffer_dataBlock"
              # "buffer_dataTrial"
              # "buffer_dataBlock"
              n630 = local read "stop_TimedLoop"() -> (w1050:bool)
              n631 = Not Equal To 0?(x=w1023) -> (x != 0?=w1024:bool)
              n632 = case shown="True" w1024 {
                tunnel: w1042 -> [w1125 w1128]
                tunnel: w1023 -> [w1126 w1130]
                tunnel: w1041 -> [_ w1139]
                tunnel: [w1126 w1127] -> w1030
                tunnel: [w1125 w1128] -> w1031
                frame False {
                }
                frame True {
                  n633 = Array Subset(array=w1128, length (row)=w1130) -> (w1141:u16[][])  [unwired: 3 in]
                  n634 = call "BRig_dataBlock_iBlock.vi"() -> ("output_iBlock"=w1136:i32)  [unwired: 11 in]
                  n635 = Index Array(array=w1128, index (row)=0, index (col)=w1136) -> (element=w1135:u16)
                  n636 = To Double Precision Float(number=w1141) -> (double precision float=w1140:dbl[][])
                  n637 = Not Equal?(x=u16 1, y=w1135) -> (x != y?=w1133:bool)
                  n638 = call-poly <vilib>:"Write To Spreadsheet File.vi"("delimiter (\\t)"="," ("delimiter (\\t)"), "append to file? (new file:F)"=w1133, "2D data"=w1140, "file path (dialog if empty)"=w1139) -> ("new file path (Not A Path if cancelled)"=w1132:path)  [unwired: 4 in]
                  n639 = call <vilib>:"Is Path and Not Empty.vi"("path"=w1132) -> ("Is Path and Not Empty?"=w1131:bool)  [unwired: 4 in]
                  n640 = Select(t=0, s=w1131, f=w1130) -> (s? t:f=w1127:i32)
                }
              }
              n641 = RT FIFO Read(0:w1049, 3:w1043) -> (8:w1036:refnum<k33>, 9:w1027:u16[], 10:w1047:bool, 11:w1044:errorcluster)  [unwired: 2 in, 1 out]
              n642 = Unbundle By Name(w1044) -> ("code"=w1048:i32)
              n643 = Not(x=w1047) -> (.not. x?=w1046:bool)
              n644 = Equal To 0?(x=w1048) -> (x = 0?=w1045:bool)
              n645 = And(x=w1045, y=w1046) -> (x .and. y?=w1038:bool)
              n646 = Select(t=w1044, s=w1045, f=w1043) -> (s? t:f=w1037:errorcluster)
              n647 = Not Equal To 0?(x=w1021) -> (x != 0?=w1022:bool)
              n648 = case shown="True" w1022 {
                tunnel: w1040 -> [w1108 w1111]
                tunnel: w1021 -> [w1109 w1113]
                tunnel: w1039 -> [_ w1122]
                tunnel: [w1109 w1110] -> w1034
                tunnel: [w1108 w1111] -> w1035
                frame False {
                }
                frame True {
                  n649 = Array Subset(array=w1111, length (row)=w1113) -> (w1124:u16[][])  [unwired: 3 in]
                  n650 = call "BRig_dataTrial_nTrial.vi"() -> ("output_nTrial"=w1119:i32)  [unwired: 11 in]
                  n651 = Index Array(array=w1111, index (row)=0, index (col)=w1119) -> (element=w1118:u16)
                  n652 = To Double Precision Float(number=w1124) -> (double precision float=w1123:dbl[][])
                  n653 = Not Equal?(x=u16 1, y=w1118) -> (x != y?=w1116:bool)
                  n654 = call-poly <vilib>:"Write To Spreadsheet File.vi"("delimiter (\\t)"="," ("delimiter (\\t)"), "append to file? (new file:F)"=w1116, "2D data"=w1123, "file path (dialog if empty)"=w1122) -> ("new file path (Not A Path if cancelled)"=w1115:path)  [unwired: 4 in]
                  n655 = call <vilib>:"Is Path and Not Empty.vi"("path"=w1115) -> ("Is Path and Not Empty?"=w1114:bool)  [unwired: 4 in]
                  n656 = Select(t=0, s=w1114, f=w1113) -> (s? t:f=w1110:i32)
                }
              }
              n657 = case shown="True" w1038 {
                tunnel: w1035 -> [w1055 w1065]
                tunnel: w1034 -> [w1054 w1063]
                tunnel: [w1055 w1064] -> w1033
                tunnel: [w1054 w1062] -> w1032
                tunnel: w1031 -> [w1053 w1061]
                tunnel: w1030 -> [w1052 w1059]
                tunnel: [w1053 w1060] -> w1029
                tunnel: [w1052 w1058] -> w1028
                tunnel: w1027 -> [_ w1068]
                tunnel: w1026 -> [_ w1057]
                tunnel: w1025 -> [_ w1056]
                frame False {
                  n658 = Wait (ms)(milliseconds to wait=u32 10) -> ()  [unwired: 1 out]
                }
                frame True {
                  n659 = Index Array(array=w1068, index=0) -> (element=w1066:u16)
                  n660 = Not Equal To 0?(x=w1066) -> (x != 0?=w1067:bool)
                  n661 = case shown="True" w1067 {
                    tunnel: w1068 -> [_ w1084]
                    tunnel: w1066 -> [_ w1087]
                    tunnel: w1065 -> [w1073 w1077]
                    tunnel: [w1073 w1076] -> w1064
                    tunnel: w1063 -> [w1072 w1075]
                    tunnel: [w1072 w1074] -> w1062
                    tunnel: w1061 -> [w1071 w1081]
                    tunnel: [w1071 w1079] -> w1060
                    tunnel: w1059 -> [w1070 w1080]
                    tunnel: [w1070 w1078] -> w1058
                    tunnel: w1057 -> [_ w1083]
                    tunnel: w1056 -> [_ w1082]
                    frame False {
                    }
                    frame True {
                      n662 = Equal?(x=u16 1 ("y"), y=w1087) -> (x = y?=w1085:bool)
                      n663 = case shown="False" w1085 {
                        tunnel: w1084 -> [w1095 w1107]
                        tunnel: w1083 -> [w1093 _]
                        tunnel: w1082 -> [_ w1102]
                        tunnel: w1081 -> [w1097 w1101]
                        tunnel: w1080 -> [w1096 w1103]
                        tunnel: [w1097 w1100] -> w1079
                        tunnel: [w1096 w1099] -> w1078
                        tunnel: w1077 -> [w1092 w1104]
                        tunnel: [w1090 w1104] -> w1076
                        tunnel: w1075 -> [w1089 w1098]
                        tunnel: [w1088 w1098] -> w1074
                        frame True {
                          n664 = Array Subset(array=w1095, index=1, length=w1093) -> (w1091:u16[])
                          n665 = Increment(x=w1089) -> (x+1=w1088:i32)
                          n666 = Replace Array Subset(array=w1092, new element=w1091, index (row)=w1089) -> (w1090:u16[][])  [unwired: 1 in]
                        }
                        frame False {
                          n667 = Array Subset(array=w1107, index=1, length=w1102) -> (w1105:u16[])
                          n668 = Increment(x=w1103) -> (x+1=w1099:i32)
                          n669 = Replace Array Subset(array=w1101, new element=w1105, index (row)=w1103) -> (w1100:u16[][])  [unwired: 1 in]
                        }
                      }
                    }
                  }
                }
              }
            }
            n670 = node-c288(w915) -> ()  [unwired: 1 out]
            n671 = RT FIFO Delete(0:w852, 2:TRUE ("force destroy? (F)"), 3:w845) -> ()  [unwired: 1 out]
            n672 = RT FIFO Delete(0:w810, 2:TRUE ("force destroy? (F)"), 3:w809) -> ()  [unwired: 1 out]
            n673 = flat-sequence {
              tunnel: w886 -> [w1143]
              tunnel: w885 -> [w1146]
              tunnel: w884 -> [w1145]
              tunnel: w883 -> [w1144]
              tunnel: w882 -> [w1148]
              tunnel: w880 -> [_]
              tunnel: w801 -> [w1150]
              tunnel: w850 -> [w1149]
              tunnel: [w1142] -> w861
              tunnel: w845 -> [_]
              tunnel: w879 -> [w1161]
              tunnel: w878 -> [w1160]
              tunnel: w877 -> [w1159]
              tunnel: [w1158] -> w876
              tunnel: [w1157] -> w875
              tunnel: [w1152] -> w871
              tunnel: w861 -> [w1151]
              frame #0 {
                # "Store"
                n674 = call "BRig_RT__Case_Exp__storeData__endExp__v5__p1.vi"("input_dataCurrent"=w1144, "input_dataLC"=w1149, "input_dataExp"=w1150, "input_dataExp_end"=w1145, "input_dataLC_end"=w1146) -> ("output_True"=w1147:bool)  [unwired: 10 in]
                n675 = call "BRig_RT__Case_Exp__storeData__endExp__v5__p2.vi"("input_dataCurrent"=w1144, "input_dataLick"=w1148, "input_True"=w1147, "input_dataMTrig"=w1143) -> ("output_True"=w1142:bool)  [unwired: 11 in]
              }
              frame #1 {
                # "Send"
                n676 = local read "Data Set Prefix"() -> (w1153:string)
                n677 = call "BRig_RT_comm_webdav_upload_all__v3.vi"("input_I_connected_webdav"=w1159, "input_fileName_prefix"=w1153, "input_hSession"=w1160, "input_error"=w1161, "input_True"=w1151) -> ("output_hSession"=w1157:T4, "error out"=w1158:errorcluster, "output_nFilenames"=w1154:i32, "output_arrFilenames"=w1155:string[], "output_uploaded"=w1156:bool[], "output_strCmd"=w1152:string)  [unwired: 5 in]
                n678 = call "BRig_RT_comm_webdav_upload_all_warnUser.vi"("input_n"=w1154, "input_arrFilenames"=w1155, "input_arrUploaded"=w1156) -> ()  [unwired: 9 in]
              }
            }
            n679 = flat-sequence {
              tunnel: w895 -> [w1162]
              tunnel: [w1162] -> w881
              frame #0 {
                w1163 = FALSE ("START")
                n680 = local write "START"(w1163) -> ()
                n681 = local write "STOP_endTrial"(w1163) -> ()
                n682 = local write "STOP_endBlock"(w1163) -> ()
              }
            }
            n683 = xnode "Read/Write Control"("FPGA VI Reference In"=w912, "error in"=w881, "Counts_Reset"=TRUE, "audioTrigger_L"=w898, "audioFreq_L_kHz"=w896, "audioAmp_L"=w897, "audioTrigger_R"=w898, "audioFreq_R_kHz"=w896, "audioAmp_R"=w897, "A3_SL"=w898, "A1_SR"=w898, "A6_Act"=w898) -> ("FPGA VI Reference Out"=w911:refnum<k20>, "error out"=w880:errorcluster)
            n684 = call "BRig_RT__Case_Exp__comm_tcp__data_other.vi"("input_strState"=w871, "input_strAccum"="" ("f"), "input_error"=w872, "input_hTCP"=w873, "input_I_connected_TCP"=w874) -> ("output_error"=w867:errorcluster, "output_hTCP"=w868:refnum<k5>, "output_I_connect_TCP"=w869:bool)  [unwired: 3 in, 1 out]
          }
        }
        n685 = local read "STOP_abort"() -> (w311:bool)
      }
    }
  }
  n686 = flat-sequence {
    tunnel: w89 -> [w2121]
    tunnel: w88 -> [w2123]
    tunnel: w82 -> [w2122]
    tunnel: [w2122] -> w94
    tunnel: [w2121] -> w93
    tunnel: [w2120] -> w92
    tunnel: w67 -> [w2119]
    tunnel: [w2119] -> w91
    tunnel: w68 -> [w2118]
    tunnel: [w2118] -> w90
    tunnel: w75 -> [w2116]
    tunnel: w74 -> [w2115]
    tunnel: w73 -> [w2114]
    tunnel: w69 -> [w2117]
    tunnel: [w2117] -> w87
    tunnel: w86 -> [_]
    tunnel: [w2116] -> w81
    tunnel: [w2115] -> w80
    tunnel: [w2114] -> w79
    tunnel: w94 -> [w2143]
    tunnel: w93 -> [w2142]
    tunnel: w92 -> [w2141]
    tunnel: [w2140] -> _
    tunnel: w91 -> [w2139]
    tunnel: w90 -> [w2138]
    tunnel: w87 -> [w2137]
    tunnel: w81 -> [w2136]
    tunnel: w80 -> [w2135]
    tunnel: w79 -> [w2134]
    frame #0 {
      # "Stop FPGA\nSend QUIT to Host"
      n687 = case shown="True" w2122 {
        tunnel: w2121 -> [_ w2132]
        tunnel: w2123 -> [w2129 w2131]
        tunnel: [w2129 w2130] -> w2120
        frame False {
        }
        frame True {
          n688 = xnode "Read/Write Control"("FPGA VI Reference In"=w2132, "error in"=w2131, "FPGA_Stop"=TRUE) -> ("error out"=w2130:errorcluster)  [unwired: 1 out]
        }
      }
      n689 = case shown="True" w2116 {
        tunnel: w2115 -> [_ w2128]
        tunnel: w2114 -> [_ w2127]
        frame False {
        }
        frame True {
          w2124 = "<S,Q><S,Q><S,Q><S,Q>" ("input_packet")
          n690 = call "BRig_RT_comm_tcp_write_RTwrite.vi"("input_error"=w2127, "input_packet"=w2124, "input_hTCP"=w2128) -> ("output_error"=w2126:errorcluster, "output_hTCP"=w2125:refnum<k5>)  [unwired: 5 in, 2 out]
          n691 = call "BRig_RT_comm_tcp_write_RTwrite.vi"("input_error"=w2126, "input_packet"=w2124, "input_hTCP"=w2125) -> ()  [unwired: 5 in, 4 out]
        }
      }
    }
    frame #1 {
      # "Disconnect FPGA\nDisconnect comm webdav"
      n692 = case shown="True" w2143 {
        tunnel: w2141 -> [w2148 w2151]
        tunnel: w2142 -> [_ w2150]
        tunnel: [w2148 w2149] -> w2140
        frame False {
        }
        frame True {
          n693 = xnode "Close FPGA VI Reference"("FPGA VI Reference In"=w2150, "error in"=w2151) -> ("error out"=w2152:errorcluster)
          n694 = call <vilib>:"Reset myRIO.vi"("error in (no error)"=w2152) -> ("error out"=w2149:errorcluster)  [unwired: 10 in]
        }
      }
      n695 = case shown="True" w2136 {
        tunnel: w2135 -> [_ w2145]
        tunnel: w2134 -> [_ w2144]
        frame False {
        }
        frame True {
          n696 = TCP Close Connection(connection ID=w2145, error in (no error)=w2144) -> ()  [unwired: 1 in, 2 out]
        }
      }
      n697 = case shown="True" w2139 {
        tunnel: w2138 -> [_ w2147]
        tunnel: w2137 -> [_ w2146]
        frame False {
        }
        frame True {
          n698 = call <vilib>:"Close Session.vi"("session handle"=w2147, "error in (no error)"=w2146) -> ()  [unwired: 13 in, 1 out]
        }
      }
    }
  }
  n699 = Flush Stream(8:w6, 11:w7) -> (0:w8:errorcluster, 3:w9:refnum<k21>)  [unwired: 2 in, 1 out]
  n700 = Destroy Stream Endpoint(8:w8, 11:w9) -> ()  [unwired: 1 out]
